vi "MainKinetics Calibration.vi"() -> ()   [LabVIEW 2017]
uses:
  <vilib>/Utility/miscctls.llb/LVRowAndColumnTypeDef.ctl
  <vilib>/Utility/sysdir.llb/System Directory Type.ctl
  <vilib>/Utility/config.llb/Read Key (String).vi
  <vilib>/Utility/config.llb/Write Key (String).vi
  <vilib>/Utility/cursorutil.llb/Set Cursor (Icon Pict).vi
  PCAN_Driver/ControlCAN.lvlib
  <vilib>/Utility/config.llb/NI_LVConfig.lvlib
panel:
  out "AO[0] 2":sgl
  out "AO[0] 1":sgl
  out "RO[1]":string
  out "AO[1]":string
  out "CC":dbl
  out "AO[0]":sgl
  out "SN From File":string
  out "ProductRev":string
  out "UUT In":u16(ring)=4 items=["BLDC  60A  P/N: 1"=1, "BLDC  30A  P/N: 2"=2, "Warrior 60A P/N: 3"=3, "Condenser Merkava P/N: 4"=4, "Condenser India P/N: 4"=5]
  out "G.Stop":bool
  out "STDBY":bool
  out "CurrentSens":bool
  out "CurrentOut":dbl
  out "Current":string
  out "VISA Current":refnum<visa-resource-name>
  out "Offset":dbl
  out "Analogtest":bool=TRUE
  out "TestinExecution":string
  out "FullSpeed2 Current":dbl
  out "FullSpeed1 Current":dbl
  out "User":string
  out "ParamVersion":string
  out "DSP Board S/N":string
  out "POWER Board S/N":string caption="DRIVER Board S/N"
  in  "EventTimeout":i32=100
  out "SpeedLimit":dbl[](array[numeric])
  out "TestArray":string[](array[string])
  out "Motor Speed RPM Serial":dbl
  out "DAQmx Device Name":tag
  out "PN":string
  out "FileName":string
  out "VenableSpeed":u16
  out "TesterVersion":string
  out "ClosePanel":bool=TRUE
  out "UUT SN Report":string
  out "Automation":bool
  out "Test Failed":bool
  out "VisualInspectionResult":bool
  out "MotorTempResult":bool
  out "VenableDirectionResult":bool
  out "VenableResult":bool
  out "ComTestResult":bool=TRUE
  out "UUT SoftwareVer":string
  out "Next SN":i32
  in  "SetSN":bool
  out "Current SN":i32
  out "FullSpeed2 Speed":dbl
  out "FullSpeed2 Current":dbl
  out "FullSpeed1 Current":dbl
  out "FullSpeed1 Speed":dbl
  out "UUT":u8
  out "CAN Status":bool
  out "Array":u64[][](array[numeric]) format="%016x"
  out "Motor Phase Current RMS":dbl
  out "Ambient Temperature":dbl
  out "Speed error":bool
  out "Commutation err":bool
  out "Under voltage/Over voltage":bool
  out "Derated drive temp":bool
  out "Motor Over temperature":bool
  out "Motor Sensor temp Fauilre":bool
  out "Drive Over temperature":bool
  out "Drive Sensor temp Failure":bool
  out "Ambient Over temp":bool
  out "Ambient Sensor temp":bool
  out "DC Voltage":dbl
  out "DC Current":dbl
  out "Power transistor Heat sink Temp.":dbl
  out "Motor Stator Temp.":dbl
  out "Motor Speed RPM":dbl
  out "ECS State":u16
  out "UUT":string="EBAY"
  in  "Logger Path":path
  in  "Report":bool
  in  "Start":bool
  in  "ATR":string[][](table)=[["Test Communication", "-", "-", "-", "-", ""], ["Set S/N", "-", "-", "-", "-", ""], ["Set Board Number", "-", "-", "-", "-", ""], [" ", "", "", "", "", ""], ["Test Communication", "-", "-", "-", "-", ""], ["Get S/N", "-", "-", "-", "", ""], ["Get Board Number", "-", "-", "-", "", ""], ["Get FW", "-", "-", "-", "", ""], ["Enable Motor", "", "", "", "", ""], ["Small position command", "", "", "", "", ""], ["Measure delta", "", "", "", "", ""], ["Velocity command", "", "", "", "", ""]]
  in  "Settings":bool
  in  "Refresh Button":bool
  out "Serial Status":bool
  in  "VISA Kinetics":refnum<visa-resource-name>="COM6"
  in  "Serial Com":bool
  in  "Help Button":bool
  out "Pannel User Message":string
  in  "Stop Button":bool
  # "Kinetics"
  # "REDLER TECHNOLOGIES LTD"
  # "ver 1.2p"
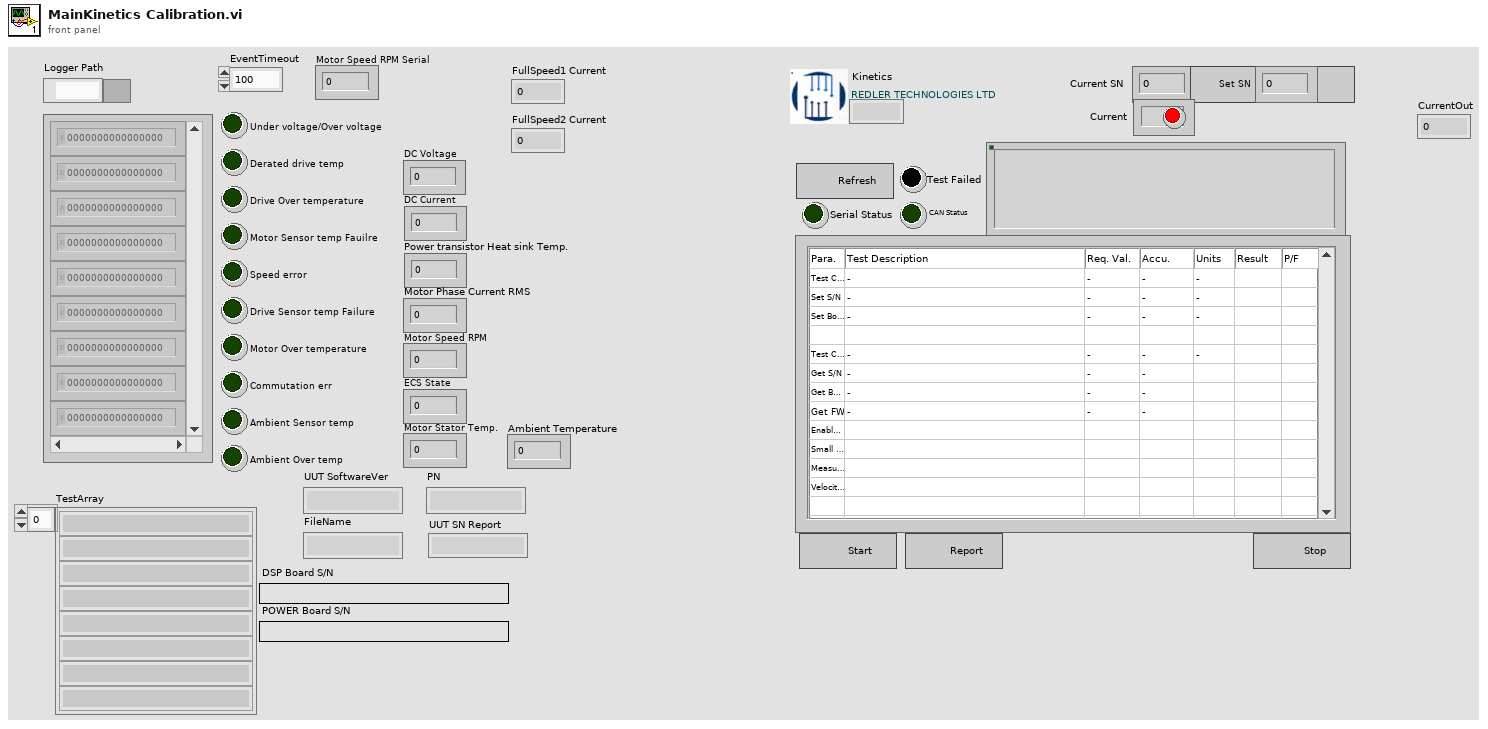
[diagram p1: front panel]
types:
  T1 = enum8{"Enabled", "Disabled", "Disabled and Grayed Out"}
  T2 = cluster{"VISA":refnum<visa-resource-name>, "TestArray":string[]}
  T3 = cluster{"ID":u32, "MSGTYPE":u8, "LEN":u8, "aDATA":u8[]}[]
  T4 = enum16{"Erase ATR Table", "Stop", "MainProgram", "Initialize"}
  T5 = typedef "NI_LVConfig.lvlib/Config Data RefNum.ctl" = refnum<k1>
  T6 = enum16{"Init", "0 ohm", "6 ohm", "13.2 ohm", "15 ohm", "25.9 ohm", "33 ohm", "Down", "Up", "Venable", "Firmware", "PowerSuply"}
  T7 = enum16{"Wait", "Exit", "VC=0", "ReadVC", "VC=1000"}
  T8 = enum16{"Stop", "Result", "FullSpeed2", "MD[1]=1", "FullSpeed1", "MD[1]=0"}
  T9 = enum16{"K15", "K16", "K17", "Venable", "Firmeware", "Fan", "Power", "120C", "110C", "100C", "90C", "80C", "70C", "60C", "50C", "40C", "30C", "25C", "20C", "10C", "0C"}
  T10 = enum8{"Term1", "Term2", "Current", "Fan", "TempCPU"}
  T11 = enum16{"Exit", "AI0/3", "AO0", "Wait", "Read", "Init"}
  T12 = enum16{"Exit", "Wait", "ReadCurrent", "ReadTemp", "Init"}
  T13 = enum16{"Init", "0 ohm", "6 ohm", "13.2 ohm", "15 ohm", "25.9 ohm", "33 ohm", "Down", "Up", "Venable", "Firmware", "PowerSuply"}[]
  T14 = typedef "LVRowAndColumnTypeDef.ctl" = cluster{"Row":i32, "Column":i32}
  T15 = enum32{"Invalid", "Standard", "Closed", "Hidden", "Minimized", "Maximized"}
  T16 = cluster{"ID":u32, "MSGTYPE":u8, "LEN":u8, "aDATA":u8[]}
  T17 = enum16{"open", "replace", "create", "open or create", "replace or create", "replace or create with confirmation"}
  T18 = typedef "ControlCAN.lvlib/DevType.ctl" = u32
  T19 = typedef "ControlCAN.lvlib/CAN Channel.ctl" = u32
  T20 = typedef "ControlCAN.lvlib/VCI_INIT_CONFIG.ctl" = cluster{"AccCode":u32, "AccMask":u32, "InitFlag":T21, "Fliter":T22, "Timing0":u8, "Timing1":u8, "Mode":T23}
  T21 = typedef "ControlCAN.lvlib/InitFlag.ctl" = u32
  T22 = typedef "ControlCAN.lvlib/Fliter.ctl" = u8
  T23 = typedef "ControlCAN.lvlib/Mode.ctl" = u8
  T24 = cluster{"DevType":T18, "DevIndex":u32, "CanIndex":T19, "VCI_INIT_CONFIG":T20}
  T25 = typedef "ControlCAN.lvlib/VCI_CAN_OBJ.ctl" = cluster{"ID":u32, "TimeStamp":u32, "TimeFlag":u8, "SendType":u8, "RemoteFlag":u8, "ExternFlag":u8, "DataLen":u8, "Data":u8[], "Reserved":u8[]}
  T26 = cluster{"Type":enum16{"接收", "发送"}, "Channel":T19, "Time":timestamp, "VCI_CAN_OBJ":T25}[]
  T27 = cluster{"Type":enum16{"接收", "发送"}, "Channel":T19, "Time":timestamp, "VCI_CAN_OBJ":T25}
  T28 = typedef "LVPoint32TypeDef.ctl" = cluster{"Horizontal":i32, "Vertical":i32}
  T29 = typedef "System Directory Type.ctl" = i32
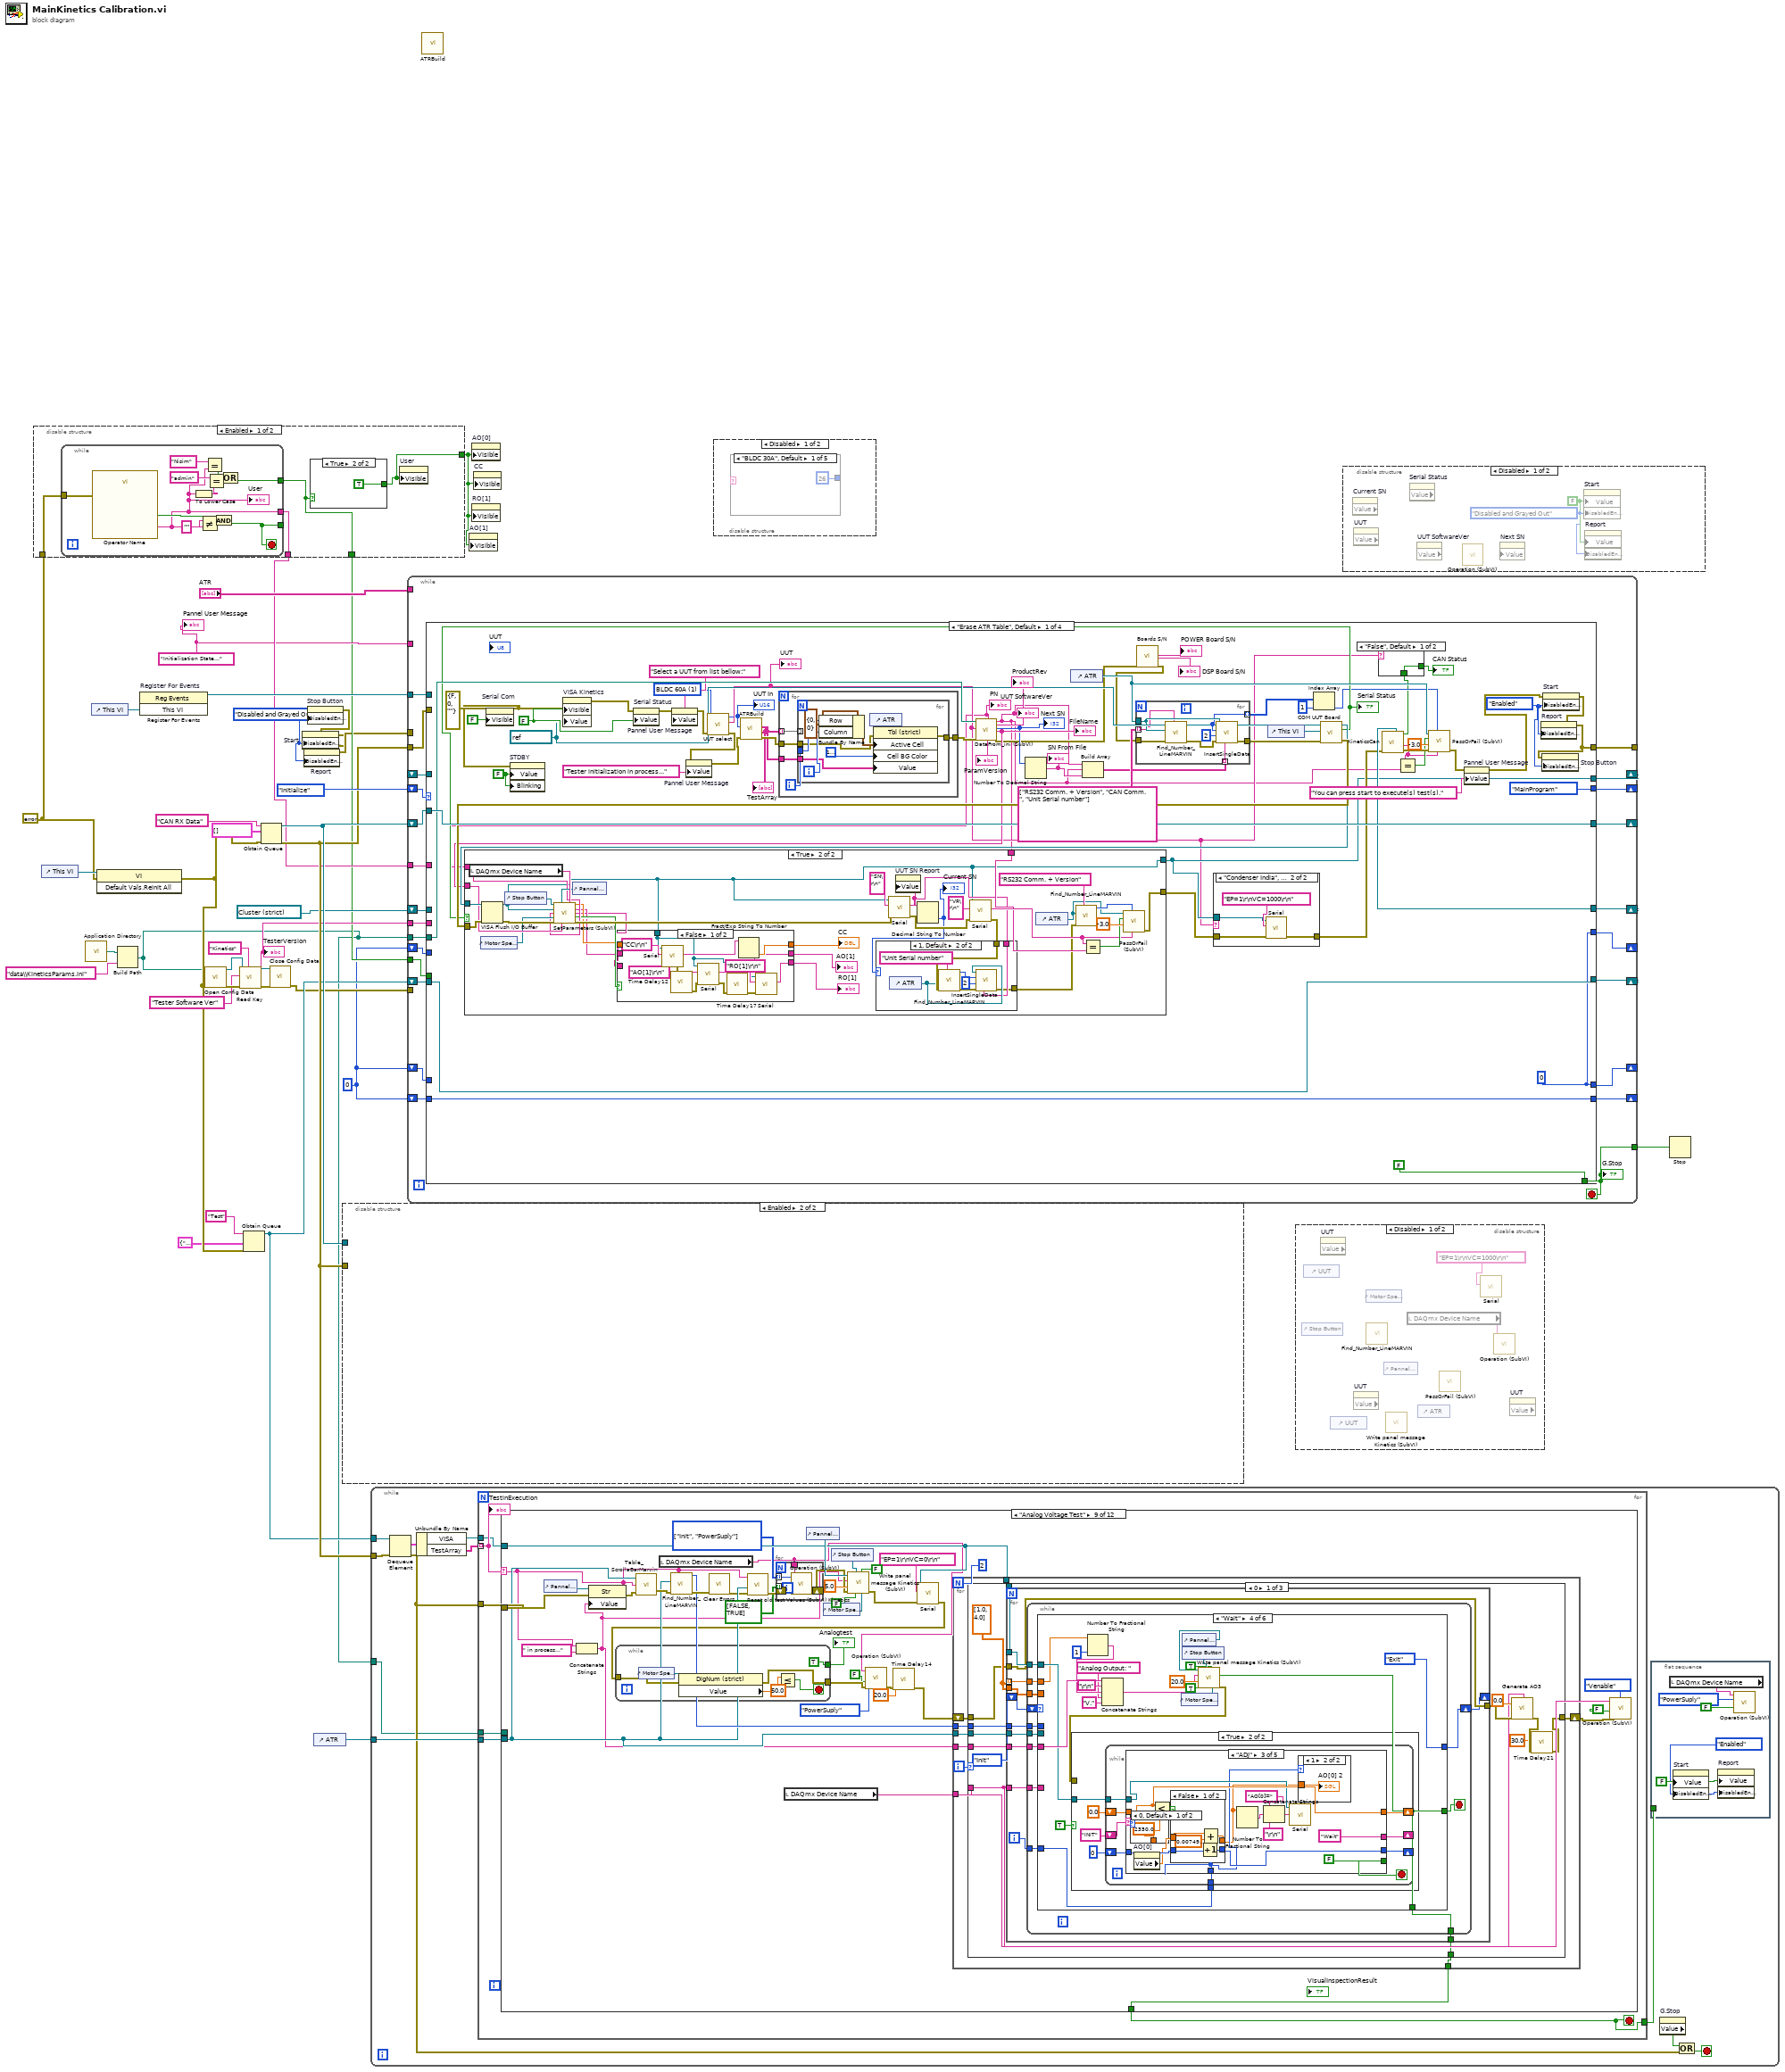
[diagram p0: block diagram]
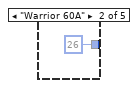
[diagram p2: hidden frame]
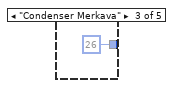
[diagram p3: hidden frame]
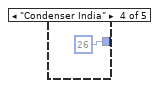
[diagram p4: hidden frame]
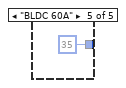
[diagram p5: hidden frame]
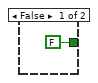
[diagram p7: hidden frame]
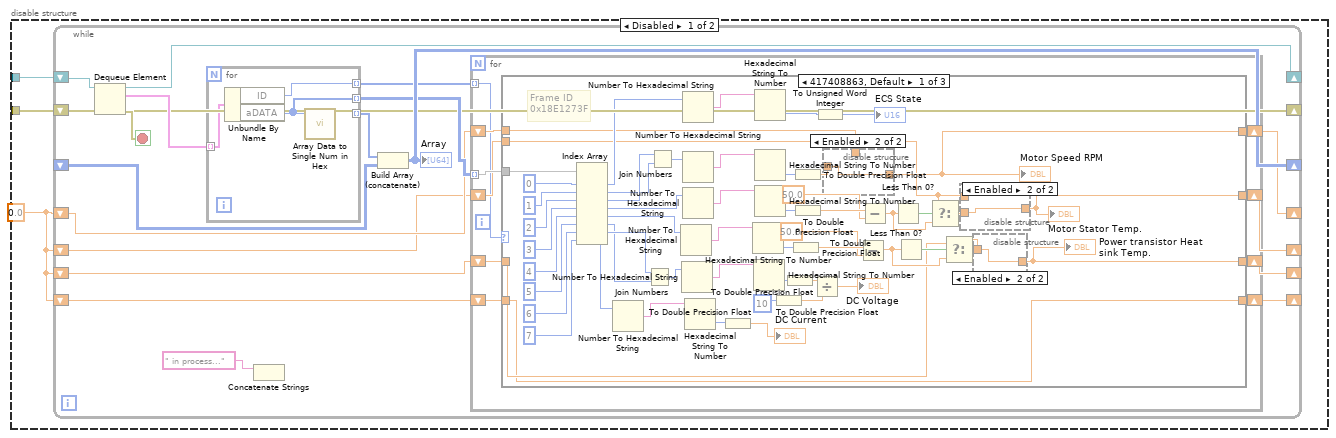
[diagram p9: hidden frame]
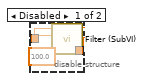
[diagram p10: hidden frame]
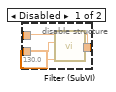
[diagram p11: hidden frame]
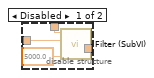
[diagram p12: hidden frame]
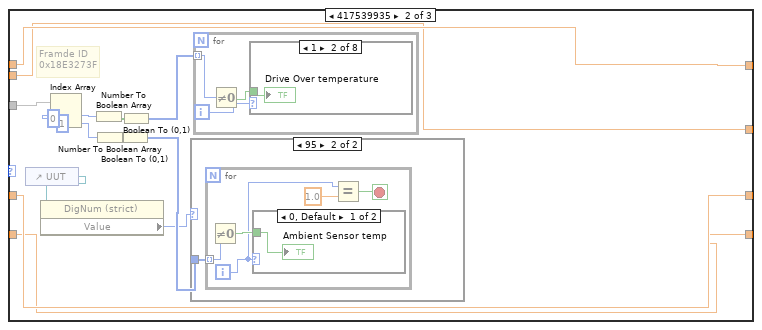
[diagram p13: hidden frame]
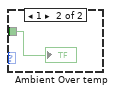
[diagram p15: hidden frame]
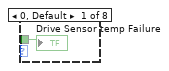
[diagram p16: hidden frame]
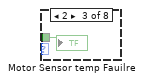
[diagram p17: hidden frame]
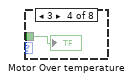
[diagram p18: hidden frame]
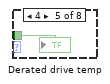
[diagram p19: hidden frame]
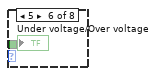
[diagram p20: hidden frame]
diagram:
  w2 = T1."Disabled and Grayed Out" ("Disabled")
  w23 = "Initialization State..."
  w9 = 0
  w12 = errorcluster {"status"=FALSE, "code"=0, "source"=""} ("error in (no error)")
  n1 = disable-structure shown="Enabled" {
    disable-tunnel: [w41 _] -> w24
    disable-tunnel: w12 -> [w40 _]
    disable-tunnel: [w39 _] -> w10
    disable-tunnel: [w38 _] -> w1
    frame Enabled {
      n2 = while {
        tunnel: [w52] -> _
        tunnel: [w45] -> w41
        tunnel: [w50] -> w39
        tunnel: w40 -> [w47]
        stop <- w52 stop-if-true
        n3 = call "Operator Name"("error in (no error)"=w47) -> ("Operator Name"=w45:string, "OK"=w53:bool)  [unwired: 16 in, 1 out]
        "User" <- w45
        n4 = To Lower Case(string=w45) -> (all lower case string=w44:string)
        n5 = Not Equal?(x=w45, y="") -> (x != y?=w54:bool)
        n6 = Equal?(x="Nisim", y=w45) -> (x = y?=w48:bool)
        n7 = Equal?(x="admin", y=w44) -> (x = y?=w51:bool)
        n8 = And(x=w53, y=w54) -> (x .and. y?=w52:bool)
        n9 = Or(x=w48, y=w51) -> (x .or. y?=w50:bool)
      }
      n10 = case shown="True" w39 {
        tunnel: [FALSE TRUE] -> w38
        frame False {
        }
        frame True {
        }
      }
      n11 = property on="User" class="Str"("Visible"=w38) -> ()  [unwired: 2 in, 2 out]
    }
    frame Disabled {
    }
  }
  n12 = control-ref of="This VI"() -> (w13:refnum<vi>)
  n13 = call <vilib>:"Application Directory.vi"() -> ("Application Directory"=w28:path)
  n14 = control-ref of="This VI"() -> (w26:refnum<vi>)
  n15 = invoke class="VI" method="Default Vals.Reinit All"(reference=w13, error in=w12) -> (error out=w11:errorcluster)  [unwired: 1 in, 2 out]
  n16 = Build Path(base path=w28, name or relative path="data\\KineticsParams.ini") -> (appended path=w6:path)
  n17 = register-events "Register For Events"(w26) -> (reference out=w25:refnum<event-registration>)  [unwired: 2 in, 1 out]
  n18 = call <vilib>:"Open Config Data.vi"("error in (no error)"=w11, "configuration file path"=w6) -> ("error out"=w21:errorcluster, "refnum"=w20:T5)  [unwired: 1 in, 7 out]
  n19 = call-poly <vilib>:"Read Key.vi"("section"="Kinetics", "error in (no error)"=w21, "key"="Tester Software Ver", "refnum"=w20) -> ("error out"=w18:errorcluster, "value"=w14:string, "refnum out"=w17:T5)  [unwired: 2 in, 3 out]
  "TesterVersion" <- w14
  n20 = Obtain Queue(name (unnamed)="Test", element data type=T2 {"VISA"="COM1", "TestArray"=[]}, error in (no error)=w11) -> (queue out=w31:refnum<queue>)  [unwired: 2 in, 2 out]
  n21 = Obtain Queue(name (unnamed)="CAN RX Data", element data type=T3 [], error in (no error)=w11) -> (queue out=w34:refnum<queue>, error out=w32:errorcluster)  [unwired: 2 in, 1 out]
  n22 = call <vilib>:"Close Config Data.vi"("error in (no error)"=w18, "refnum"=w17) -> ("error out"=w16:errorcluster)  [unwired: 8 in, 1 out]
  n23 = property on="Stop Button" class="Bool (strict)"("DisabledEnum"=w2) -> (error out=w3:errorcluster)  [unwired: 2 in, 1 out]
  n24 = property on="Start" class="Bool (strict)"(error in=w3, "DisabledEnum"=w2) -> (error out=w4:errorcluster)  [unwired: 1 in, 1 out]
  n25 = property on="Report" class="Bool (strict)"(error in=w4, "DisabledEnum"=w2) -> (error out=w5:errorcluster)  [unwired: 1 in, 1 out]
  n26 = control-ref of="ATR"() -> (w22:refnum<vi>)
  n27 = disable-structure shown="Enabled" {
    disable-tunnel: w34 -> [w58 _]
    disable-tunnel: w32 -> [w57 _]
    frame Disabled {
      w56 = 0.0
      n28 = while {
        shift-right: [w75] -> _
        shift-left: w58 -> [w77]
        shift-right: [w73] -> _
        shift-left: _ -> [w74]
        shift-right: [w69] -> _
        shift-left: w57 -> [w69]
        shift-right: [w67] -> _
        shift-left: w56 -> [w68]
        shift-right: [w66] -> _
        shift-left: w56 -> [w65]
        shift-right: [w64] -> _
        shift-left: w56 -> [w63]
        shift-right: [w62] -> _
        shift-left: w56 -> [w61]
        stop <- w76 stop-if-true
        n29 = Dequeue Element(queue=w77, error in (no error)=w69) -> (queue out=w75:refnum<queue>, element=w70:T3, error out=w76:errorcluster)  [unwired: 1 in, 1 out]
        n30 = for {
          tunnel: [w223] -> w72 mode=indexing
          tunnel: w70 -> [w222] mode=indexing
          tunnel: [w221] -> w71 mode=indexing
          tunnel: [w220] -> w60 mode=indexing
          n31 = Unbundle By Name(w222) -> ("ID"=w220:u32, "aDATA"=w221:u8[])
          n32 = call "Array Data to Single Num in Hex.vi"("aDATA"=w221) -> ("Numeric"=w223:u64)  [unwired: 10 in]
        }
        n33 = Concatenate Strings(" in process..." ("Strin")) -> ()  [unwired: 1 in, 1 out]
        n34 = Build Array (concatenate)(w72, w74) -> (w73:u64[][])
        "Array" <- w73
        n35 = for {
          tunnel: w71 -> [w87] mode=indexing
          shift-right: [w85] -> w67
          shift-left: w68 -> [w86]
          shift-right: [w84] -> w66
          shift-left: w65 -> [w83]
          shift-right: [w82] -> w64
          shift-left: w63 -> [w81]
          shift-right: [w80] -> w62
          shift-left: w61 -> [w79]
          tunnel: w60 -> [w78] mode=indexing
          n36 = case shown="417408863, Default" w78 {
            tunnel: w87 -> [w124 w172 w210]
            tunnel: w86 -> [w98 w161 w199]
            tunnel: [w97 w161 w199] -> w85
            tunnel: [w94 w160 w198] -> w84
            tunnel: w83 -> [w93 w160 w198]
            tunnel: [w90 w159 w197] -> w82
            tunnel: w81 -> [w89 w159 w197]
            tunnel: [w88 w158 w193] -> w80
            tunnel: w79 -> [w88 w158 w192]
            frame 417408863, Default {
              # "Frame ID\n0x18E1273F"
              n37 = Index Array(array=w124, index #1=0 ("index"), index #2=1 ("index"), index #3=2 ("index"), index #4=3 ("index"), index #5=4 ("index"), index #6=5 ("index"), index #7=6 ("index"), index #8=7 ("index")) -> (element #1=w108:u8, element #2=w110:u8, element #3=w111:u8, element #4=w115:u8, element #5=w118:u8, element #6=w122:u8, element #7=w123:u8, element #8=w121:u8)
              n38 = Number To Hexadecimal String(2:w121) -> (0:w135:string)  [unwired: 1 in]
              n39 = Join Numbers(hi=w123, lo=w122) -> ((hi.lo)=w142:u16)
              n40 = Join Numbers(hi=w111, lo=w110) -> ((hi.lo)=w112:u16)
              n41 = Number To Hexadecimal String(2:w118) -> (0:w119:string)  [unwired: 1 in]
              n42 = Number To Hexadecimal String(2:w142) -> (0:w141:string)  [unwired: 1 in]
              n43 = Number To Hexadecimal String(2:w108) -> (0:w109:string)  [unwired: 1 in]
              n44 = Number To Hexadecimal String(2:w112) -> (0:w113:string)  [unwired: 1 in]
              n45 = Number To Hexadecimal String(2:w115) -> (0:w116:string)  [unwired: 1 in]
              n46 = Hexadecimal String To Number(string=w135) -> (number=w134:u32)  [unwired: 2 in, 1 out]
              n47 = To Double Precision Float(number=w134) -> (double precision float=→"DC Current":dbl)
              n48 = Hexadecimal String To Number(string=w119) -> (number=w120:u32)  [unwired: 2 in, 1 out]
              n49 = Hexadecimal String To Number(string=w141) -> (number=w140:u32)  [unwired: 2 in, 1 out]
              n50 = Hexadecimal String To Number(string=w109) -> (number=w106:u32)  [unwired: 2 in, 1 out]
              n51 = Hexadecimal String To Number(string=w113) -> (number=w114:u32)  [unwired: 2 in, 1 out]
              n52 = Hexadecimal String To Number(string=w116) -> (number=w117:u32)  [unwired: 2 in, 1 out]
              n53 = To Double Precision Float(number=u32 10 ("y")) -> (double precision float=w138:dbl)
              n54 = To Double Precision Float(number=w140) -> (double precision float=w137:dbl)
              n55 = To Double Precision Float(number=w120) -> (double precision float=w103:dbl)
              n56 = To Double Precision Float(number=w114) -> (double precision float=w99:dbl)
              n57 = To Double Precision Float(number=w117) -> (double precision float=w105:dbl)
              n58 = Divide(x=w137, y=w138) -> (x/y=→"DC Voltage":dbl)
              n59 = To Unsigned Word Integer(number=w106) -> (unsigned 16bit integer=→"ECS State":u16)
              n60 = disable-structure shown="Enabled" {
                disable-tunnel: w99 -> [w156 w157]
                disable-tunnel: w98 -> [w155 _]
                disable-tunnel: [w153 w157] -> w97
                frame Disabled {
                  n61 = call "Filter (SubVI).vi"("Delta"=5000.0, "NewVal"=w156, "OldVal"=w155) -> ("Val"=w153:dbl)  [unwired: 8 in]
                }
                frame Enabled {
                }
              }
              "Motor Speed RPM" <- w97
              n62 = Subtract(x=w103, y=50.0 ("x")) -> (x-y=w92:dbl)
              n63 = Subtract(x=w105, y=50.0 ("x")) -> (x-y=w95:dbl)
              n64 = Less Than 0?(x=w95) -> (x < 0?=w101:bool)
              n65 = Less Than 0?(x=w92) -> (x < 0?=w100:bool)
              n66 = Select(t=w93, s=w101, f=w95) -> (s? t:f=w96:dbl)
              n67 = Select(t=w89, s=w100, f=w92) -> (s? t:f=w91:dbl)
              n68 = disable-structure shown="Enabled" {
                disable-tunnel: w96 -> [w151 w152]
                disable-tunnel: [w150 w152] -> w94
                disable-tunnel: w93 -> [w149 _]
                frame Disabled {
                  n69 = call "Filter (SubVI).vi"("Delta"=130.0, "NewVal"=w151, "OldVal"=w149) -> ("Val"=w150:dbl)  [unwired: 8 in]
                }
                frame Enabled {
                }
              }
              "Motor Stator Temp." <- w94
              n70 = disable-structure shown="Enabled" {
                disable-tunnel: w91 -> [w146 w147]
                disable-tunnel: [w144 w147] -> w90
                disable-tunnel: w89 -> [w143 _]
                frame Disabled {
                  n71 = call "Filter (SubVI).vi"("Delta"=100.0, "NewVal"=w146, "OldVal"=w143) -> ("Val"=w144:dbl)  [unwired: 8 in]
                }
                frame Enabled {
                }
              }
              "Power transistor Heat sink Temp." <- w90
            }
            frame 417539935 {
              # "Framde ID\n0x18E3273F"
              n72 = control-ref of="UUT"() -> (w162:refnum<vi>)
              n73 = property on="Property Node" class="DigNum (strict)"(reference=w162) -> ("Value"=w163:u8)  [unwired: 1 in, 2 out]
              n74 = Index Array(array=w172, index #1=0 ("index"), index #2=1 ("index")) -> (element #1=w170:u8, element #2=w165:u8)
              n75 = Number To Boolean Array(number=w170) -> (Boolean array=w169:bool[])
              n76 = Number To Boolean Array(number=w165) -> (Boolean array=w167:bool[])
              n77 = Boolean To (0,1)(Boolean=w167) -> (0, 1=w164:i16[])
              n78 = Boolean To (0,1)(Boolean=w169) -> (0, 1=w168:i16[])
              n79 = case shown="95" w163 {
                tunnel: w164 -> [_ w173]
                frame 0, Default {
                }
                frame 95 {
                  n80 = for {
                    tunnel: w173 -> [w178] mode=indexing
                    i -> [w174]
                    stop <- w176 stop-if-true
                    n81 = Not Equal To 0?(x=w178) -> (x != 0?=w177:bool)
                    n82 = case shown="0, Default" w174 {
                      tunnel: w177 -> [w179 w180]
                      frame 0, Default {
                        "Ambient Sensor temp" <- w179
                      }
                      frame 1 {
                        "Ambient Over temp" <- w180
                      }
                    }
                    n83 = Equal?(x=w174, y=1.0) -> (x = y?=w176:bool)
                  }
                }
              }
              n84 = for {
                tunnel: w168 -> [w182] mode=indexing
                i -> [w183]
                n85 = Not Equal To 0?(x=w182) -> (x != 0?=w181:bool)
                n86 = case shown="1" w183 {
                  tunnel: w181 -> [w184 w185 w186 w187 w188 w189 w190 w191]
                  frame 0, Default {
                    "Drive Sensor temp Failure" <- w184
                  }
                  frame 1 {
                    "Drive Over temperature" <- w185
                  }
                  frame 2 {
                    "Motor Sensor temp Fauilre" <- w186
                  }
                  frame 3 {
                    "Motor Over temperature" <- w187
                  }
                  frame 4 {
                    "Derated drive temp" <- w188
                  }
                  frame 5 {
                    "Under voltage/Over voltage" <- w189
                  }
                  frame 6 {
                    "Commutation err" <- w190
                  }
                  frame 7 {
                    "Speed error" <- w191
                  }
                }
              }
            }
            frame 417474399 {
              # "Frame ID\n0x18E2273F"
              n87 = Index Array(array=w210, index #1=0 ("index"), index #2=1 ("index")) -> (element #1=w207:u8, element #2=w204:u8)
              n88 = disable-structure shown="Enabled" {
                disable-tunnel: [w218 w219] -> w208
                disable-tunnel: w207 -> [w217 w219]
                frame Disabled {
                  n89 = Number To Hexadecimal String(2:w217) -> (0:w216:string)  [unwired: 1 in]
                  n90 = Hexadecimal String To Number(string=w216) -> (number=w218:u32)  [unwired: 2 in, 1 out]
                }
                frame Enabled {
                }
              }
              n91 = Number To Hexadecimal String(2:w204) -> (0:w202:string)  [unwired: 1 in]
              n92 = Hexadecimal String To Number(string=w202) -> (number=w203:u32)  [unwired: 2 in, 1 out]
              n93 = To Double Precision Float(number=w203) -> (double precision float=w201:dbl)
              n94 = To Double Precision Float(number=w208) -> (double precision float=→"Motor Phase Current RMS":dbl)
              n95 = Subtract(x=w201, y=50.0) -> (x-y=w195:dbl)
              n96 = Less Than 0?(x=w195) -> (x < 0?=w196:bool)
              n97 = Select(t=w192, s=w196, f=w195) -> (s? t:f=w194:dbl)
              n98 = disable-structure shown="Disabled" {
                disable-tunnel: w194 -> [w214 w215]
                disable-tunnel: [w212 w215] -> w193
                disable-tunnel: w192 -> [w211 _]
                frame Disabled {
                  n99 = call "Filter (SubVI).vi"("Delta"=65.0, "NewVal"=w214, "OldVal"=w211) -> ("Val"=w212:dbl)  [unwired: 8 in]
                }
                frame Enabled {
                }
              }
              "Ambient Temperature" <- w193
            }
          }
        }
      }
    }
    frame Enabled {
    }
  }
  n100 = while {
    tunnel: w22 -> [w234]
    tunnel: w32 -> [w232]
    tunnel: w31 -> [w233]
    tunnel: w6 -> [w224]
    stop <- w226 stop-if-true
    n101 = Dequeue Element(queue=w233, error in (no error)=w232) -> (element=w231:T2, error out=w229:errorcluster)  [unwired: 1 in, 2 out]
    n102 = Unbundle By Name(w231) -> ("VISA"=w230:refnum<visa-resource-name>, "TestArray"=w227:string[])
    n103 = for {
      tunnel: w227 -> [w244] mode=indexing
      tunnel: w230 -> [w243]
      tunnel: w234 -> [w242]
      tunnel: w229 -> [w245]
      tunnel: [w241] -> w228
      tunnel: w224 -> [w240]
      stop <- w241 stop-if-true
      n104 = case shown="\"Analog Voltage Test\"" w244 {
        selector: w244 -> [_ w263 w693 w1167 w1306 w1453 w1538 w1622 w1710 w2205 w2346 _]
        tunnel: w242 -> [_ w256 _ _ w1300 w1447 w1532 w1616 w1711 w2213 w2345 w2421]
        tunnel: w245 -> [_ w266 _ _ w1313 w1452 w1537 w1621 w1712 w2220 w2333 w2425]
        tunnel: w243 -> [_ w259 w692 w1166 w1303 w1441 w1529 w1607 w1693 w2206 w2331 _]
        tunnel: [TRUE ("Stopped") w251 w691 w1156 w1296 w1436 w1522 w1609 w1705 w2204 FALSE ("Stopped") _] -> w241
        tunnel: w240 -> [_ _ _ _ _ _ _ _ _ _ w2332 _]
        frame "", Default {
        }
        frame "Comm. & Motor Test" {
          n105 = control-ref of="Pannel User Message"() -> (w267:refnum<vi>)
          n106 = Concatenate Strings(w263, " in process..." ("string")) -> (w258:string)
          n107 = property class="Str"(reference=w267, error in=w266, "Value"=w258) -> (error out=w265:errorcluster)  [unwired: 1 out]
          n108 = call "Table_ScrollaBarMarvin.vi"("error in"=w265, "Line to focus"=w263, "reference in"=w256) -> ("error out"=w262:errorcluster)  [unwired: 2 out]
          n109 = call "Find_Number_LineMARVIN.vi"("Test Paragraph"=w263, "error in"=w262, "TableIn"=w256) -> ("error out"=w268:errorcluster, "Line number"=w247:i32)  [unwired: 2 in, 2 out]
          n110 = property on="UUT" class="Str"() -> ("Value"=w255:string)  [unwired: 2 in, 2 out]
          n111 = Concatenate Strings("- Set the FIREWERE switch to OFF position." ("Screen Line"), "- Set the VENABLE switch to ON position." ("Screen Line")) -> (w252:string)
          n112 = call <vilib>:"Clear Errors.vi"("error in (no error)"=w268) -> ("error out"=w261:errorcluster)  [unwired: 5 in, 1 out]
          n113 = Add(x=3, y=w247) -> (x+y=w257:i32)
          n114 = call "Reset old test Values (SubVI) Kinetics.vi"("error in"=w261, "Atr in"=w256, "Test Paragraph"=w263) -> ("error out"=w250:errorcluster)  [unwired: 6 in, 2 out]
          n115 = case shown="\"Condenser India\", \"Condenser Merkava\"" w255 {
            tunnel: w252 -> [_ w690]
            tunnel: w250 -> [w688 w689]
            tunnel: [w688 w689] -> w249
            frame "False", Default {
            }
            frame "Condenser India", "Condenser Merkava" {
              n116 = One Button Dialog(message=w690) -> ()  [unwired: 1 in, 1 out]
            }
          }
          n117 = for {
            N: 2 -> [_]
            tunnel: w259 -> [w276]
            tunnel: w258 -> [w275]
            tunnel: w257 -> [w274]
            tunnel: w256 -> [w273]
            tunnel: [w272] -> w251
            tunnel: w249 -> [w271]
            tunnel: w247 -> [w269]
            i -> [w270]
            n118 = case shown="0, Default" w270 {
              tunnel: w276 -> [w292 w391]
              tunnel: w275 -> [w291 w390]
              tunnel: w274 -> [w290 _]
              tunnel: w273 -> [w284 w388]
              tunnel: [w289 w392] -> w272
              tunnel: w271 -> [w280 _]
              tunnel: w269 -> [w286 _]
              frame 0, Default {
                n119 = Increment(x=w286) -> (x+1=w279:i32)
                n120 = property on="Serial Status" class="Bool (strict)"() -> ("Value"=w288:bool)  [unwired: 2 in, 2 out]
                n121 = property on="UUT SoftwareVer" class="Str"() -> ("Value"=w277:string)  [unwired: 2 in, 2 out]
                n122 = call "PassOrFail (SubVI).vi"("String Res"=w277, "index (row)"=w279, "error in (no error)"=w280, "Data in"=-3.0, "Pass?Fail"=w288, "Table in"=w284) -> ("error out"=w282:errorcluster)  [unwired: 5 in]
                n123 = Increment(x=w279) -> (x+1=w278:i32)
                n124 = property on="CAN Status" class="Bool (strict)"() -> ("Value"=w283:bool)  [unwired: 2 in, 2 out]
                n125 = call "PassOrFail (SubVI).vi"("String Res"=w277, "index (row)"=w278, "error in (no error)"=w282, "Data in"=-3.0, "Pass?Fail"=w283, "Table in"=w284) -> ("error out"=w281:errorcluster)  [unwired: 5 in]
                n126 = disable-structure shown="Disabled" {
                  disable-tunnel: w292 -> [w300 _]
                  disable-tunnel: w291 -> [w299 _]
                  disable-tunnel: w290 -> [w297 _]
                  disable-tunnel: [w295 _] -> w289
                  disable-tunnel: w284 -> [w294 _]
                  disable-tunnel: w281 -> [w293 _]
                  frame Disabled {
                    n127 = while {
                      shift-right: [w311] -> _
                      shift-left: T7."VC=1000" -> [w314]
                      tunnel: w293 -> [w313]
                      tunnel: w300 -> [w312]
                      tunnel: w299 -> [w310]
                      shift-right: [w307] -> w296
                      shift-left: bool[] [FALSE, FALSE] -> [w308]
                      tunnel: w297 -> [w306]
                      tunnel: w294 -> [w305]
                      tunnel: [w303] -> w295
                      i -> [w309]
                      stop <- w304 stop-if-true
                      n128 = case shown="\"Exit\", Default" w314 {
                        tunnel: w313 -> [_ w337 _ w368 _]
                        tunnel: w312 -> [w317 w335 w344 w372 _]
                        tunnel: [T7."Exit" T7."Wait" w341 T7."Wait" T7."ReadVC"] -> w311
                        tunnel: w310 -> [_ _ _ _ w380]
                        tunnel: [TRUE FALSE FALSE FALSE FALSE] -> w304
                        tunnel: w309 -> [_ _ w342 _ w375]
                        tunnel: w308 -> [w316 w332 w340 w370 w377]
                        tunnel: [w316 w332 w339 w370 w377] -> w307
                        tunnel: w306 -> [w325 _ _ _ _]
                        tunnel: w305 -> [w327 _ _ _ _]
                        tunnel: [_ _ _ _ w374] -> w303
                        frame "Exit", Default {
                          n129 = And Array Elements(Boolean array=w316) -> (logical AND=w320:bool)
                          n130 = local read "DAQmx Device Name"() -> (w324:tag)
                          n131 = Select(t="OK", s=w320, f="Failed") -> (s? t:f=w326:string)
                          n132 = call "PassOrFail (SubVI).vi"("String Res"=w326, "index (row)"=w325, "Data in"=-3.0, "Pass?Fail"=w320, "Table in"=w327) -> ("error out"=w315:errorcluster)  [unwired: 6 in]
                          n133 = call "Serial.vi"("error in (no error)"=w315, "write buffer"="EP=1\r\nVC=0\r\n", "VISA resource name"=w317) -> ("error out"=w318:errorcluster)  [unwired: 7 in, 1 out]
                          n134 = call "Operation (SubVI).vi"("error in (no error)"=w318, "On/Off"=FALSE, "Operation"=T6."Venable", "DAQmx Device Name"=w324) -> ()  [unwired: 7 in, 1 out]
                        }
                        frame "VC=0" {
                          n135 = call "Serial.vi"("error in (no error)"=w337, "write buffer"="EP=1\r\nVC=0\r\n", "VISA resource name"=w335) -> ()  [unwired: 7 in, 2 out]
                        }
                        frame "ReadVC" {
                          n136 = call "Serial.vi"("write buffer"="VC\r\n", "VISA resource name"=w344) -> ("read buffer"=w343:string)  [unwired: 8 in, 1 out]
                          n137 = case shown="5, Default" w342 {
                            tunnel: w343 -> [w353 w359]
                            tunnel: [T7."VC=0" T7."Exit"] -> w341
                            tunnel: w340 -> [w348 w358]
                            tunnel: [w346 w355] -> w339
                            frame 2 {
                              n138 = Decimal String To Number(string=w353) -> (number=w352:i32)  [unwired: 2 in, 1 out]
                              n139 = In Range and Coerce(upper limit=11000, x=w352, lower limit=10500) -> (In Range?=w347:bool)  [unwired: 1 out]
                              n140 = Replace Array Subset(array=w348, new element=w347, index=0) -> (w346:bool[])
                            }
                            frame 5, Default {
                              n141 = Decimal String To Number(string=w359) -> (number=w362:i32)  [unwired: 2 in, 1 out]
                              n142 = In Range and Coerce(upper limit=100, x=w362, lower limit=0) -> (In Range?=w356:bool)  [unwired: 1 out]
                              n143 = Replace Array Subset(array=w358, new element=w356, index=1) -> (w355:bool[])
                            }
                          }
                        }
                        frame "VC=1000" {
                          n144 = local read "DAQmx Device Name"() -> (w369:tag)
                          n145 = call "Operation (SubVI).vi"("error in (no error)"=w368, "On/Off"=TRUE, "Operation"=T6."Venable", "DAQmx Device Name"=w369) -> ("error out"=w367:errorcluster)  [unwired: 7 in]
                          n146 = call "Serial.vi"("error in (no error)"=w367, "write buffer"="EP=1\r\nVC=10800\r\n", "VISA resource name"=w372) -> ()  [unwired: 7 in, 2 out]
                        }
                        frame "Wait" {
                          n147 = case shown="4" w375 {
                            tunnel: [59.0 ("Time to wait") 59.0 ("Time to wait")] -> w381
                            frame 4 {
                            }
                            frame 1, Default {
                            }
                          }
                          n148 = control-ref of="Motor Speed RPM Serial"() -> (w385:refnum<vi>)
                          n149 = control-ref of="Pannel User Message"() -> (w384:refnum<vi>)
                          n150 = control-ref of="Stop Button"() -> (w379:refnum<vi>)
                          n151 = call "Write panel message Kinetics (SubVI).vi"(4:"rpm"=w385, 5:"rpm"=TRUE ("rpm"), "PrintTime"=TRUE, "Stop"=w379, "Time to wait"=w381, "Strin"=w380, "String in"=w384) -> ("Stopped"=w374:bool)  [unwired: 2 in, 2 out]
                        }
                      }
                    }
                    n152 = And Array Elements(Boolean array=w296) -> (logical AND=→"ComTestResult":bool)
                  }
                  frame Enabled {
                  }
                }
              }
              frame 1 {
                n153 = case shown="True" TRUE {
                  tunnel: [_ w414] -> w392
                  tunnel: w391 -> [w393 w413]
                  tunnel: w390 -> [_ w411]
                  tunnel: w388 -> [w399 _]
                  frame False {
                    n154 = Two Button Dialog(message="Is the motor run in he right direction?", 1:"No" ("F button name (\"Cancel\")"), 2:"Yes" ("T button name (\"OK\")")) -> (T button?=w395:bool)
                    n155 = call "Find_Number_LineMARVIN.vi"("Test Paragraph"="Motor Direction", "TableIn"=w399) -> ("Line number"=w410:i32)  [unwired: 3 in, 3 out]
                    n156 = Select(t="OK", s=w395, f="Failed") -> (s? t:f=w409:string)
                    n157 = call "PassOrFail (SubVI).vi"("String Res"=w409, "index (row)"=w410, "Data in"=-3.0, "Pass?Fail"=w395, "Table in"=w399) -> ("error out"=w407:errorcluster)  [unwired: 6 in]
                    n158 = call "Serial.vi"("error in (no error)"=w407, "write buffer"="EP=1\r\nVC=0\r\n", "VISA resource name"=w393) -> ("error out"=w408:errorcluster)  [unwired: 7 in, 1 out]
                    n159 = local read "DAQmx Device Name"() -> (w394:tag)
                    n160 = call "Operation (SubVI).vi"("error in (no error)"=w408, "On/Off"=FALSE, "Operation"=T6."Venable", "DAQmx Device Name"=w394) -> ()  [unwired: 7 in, 1 out]
                  }
                  frame True {
                    n161 = property on="UUT" class="Str"() -> ("Value"=w416:string)  [unwired: 2 in, 2 out]
                    n162 = case shown="\"BLDC 60A\"" w416 {
                      tunnel: [26 26 26 26 40] -> w417
                      tunnel: [_ _ _ _ 56] -> w418
                      tunnel: [_ _ _ _ "10800"] -> w412
                      frame "BLDC 30A", Default {
                      }
                      frame "Warrior 60A" {
                      }
                      frame "Condenser Merkava" {
                      }
                      frame "Condenser India" {
                      }
                      frame "BLDC 60A" {
                      }
                    }
                    n163 = local read "DAQmx Device Name"() -> (w422:tag)
                    n164 = control-ref of="Stop Button"() -> (w419:refnum<vi>)
                    n165 = control-ref of="ATR"() -> (w423:refnum<vi>)
                    n166 = control-ref of="Pannel User Message"() -> (w420:refnum<vi>)
                    n167 = control-ref of="Motor Speed RPM Serial"() -> (w421:refnum<vi>)
                    n168 = while {
                      shift-right: [w436] -> _
                      shift-left: T8."MD[1]=0" -> [w437]
                      tunnel: w419 -> [w435]
                      tunnel: w420 -> [w434]
                      tunnel: w421 -> [w433]
                      tunnel: w422 -> [w432]
                      tunnel: w417 -> [w431]
                      tunnel: w418 -> [w430]
                      tunnel: w423 -> [w429]
                      tunnel: [w424] -> w414
                      tunnel: w413 -> [w427]
                      tunnel: w412 -> [w426]
                      tunnel: w411 -> [w425]
                      stop <- w428 stop-if-true
                      n169 = case shown="\"FullSpeed2\"" w437 {
                        tunnel: [T8."Stop" T8."Stop" w495 w566 w606 w680] -> w436
                        tunnel: [TRUE w457 FALSE FALSE FALSE FALSE] -> w428
                        tunnel: w435 -> [_ w447 w480 w546 w592 w657]
                        tunnel: w434 -> [_ w446 w481 w547 w593 w658]
                        tunnel: w433 -> [_ w445 w482 w541 w595 w652]
                        tunnel: w432 -> [_ w449 w485 w533 _ w644]
                        tunnel: w431 -> [_ _ _ _ w594 _]
                        tunnel: w430 -> [_ _ w479 _ _ _]
                        tunnel: w429 -> [_ w458 _ _ _ _]
                        tunnel: w427 -> [w438 w452 w475 w528 w590 w649]
                        tunnel: w426 -> [_ _ w474 _ w587 _]
                        tunnel: w425 -> [_ _ w472 w538 w585 w648]
                        tunnel: [_ w442 w471 w529 w584 w639] -> w424
                        frame "Stop", Default {
                          n170 = call "Serial.vi"("write buffer"="EP=1\r\nVC=0\r\nMD[1]=1\r\n", "VISA resource name"=w438) -> ()  [unwired: 8 in, 2 out]
                        }
                        frame "Result" {
                          n171 = property on="FullSpeed2 Current" class="DigNum (strict)"() -> ("Value"=w463:dbl)  [unwired: 2 in, 2 out]
                          n172 = property on="FullSpeed1 Current" class="DigNum (strict)"() -> ("Value"=w462:dbl)  [unwired: 2 in, 2 out]
                          n173 = Subtract(x=w463, y=w462) -> (x-y=w470:dbl)
                          n174 = call "Find_Number_LineMARVIN.vi"("Test Paragraph"="Motor Direction", "TableIn"=w458) -> ("Line number"=w467:i32)  [unwired: 3 in, 3 out]
                          n175 = Absolute Value(x=w470) -> (abs(x)=w465:dbl)
                          n176 = Greater Or Equal?(x=w465, y=7.0) -> (x >= y?=w443:bool)
                          n177 = Not(x=w443) -> (.not. x?=w442:bool)
                          n178 = Select(t="OK", s=w443, f="Failed") -> (s? t:f=w459:string)
                          n179 = call "PassOrFail (SubVI).vi"("String Res"=w459, "index (row)"=w467, "Data in"=-3.0, "Pass?Fail"=w443, "Table in"=w458) -> ("error out"=w451:errorcluster)  [unwired: 6 in]
                          n180 = call "Serial.vi"("error in (no error)"=w451, "write buffer"="EP=1\r\nVC=0\r\n", "VISA resource name"=w452) -> ("error out"=w456:errorcluster)  [unwired: 7 in, 1 out]
                          n181 = call "Operation (SubVI).vi"("error in (no error)"=w456, "On/Off"=FALSE, "Operation"=T6."Venable", "DAQmx Device Name"=w449) -> ("error out"=w448:errorcluster)  [unwired: 7 in]
                          n182 = Not(x=TRUE) -> (.not. x?=w457:bool)
                          n183 = call "Wait Motor 0 RPM (SubVI).vi"("Strin"="Please wait untill RPM = 0.", "error in (no error)"=w448, "Motor Speed RPM Serial"=w445, "Pannel User Message"=w446, "Stop"=w447) -> ()  [unwired: 6 in, 1 out]
                        }
                        frame "FullSpeed2" {
                          n184 = Search and Replace String(input string="EP=1\r\nVC=0\r\n" ("write buffer"), search string="0", replace string=w474) -> (result string=w478:string)  [unwired: 5 in, 3 out]
                          n185 = call "Serial.vi"("write buffer"=w478, "VISA resource name"=w475) -> ("error out"=w473:errorcluster)  [unwired: 8 in, 1 out]
                          n186 = Concatenate Strings(w472, "\nFull speed operation " ("string")) -> (w489:string)
                          n187 = call "Write panel message Kinetics (SubVI).vi"(4:"rpm"=w482, 5:"rpm"=TRUE ("rpm"), "PrintTime"=TRUE, "Stop"=w480, "error in (no error)"=w473, "Time to wait"=45.0, "Strin"=w489, "String in"=w481) -> ("error out"=w492:errorcluster, "Stopped"=w484:bool)  [unwired: 1 in, 1 out]
                          n188 = flat-sequence {
                            tunnel: w492 -> [w499]
                            tunnel: [w499] -> w491
                            tunnel: [w498] -> w490
                            frame #0 {
                              n189 = call <vilib>:"High Resolution Relative Seconds.vi"() -> ("relative seconds"=w498:dbl)
                            }
                          }
                          n190 = while {
                            tunnel: w491 -> [_]
                            tunnel: [w522] -> _
                            tunnel: w479 -> [w526]
                            tunnel: w490 -> [w524]
                            tunnel: w489 -> [w520]
                            tunnel: w482 -> [w513]
                            tunnel: w485 -> [_]
                            tunnel: w484 -> [w517]
                            tunnel: [w508] -> w483
                            tunnel: w481 -> [w516]
                            tunnel: w480 -> [w515]
                            tunnel: [w511] -> w471
                            stop <- w527 stop-if-true
                            n191 = call <vilib>:"High Resolution Relative Seconds.vi"() -> ("relative seconds"=w525:dbl)
                            n192 = local read "CurrentOut"() -> (w510:dbl)
                            n193 = property class="DigNum (strict)"(reference=w513) -> ("Value"=w502:dbl)  [unwired: 1 in, 2 out]
                            n194 = Subtract(x=w525, y=w524) -> (x-y=w506:dbl)
                            n195 = Greater Or Equal?(x=w506, y=60.0) -> (x >= y?=w507:bool)
                            n196 = To Double Precision Float(number=w510) -> (double precision float=w509:dbl)
                            "FullSpeed2 Current" <- w509
                            n197 = Greater Or Equal?(x=w509, y=w526) -> (x >= y?=w514:bool)
                            n198 = Greater Or Equal?(x=w506, y=15.0) -> (x >= y?=w504:bool)
                            n199 = In Range and Coerce(upper limit=11000.0, x=w502, lower limit=10600.0 ("y")) -> (In Range?=w500:bool)  [unwired: 1 out]
                            n200 = And(x=w514, y=w500) -> (x .and. y?=w512:bool)
                            n201 = call "Write panel message Kinetics (SubVI).vi"(4:"rpm"=w513, 5:"rpm"=TRUE ("rpm"), "PrintTime"=FALSE, "Stop"=w515, "Time to wait"=0.2, "Strin"=w520, "String in"=w516) -> ("error out"=w522:errorcluster, "Stopped"=w511:bool)  [unwired: 2 in, 1 out]
                            n202 = Compound Arithmetic op=OR(w504, w511, w507) -> (w508:bool)
                            n203 = Compound Arithmetic op=OR(w504, w511, w517, w507, w512) -> (w527:bool)
                          }
                          n204 = Select(t=T8."Stop", s=w483, f=T8."Result") -> (s? t:f=w495:T8)
                        }
                        frame "MD[1]=1" {
                          n205 = call "Operation (SubVI).vi"("On/Off"=FALSE, "Operation"=T6."Venable", "DAQmx Device Name"=w533) -> ("error out"=w556:errorcluster)  [unwired: 8 in]
                          n206 = Concatenate Strings(w538, "\nSet Parameters MD[1]=1" ("Strin")) -> (w548:string)
                          n207 = disable-structure shown="Enabled" {
                            disable-tunnel: w556 -> [w573 w579]
                            disable-tunnel: [w572 w579] -> w555
                            disable-tunnel: w548 -> [w571 w578]
                            disable-tunnel: w547 -> [w570 w582]
                            disable-tunnel: w546 -> [w569 w581]
                            disable-tunnel: w541 -> [w568 w580]
                            disable-tunnel: [w567 w577] -> w530
                            frame Disabled {
                              n208 = call "Write panel message Kinetics (SubVI).vi"(4:"rpm"=w568, 5:"rpm"=FALSE ("rpm"), "PrintTime"=FALSE, "Stop"=w569, "error in (no error)"=w573, "Time to wait"=30.0, "Strin"=w571, "String in"=w570) -> ("error out"=w572:errorcluster, "Stopped"=w567:bool)  [unwired: 1 in, 1 out]
                            }
                            frame Enabled {
                              n209 = call "Wait Motor 0 RPM (SubVI).vi"("Strin"=w578, "error in (no error)"=w579, "Motor Speed RPM Serial"=w580, "Pannel User Message"=w582, "Stop"=w581) -> ("Stopped"=w577:bool)  [unwired: 6 in]
                            }
                          }
                          n210 = call "Serial.vi"("error in (no error)"=w555, "write buffer"="EP=1\r\nVC=0\r\nMD[1]=1\r\n", "VISA resource name"=w528) -> ("error out"=w552:errorcluster)  [unwired: 7 in, 1 out]
                          n211 = call "Operation (SubVI).vi"("error in (no error)"=w552, "On/Off"=FALSE, "Operation"=T6."PowerSuply", "DAQmx Device Name"=w533) -> ("error out"=w551:errorcluster)  [unwired: 7 in]
                          n212 = call "Write panel message Kinetics (SubVI).vi"(4:"rpm"=w541, 5:"rpm"=FALSE ("rpm"), "PrintTime"=TRUE, "Stop"=w546, "error in (no error)"=w551, "Time to wait"=25.0, "Strin"=w548, "String in"=w547) -> ("error out"=w534:errorcluster, "Stopped"=w531:bool)  [unwired: 1 in, 1 out]
                          n213 = call "Operation (SubVI).vi"("error in (no error)"=w534, "On/Off"=TRUE, "Operation"=T6."PowerSuply", "DAQmx Device Name"=w533) -> ("error out"=w535:errorcluster)  [unwired: 7 in]
                          n214 = call "Operation (SubVI).vi"("error in (no error)"=w535, "On/Off"=TRUE, "Operation"=T6."Venable", "DAQmx Device Name"=w533) -> ("error out"=w543:errorcluster)  [unwired: 7 in]
                          n215 = call "Write panel message Kinetics (SubVI).vi"(4:"rpm"=w541, 5:"rpm"=FALSE ("rpm"), "PrintTime"=TRUE, "Stop"=w546, "error in (no error)"=w543, "Time to wait"=3.0, "Strin"=w548, "String in"=w547) -> ("Stopped"=w532:bool)  [unwired: 1 in, 2 out]
                          n216 = Compound Arithmetic op=OR(w532, w531, w530) -> (w529:bool)
                          n217 = Compound Arithmetic op=OR(w532, w531, w530) -> (w540:bool)
                          n218 = Select(t=T8."Stop", s=w540, f=T8."FullSpeed2") -> (s? t:f=w566:T8)
                        }
                        frame "FullSpeed1" {
                          n219 = Search and Replace String(input string="EP=1\r\nVC=0\r\n" ("write buffer"), search string="0", replace string=w587) -> (result string=w586:string)  [unwired: 5 in, 3 out]
                          n220 = call "Serial.vi"("write buffer"=w586, "VISA resource name"=w590) -> ("error out"=w591:errorcluster)  [unwired: 8 in, 1 out]
                          n221 = Concatenate Strings(w585, "\nFull speed operation " ("string")) -> (w600:string)
                          n222 = call "Write panel message Kinetics (SubVI).vi"(4:"rpm"=w595, 5:"rpm"=TRUE ("rpm"), "PrintTime"=TRUE, "Stop"=w592, "error in (no error)"=w591, "Time to wait"=45.0, "Strin"=w600, "String in"=w593) -> ("error out"=w603:errorcluster, "Stopped"=w596:bool)  [unwired: 1 in, 1 out]
                          n223 = flat-sequence {
                            tunnel: w603 -> [w610]
                            tunnel: [w610] -> w602
                            tunnel: [w609] -> w601
                            frame #0 {
                              n224 = call <vilib>:"High Resolution Relative Seconds.vi"() -> ("relative seconds"=w609:dbl)
                            }
                          }
                          n225 = while {
                            tunnel: w602 -> [_]
                            tunnel: [w633] -> _
                            tunnel: w594 -> [w637]
                            tunnel: w601 -> [w635]
                            tunnel: w600 -> [w631]
                            tunnel: w595 -> [w622]
                            tunnel: w596 -> [w627]
                            tunnel: [w619] -> w583
                            tunnel: w593 -> [w626]
                            tunnel: w592 -> [w625]
                            tunnel: [w621] -> w584
                            stop <- w638 stop-if-true
                            n226 = call <vilib>:"High Resolution Relative Seconds.vi"() -> ("relative seconds"=w636:dbl)
                            n227 = local read "CurrentOut"() -> (w620:dbl)
                            n228 = property class="DigNum (strict)"(reference=w622) -> ("Value"=w612:dbl)  [unwired: 1 in, 2 out]
                            n229 = Subtract(x=w636, y=w635) -> (x-y=w617:dbl)
                            n230 = Greater Or Equal?(x=w617, y=60.0) -> (x >= y?=w618:bool)
                            n231 = To Double Precision Float(number=w620) -> (double precision float=→"FullSpeed1 Current":dbl)
                            n232 = Greater Or Equal?(x=w620, y=w637) -> (x >= y?=w624:bool)
                            n233 = Greater Or Equal?(x=w617, y=15.0) -> (x >= y?=w615:bool)
                            n234 = In Range and Coerce(upper limit=11000.0, x=w612, lower limit=10600.0 ("y")) -> (In Range?=w611:bool)  [unwired: 1 out]
                            n235 = And(x=w611, y=w624) -> (x .and. y?=w623:bool)
                            n236 = call "Write panel message Kinetics (SubVI).vi"(4:"rpm"=w622, 5:"rpm"=TRUE ("rpm"), "PrintTime"=FALSE, "Stop"=w625, "Time to wait"=0.2, "Strin"=w631, "String in"=w626) -> ("error out"=w633:errorcluster, "Stopped"=w621:bool)  [unwired: 2 in, 1 out]
                            n237 = Compound Arithmetic op=OR(w615, w621, w618) -> (w619:bool)
                            n238 = Compound Arithmetic op=OR(w615, w621, w627, w618, w623) -> (w638:bool)
                          }
                          n239 = Select(t=T8."Stop", s=w583, f=T8."MD[1]=1") -> (s? t:f=w606:T8)
                        }
                        frame "MD[1]=0" {
                          n240 = call "Operation (SubVI).vi"("On/Off"=FALSE, "Operation"=T6."Venable", "DAQmx Device Name"=w644) -> ("error out"=w667:errorcluster)  [unwired: 8 in]
                          n241 = Concatenate Strings(w648, "\nSet Parameters MD[1]=0" ("Strin")) -> (w659:string)
                          n242 = call "Write panel message Kinetics (SubVI).vi"(4:"rpm"=w652, 5:"rpm"=FALSE ("rpm"), "PrintTime"=FALSE, "Stop"=w657, "error in (no error)"=w667, "Time to wait"=0.2, "Strin"=w659, "String in"=w658) -> ("error out"=w666:errorcluster, "Stopped"=w640:bool)  [unwired: 1 in, 1 out]
                          n243 = call "Serial.vi"("error in (no error)"=w666, "write buffer"="EP=1\r\nVC=0\r\nMD[1]=0\r\n", "VISA resource name"=w649) -> ("error out"=w663:errorcluster)  [unwired: 7 in, 1 out]
                          n244 = call "Operation (SubVI).vi"("error in (no error)"=w663, "On/Off"=FALSE, "Operation"=T6."PowerSuply", "DAQmx Device Name"=w644) -> ("error out"=w662:errorcluster)  [unwired: 7 in]
                          n245 = call "Write panel message Kinetics (SubVI).vi"(4:"rpm"=w652, 5:"rpm"=FALSE ("rpm"), "PrintTime"=TRUE, "Stop"=w657, "error in (no error)"=w662, "Time to wait"=25.0, "Strin"=w659, "String in"=w658) -> ("error out"=w647:errorcluster, "Stopped"=w641:bool)  [unwired: 1 in, 1 out]
                          n246 = call "Operation (SubVI).vi"("error in (no error)"=w647, "On/Off"=TRUE, "Operation"=T6."PowerSuply", "DAQmx Device Name"=w644) -> ("error out"=w646:errorcluster)  [unwired: 7 in]
                          n247 = call "Operation (SubVI).vi"("error in (no error)"=w646, "On/Off"=TRUE, "Operation"=T6."Venable", "DAQmx Device Name"=w644) -> ("error out"=w654:errorcluster)  [unwired: 7 in]
                          n248 = call "Write panel message Kinetics (SubVI).vi"(4:"rpm"=w652, 5:"rpm"=FALSE ("rpm"), "PrintTime"=TRUE, "Stop"=w657, "error in (no error)"=w654, "Time to wait"=3.0, "Strin"=w659, "String in"=w658) -> ("Stopped"=w642:bool)  [unwired: 1 in, 2 out]
                          n249 = Compound Arithmetic op=OR(w642, w641, w640) -> (w639:bool)
                          n250 = Compound Arithmetic op=OR(w642, w641, w640) -> (w651:bool)
                          n251 = Select(t=T8."Stop", s=w651, f=T8."FullSpeed1") -> (s? t:f=w680:T8)
                        }
                      }
                    }
                  }
                }
              }
            }
          }
        }
        frame "Venable Test" {
          n252 = control-ref of="Stop Button"() -> (w697:refnum<vi>)
          n253 = control-ref of="ATR"() -> (w698:refnum<vi>)
          n254 = control-ref of="Pannel User Message"() -> (w699:refnum<vi>)
          n255 = control-ref of="Motor Speed RPM Serial"() -> (w700:refnum<vi>)
          n256 = control-ref of="UUT"() -> (w701:refnum<vi>)
          n257 = Concatenate Strings(w693, " in process..." ("Strin")) -> (w694:string)
          n258 = while {
            shift-right: [w708] -> _
            shift-left: enum16{"Stop", "Direction", "Venable", "Start"}."Start" -> [w713]
            tunnel: w697 -> [w712]
            tunnel: w698 -> [w711]
            tunnel: w699 -> [w710]
            tunnel: w700 -> [w709]
            tunnel: w701 -> [w706]
            tunnel: w694 -> [w707]
            tunnel: w693 -> [w705]
            tunnel: w692 -> [w704]
            tunnel: [w702] -> w691
            stop <- w703 stop-if-true
            n259 = case shown="\"Start\"" w713 {
              tunnel: w712 -> [_ w743 w992 w1041]
              tunnel: w711 -> [_ w739 w990 w1034]
              tunnel: w710 -> [_ w742 w993 w1047]
              tunnel: w709 -> [_ w741 w994 _]
              tunnel: w706 -> [w714 w735 w995 _]
              tunnel: [w716 FALSE FALSE FALSE] -> w703
              tunnel: [w715 w738 w991 w1045] -> w708
              tunnel: w707 -> [_ w740 w989 w1040]
              tunnel: w705 -> [_ _ _ w1033]
              tunnel: w704 -> [_ _ _ w1036]
              tunnel: [_ _ _ w1028] -> w702
              frame "Stop", Default {
                n260 = disable-structure shown="Enabled" {
                  disable-tunnel: [w719 TRUE] -> w716
                  disable-tunnel: [w718 enum16{"Stop", "Direction", "Venable", "Start"}."Stop"] -> w715
                  disable-tunnel: w714 -> [w717 _]
                  frame Disabled {
                    n261 = flat-sequence {
                      tunnel: w717 -> [_]
                      tunnel: [TRUE] -> w719
                      tunnel: [enum16{"Stop", "Direction", "Venable", "Start"}."Stop"] -> w718
                      frame #0 {
                        (unwired) u16 0 ("Motor Speed RPM")
                        (unwired) TRUE ("Remote")
                        n262 = property on="VISA Kinetics" class="VISAName"() -> (error out=w723:errorcluster, "Value"=w724:refnum<visa-resource-name>)  [unwired: 2 in, 1 out]
                        n263 = call "Serial.vi"("error in (no error)"=w723, "Clear Log"=FALSE, "write buffer"="EP=1\r\nMD[1]=1\r\n", "VISA resource name"=w724) -> ("error out"=w720:errorcluster)  [unwired: 6 in, 1 out]
                        n264 = call "CANSendMessage.vi"("error in (no error)"=w720) -> ("error out"=w729:errorcluster)  [unwired: 10 in]
                        n265 = call "TesterOption (SubVI).vi"("2 Options"=FALSE, "error in (no error)"=w729, "On/Off"=FALSE, "Tester Option"=T9."Venable") -> ("error out"=w725:errorcluster)  [unwired: 6 in, 1 out]
                        n266 = call "Time Delay9"("error in (no error)"=w725) -> ()  [unwired: 10 in, 1 out]
                      }
                      frame #1 {
                      }
                    }
                  }
                  frame Enabled {
                  }
                }
              }
              frame "Direction" {
                n267 = property on="UUT" class="DigNum (strict)"() -> ("Value"=w734:u8)  [unwired: 2 in, 2 out]
                n268 = while {
                  shift-right: [w754] -> w737
                  shift-left: T8."MD[1]=0" -> [w755]
                  tunnel: w735 -> [w752]
                  tunnel: w743 -> [w751]
                  tunnel: w742 -> [w750]
                  tunnel: w741 -> [w749]
                  tunnel: w740 -> [w748]
                  tunnel: w739 -> [w747]
                  tunnel: w734 -> [w746]
                  stop <- w753 stop-if-true
                  n269 = case shown="\"FullSpeed2\"" w755 {
                    tunnel: [T8."Stop" w779 w816 w886 w914 w984] -> w754
                    tunnel: [TRUE FALSE FALSE FALSE FALSE FALSE] -> w753
                    tunnel: w752 -> [_ _ _ _ _ _]
                    tunnel: w751 -> [_ w766 w793 w856 w894 w952]
                    tunnel: w750 -> [_ _ w792 w865 w893 w962]
                    tunnel: w749 -> [_ _ w809 w854 w908 w958]
                    tunnel: w748 -> [_ _ w804 w873 w906 w970]
                    tunnel: w747 -> [_ w770 _ _ _ _]
                    tunnel: w746 -> [_ w758 w790 _ w888 _]
                    frame "Stop", Default {
                    }
                    frame "Result" {
                      n270 = property on="FullSpeed1 Current" class="DigNum (strict)"() -> ("Value"=w774:dbl)  [unwired: 2 in, 2 out]
                      n271 = property on="FullSpeed2 Current" class="DigNum (strict)"() -> ("Value"=w775:dbl)  [unwired: 2 in, 2 out]
                      n272 = property on="FullSpeed2 Speed" class="DigNum (strict)"() -> ("Value"=w777:dbl)  [unwired: 2 in, 2 out]
                      n273 = property on="FullSpeed1 Speed" class="DigNum (strict)"() -> ("Value"=w776:dbl)  [unwired: 2 in, 2 out]
                      n274 = Subtract(x=w775, y=w774) -> (x-y=w773:dbl)
                      n275 = Absolute Value(x=w773) -> (abs(x)=w762:dbl)
                      n276 = Greater Or Equal?(x=w762, y=u32 5) -> (x >= y?=w768:bool)
                      n277 = Equal?(x=w758, y=u8 95) -> (x = y?=w760:bool)
                      n278 = case shown="True" w760 {
                        tunnel: w777 -> [_ w788]
                        tunnel: w776 -> [_ w787]
                        tunnel: [TRUE w784] -> w769
                        frame False {
                        }
                        frame True {
                          n279 = Subtract(x=w788, y=w787) -> (x-y=w789:dbl)
                          n280 = Absolute Value(x=w789) -> (abs(x)=w786:dbl)
                          n281 = Greater Or Equal?(x=w786, y=500.0) -> (x >= y?=w784:bool)
                        }
                      }
                      n282 = call "Find_Number_LineMARVIN.vi"("Test Paragraph"="Motor Rotation Direction", "TableIn"=w770) -> ("Line number"=w767:i32)  [unwired: 3 in, 3 out]
                      n283 = And(x=w769, y=w768) -> (x .and. y?=w759:bool)
                      "VenableDirectionResult" <- w759
                      n284 = call "PassOrFail (SubVI).vi"("String Res"="", "index (row)"=w767, "Data in"=-3.0, "Pass?Fail"=w759, "Table in"=w770) -> ("error out"=w765:errorcluster)  [unwired: 6 in]
                      n285 = property class="Bool (strict)"(reference=w766, error in=w765) -> ("Value"=w782:bool)  [unwired: 2 out]
                      n286 = Select(t=T8."Stop", s=w782, f=T8."Stop") -> (s? t:f=w779:T8)
                    }
                    frame "FullSpeed2" {
                      (unwired) TRUE ("Remote")
                      n287 = Concatenate Strings(w804, "\nFull speed operation " ("string")) -> (w791:string)
                      n288 = call "CANSendMessage.vi"() -> ("error out"=w811:errorcluster)  [unwired: 11 in]
                      n289 = call "Write panel message Kinetics (SubVI).vi"(4:"rpm"=w809, 5:"rpm"=TRUE ("rpm"), "PrintTime"=FALSE, "Stop"=w793, "error in (no error)"=w811, "Time to wait"=0.2, "Strin"=w791, "String in"=w792) -> ("error out"=w796:errorcluster)  [unwired: 1 in, 2 out]
                      n290 = Equal?(x=w790, y=u8 95) -> (x = y?=w799:bool)
                      n291 = Select(t=u16 15100, s=w799, f=u16 12100 ("y")) -> ()  [unwired: 1 out]
                      n292 = flat-sequence {
                        tunnel: w796 -> [w821]
                        tunnel: [w821] -> w795
                        tunnel: [w820] -> w794
                        frame #0 {
                          n293 = call <vilib>:"High Resolution Relative Seconds.vi"() -> ("relative seconds"=w820:dbl)
                        }
                      }
                      n294 = Select(t=14500.0, s=w799, f=11500.0) -> (s? t:f=w798:dbl)
                      n295 = Select(t=47.0, s=w799, f=24.0) -> (s? t:f=w797:dbl)
                      n296 = while {
                        tunnel: w809 -> [w823]
                        tunnel: w795 -> [w847]
                        tunnel: [w830] -> w806
                        tunnel: w798 -> [w843]
                        tunnel: w797 -> [w842]
                        tunnel: w794 -> [w838]
                        tunnel: w793 -> [w828]
                        tunnel: w792 -> [w829]
                        tunnel: w791 -> [w826]
                        stop <- w840 stop-if-true
                        n297 = call <vilib>:"High Resolution Relative Seconds.vi"() -> ("relative seconds"=w839:dbl)
                        n298 = Subtract(x=w839, y=w838) -> (x-y=w837:dbl)
                        n299 = property class="DigNum (strict)"(reference=w823, error in=w847) -> ("Value"=w844:dbl)  [unwired: 2 out]
                        "FullSpeed2 Speed" <- w844
                        n300 = Greater Or Equal?(x=w837, y=120.0) -> (x >= y?=w835:bool)
                        n301 = Greater Or Equal?(x=w844, y=w843) -> (x >= y?=w834:bool)
                        n302 = property class="Bool (strict)"(reference=w828) -> ("Value"=w833:bool)  [unwired: 1 in, 2 out]
                        n303 = call "GetADCTester (SubVI).vi"("GetADCTester"=T10."Current", "TimeToGet"=5) -> ("error out"=w845:errorcluster, "ADCValOutput Single"=w841:dbl)  [unwired: 7 in, 1 out]
                        "FullSpeed2 Current" <- w841
                        n304 = Greater Or Equal?(x=w841, y=w842) -> (x >= y?=w831:bool)
                        n305 = And(x=w834, y=w831) -> (x .and. y?=w832:bool)
                        n306 = Compound Arithmetic op=OR(w833, w835, w832) -> (w840:bool)
                        n307 = call "Write panel message Kinetics (SubVI).vi"(4:"rpm"=w823, 5:"rpm"=TRUE ("rpm"), "PrintTime"=FALSE, "Stop"=w828, "error in (no error)"=w845, "Time to wait"=0.2, "Strin"=w826, "String in"=w829) -> ("error out"=w830:errorcluster)  [unwired: 1 in, 2 out]
                      }
                      n308 = property class="Bool (strict)"(reference=w793, error in=w806) -> ("Value"=w819:bool)  [unwired: 2 out]
                      n309 = Select(t=T8."Stop", s=w819, f=T8."Result") -> (s? t:f=w816:T8)
                    }
                    frame "MD[1]=1" {
                      (unwired) TRUE ("Remote")
                      (unwired) u16 0 ("Motor Speed RPM")
                      n310 = Concatenate Strings(w873, "\nSet Parameters MD[1]=1" ("Strin")) -> (w864:string)
                      n311 = call "TesterOption (SubVI).vi"("2 Options"=FALSE, "On/Off"=FALSE, "Tester Option"=T9."Venable") -> ("error out"=w878:errorcluster, "VISA Refnum out"=w869:refnum<visa-resource-name>)  [unwired: 7 in]
                      n312 = call "CANSendMessage.vi"("error in (no error)"=w878) -> ("error out"=w880:errorcluster)  [unwired: 10 in]
                      n313 = call "Write panel message Kinetics (SubVI).vi"(4:"rpm"=w854, 5:"rpm"=FALSE ("rpm"), "PrintTime"=TRUE, "Stop"=w856, "error in (no error)"=w880, "Time to wait"=20.0, "Strin"=w864, "String in"=w865) -> ("error out"=w853:errorcluster)  [unwired: 1 in, 2 out]
                      n314 = property on="VISA Kinetics" class="VISAName"(error in=w853) -> (error out=w879:errorcluster, "Value"=w882:refnum<visa-resource-name>)  [unwired: 1 in, 1 out]
                      n315 = call "Serial.vi"("error in (no error)"=w879, "Clear Log"=FALSE, "write buffer"="EP=1\r\nMD[1]=1\r\n", "VISA resource name"=w882) -> ("error out"=w868:errorcluster)  [unwired: 6 in, 1 out]
                      n316 = call "TesterOption (SubVI).vi"("2 Options"=FALSE, "error in (no error)"=w868, "On/Off"=FALSE, "Tester Option"=T9."Power", "VISA Refnum in"=w869) -> ("error out"=w866:errorcluster, "VISA Refnum out"=w857:refnum<visa-resource-name>)  [unwired: 5 in]
                      n317 = call "Write panel message Kinetics (SubVI).vi"(4:"rpm"=w854, 5:"rpm"=FALSE ("rpm"), "PrintTime"=TRUE, "Stop"=w856, "error in (no error)"=w866, "Time to wait"=25.0, "Strin"=w864, "String in"=w865) -> ("error out"=w858:errorcluster)  [unwired: 1 in, 2 out]
                      n318 = call "TesterOption (SubVI).vi"("2 Options"=FALSE, "error in (no error)"=w858, "On/Off"=TRUE, "Tester Option"=T9."Venable", "VISA Refnum in"=w857) -> ("error out"=w855:errorcluster)  [unwired: 5 in, 1 out]
                      n319 = call "Time Delay8"("error in (no error)"=w855) -> ("error out"=w851:errorcluster)  [unwired: 10 in]
                      n320 = property class="Bool (strict)"(reference=w856, error in=w851) -> ("Value"=w887:bool)  [unwired: 2 out]
                      n321 = Select(t=T8."Stop", s=w887, f=T8."FullSpeed2") -> (s? t:f=w886:T8)
                    }
                    frame "FullSpeed1" {
                      (unwired) TRUE ("Remote")
                      n322 = call "CANSendMessage.vi"() -> ("error out"=w909:errorcluster)  [unwired: 11 in]
                      n323 = Concatenate Strings(w906, "\nFull speed operation " ("string")) -> (w892:string)
                      n324 = call "Write panel message Kinetics (SubVI).vi"(4:"rpm"=w908, 5:"rpm"=TRUE ("rpm"), "PrintTime"=FALSE, "Stop"=w894, "error in (no error)"=w909, "Time to wait"=0.2, "Strin"=w892, "String in"=w893) -> ("error out"=w897:errorcluster)  [unwired: 1 in, 2 out]
                      n325 = Equal?(x=w888, y=u8 95) -> (x = y?=w904:bool)
                      n326 = flat-sequence {
                        tunnel: w897 -> [w919]
                        tunnel: [w919] -> w896
                        tunnel: [w918] -> w895
                        frame #0 {
                          n327 = call <vilib>:"High Resolution Relative Seconds.vi"() -> ("relative seconds"=w918:dbl)
                        }
                      }
                      n328 = Select(t=u16 15100, s=w904, f=u16 12100 ("y")) -> ()  [unwired: 1 out]
                      n329 = Select(t=13700.0, s=w904, f=11500.0) -> (s? t:f=w899:dbl)
                      n330 = Select(t=56.0, s=w904, f=33.0) -> (s? t:f=w898:dbl)
                      n331 = while {
                        tunnel: w908 -> [w921]
                        tunnel: w896 -> [w945]
                        tunnel: [w928] -> w907
                        tunnel: w899 -> [w940]
                        tunnel: w898 -> [w937]
                        tunnel: w895 -> [w935]
                        tunnel: w894 -> [w926]
                        tunnel: w893 -> [w927]
                        tunnel: w892 -> [w924]
                        stop <- w942 stop-if-true
                        n332 = property class="DigNum (strict)"(reference=w921, error in=w945) -> ("Value"=w941:dbl)  [unwired: 2 out]
                        "FullSpeed1 Speed" <- w941
                        n333 = call <vilib>:"High Resolution Relative Seconds.vi"() -> ("relative seconds"=w936:dbl)
                        n334 = Subtract(x=w936, y=w935) -> (x-y=w934:dbl)
                        n335 = Greater Or Equal?(x=w934, y=120.0) -> (x >= y?=w932:bool)
                        n336 = Greater Or Equal?(x=w941, y=w940) -> (x >= y?=w939:bool)
                        n337 = call "GetADCTester (SubVI).vi"("GetADCTester"=T10."Current", "TimeToGet"=5) -> ("error out"=w943:errorcluster, "ADCValOutput Single"=w938:dbl)  [unwired: 7 in, 1 out]
                        "FullSpeed1 Current" <- w938
                        n338 = Greater Or Equal?(x=w938, y=w937) -> (x >= y?=w929:bool)
                        n339 = And(x=w929, y=w939) -> (x .and. y?=w930:bool)
                        n340 = property class="Bool (strict)"(reference=w926) -> ("Value"=w931:bool)  [unwired: 1 in, 2 out]
                        n341 = call "Write panel message Kinetics (SubVI).vi"(4:"rpm"=w921, 5:"rpm"=TRUE ("rpm"), "PrintTime"=FALSE, "Stop"=w926, "error in (no error)"=w943, "Time to wait"=0.2, "Strin"=w924, "String in"=w927) -> ("error out"=w928:errorcluster)  [unwired: 1 in, 2 out]
                        n342 = Compound Arithmetic op=OR(w931, w930, w932) -> (w942:bool)
                      }
                      n343 = property class="Bool (strict)"(reference=w894, error in=w907) -> ("Value"=w917:bool)  [unwired: 2 out]
                      n344 = Select(t=T8."Stop", s=w917, f=T8."MD[1]=1") -> (s? t:f=w914:T8)
                    }
                    frame "MD[1]=0" {
                      (unwired) TRUE ("Remote")
                      (unwired) u16 0 ("Motor Speed RPM")
                      n345 = Concatenate Strings(w970, "\nSet Parameters MD[1]=0" ("Strin")) -> (w961:string)
                      n346 = call "TesterOption (SubVI).vi"("2 Options"=FALSE, "On/Off"=FALSE, "Tester Option"=T9."Venable") -> ("error out"=w976:errorcluster, "VISA Refnum out"=w966:refnum<visa-resource-name>)  [unwired: 7 in]
                      n347 = call "CANSendMessage.vi"("error in (no error)"=w976) -> ("error out"=w978:errorcluster)  [unwired: 10 in]
                      n348 = call "Write panel message Kinetics (SubVI).vi"(4:"rpm"=w958, 5:"rpm"=FALSE ("rpm"), "PrintTime"=FALSE, "Stop"=w952, "error in (no error)"=w978, "Time to wait"=0.2, "Strin"=w961, "String in"=w962) -> ("error out"=w973:errorcluster)  [unwired: 1 in, 2 out]
                      n349 = property on="VISA Kinetics" class="VISAName"(error in=w973) -> (error out=w977:errorcluster, "Value"=w980:refnum<visa-resource-name>)  [unwired: 1 in, 1 out]
                      n350 = call "Serial.vi"("error in (no error)"=w977, "Clear Log"=FALSE, "write buffer"="EP=1\r\nMD[1]=0\r\n", "VISA resource name"=w980) -> ("error out"=w965:errorcluster)  [unwired: 6 in, 1 out]
                      n351 = call "TesterOption (SubVI).vi"("2 Options"=FALSE, "error in (no error)"=w965, "On/Off"=FALSE, "Tester Option"=T9."Power", "VISA Refnum in"=w966) -> ("error out"=w963:errorcluster, "VISA Refnum out"=w953:refnum<visa-resource-name>)  [unwired: 5 in]
                      n352 = call "Write panel message Kinetics (SubVI).vi"(4:"rpm"=w958, 5:"rpm"=FALSE ("rpm"), "PrintTime"=TRUE, "Stop"=w952, "error in (no error)"=w963, "Time to wait"=25.0, "Strin"=w961, "String in"=w962) -> ("error out"=w954:errorcluster)  [unwired: 1 in, 2 out]
                      n353 = call "TesterOption (SubVI).vi"("2 Options"=FALSE, "error in (no error)"=w954, "On/Off"=TRUE, "Tester Option"=T9."Venable", "VISA Refnum in"=w953) -> ("error out"=w951:errorcluster)  [unwired: 5 in, 1 out]
                      n354 = call "Time Delay4"("error in (no error)"=w951) -> ("error out"=w947:errorcluster)  [unwired: 10 in]
                      n355 = property class="Bool (strict)"(reference=w952, error in=w947) -> ("Value"=w985:bool)  [unwired: 2 out]
                      n356 = Select(t=T8."Stop", s=w985, f=T8."FullSpeed1") -> (s? t:f=w984:T8)
                    }
                  }
                }
                n357 = flat-sequence {
                  tunnel: [enum16{"Stop", "Direction", "Venable", "Start"}."Stop"] -> w738
                  tunnel: w737 -> [_]
                  frame #0 {
                  }
                }
              }
              frame "Venable" {
                n358 = call "Find_Number_LineMARVIN.vi"("Test Paragraph"="Enable Test", "TableIn"=w990) -> ("Line number"=w996:i32)  [unwired: 3 in, 3 out]
                n359 = Increment(x=w996) -> (x+1=w986:i32)
                n360 = for {
                  tunnel: u16[] [5000, 0, 5000] -> [w1021] mode=indexing
                  tunnel: bool[] [TRUE, FALSE, TRUE] -> [w1019] mode=indexing
                  tunnel: w986 -> [w1022]
                  tunnel: w995 -> [_]
                  tunnel: w994 -> [w1012]
                  tunnel: w993 -> [w1015]
                  tunnel: w992 -> [w1014]
                  tunnel: w990 -> [w1008]
                  tunnel: w989 -> [w1006]
                  tunnel: [w1005] -> w988 mode=indexing
                  i -> [w1023]
                  (unwired) u16 5000 ("Motor Speed RPM")
                  (unwired) TRUE ("Remote")
                  w1024 = 200.0 ("y")
                  n361 = call "CANSendMessage.vi"() -> ("error out"=w1018:errorcluster)  [unwired: 11 in]
                  n362 = Add(x=w1022, y=w1023) -> (x+y=w1009:i32)
                  n363 = call "TesterOption (SubVI).vi"("2 Options"=FALSE, "error in (no error)"=w1018, "On/Off"=w1019, "Tester Option"=T9."Venable") -> ("error out"=w1017:errorcluster)  [unwired: 6 in, 1 out]
                  n364 = call "Write panel message Kinetics (SubVI).vi"(4:"rpm"=w1012, 5:"rpm"=TRUE ("rpm"), "PrintTime"=TRUE, "Stop"=w1014, "error in (no error)"=w1017, "Time to wait"=15.0, "Strin"=w1006, "String in"=w1015) -> ("error out"=w1016:errorcluster)  [unwired: 1 in, 2 out]
                  n365 = property class="DigNum (strict)"(reference=w1012, error in=w1016) -> ("Value"=w1007:dbl)  [unwired: 2 out]
                  n366 = Add(x=w1021, y=w1024) -> (x+y=w1026:dbl)
                  n367 = Subtract(x=w1021, y=w1024) -> (x-y=w1025:dbl)
                  n368 = In Range and Coerce(upper limit=w1026, x=w1007, lower limit=w1025) -> (In Range?=w1005:bool)  [unwired: 1 out]
                  n369 = call "PassOrFail (SubVI).vi"("index (row)"=w1009, "Data in"=w1007, "Pass?Fail"=w1005, "Table in"=w1008) -> ()  [unwired: 7 in, 1 out]
                }
                n370 = property class="Bool (strict)"(reference=w992) -> ("Value"=w1003:bool)  [unwired: 1 in, 2 out]
                n371 = And Array Elements(Boolean array=w988) -> (logical AND=→"VenableResult":bool)
                n372 = Select(t=enum16{"Stop", "Direction", "Venable", "Start"}."Stop", s=w1003, f=enum16{"Stop", "Direction", "Venable", "Start"}."Direction") -> (s? t:f=w991:enum16{"Stop", "Direction", "Venable", "Start"})
              }
              frame "Start" {
                n373 = property class="Str"(reference=w1047, "Value"=w1040) -> (error out=w1044:errorcluster)  [unwired: 1 in, 1 out]
                n374 = call "Find_Number_LineMARVIN.vi"("Test Paragraph"=w1033, "error in"=w1044, "TableIn"=w1034) -> ("error out"=w1035:errorcluster, "Line number"=w1032:i32)  [unwired: 2 in, 2 out]
                n375 = control-ref of="Motor Speed RPM Serial"() -> (w1027:refnum<vi>)
                n376 = call "Table_ScrollaBarMarvin.vi"("error in"=w1035, "Line to focus"=w1033, "reference in"=w1034) -> ("error out"=w1048:errorcluster)  [unwired: 2 out]
                n377 = call "Reset old test Values (SubVI) Kinetics.vi"("error in"=w1048, "Atr in"=w1034, "Test Paragraph"=w1033) -> ("error out"=w1029:errorcluster)  [unwired: 6 in, 2 out]
                n378 = Increment(x=w1032) -> (x+1=w1031:i32)
                n379 = while {
                  shift-right: [w1061] -> _
                  shift-left: T7."VC=1000" -> [w1064]
                  tunnel: w1029 -> [w1063]
                  tunnel: w1036 -> [w1062]
                  tunnel: w1033 -> [w1060]
                  shift-right: [w1057] -> w1039
                  shift-left: bool[] [FALSE, FALSE] -> [w1058]
                  tunnel: w1031 -> [w1056]
                  tunnel: w1034 -> [w1055]
                  shift-right: [w1053] -> _
                  shift-left: dbl[] [0.0, 0.0] -> [w1054]
                  tunnel: [w1051] -> w1028
                  tunnel: w1027 -> [w1050]
                  i -> [w1059]
                  stop <- w1052 stop-if-true
                  n380 = case shown="\"Wait\"" w1064 {
                    tunnel: w1063 -> [_ w1082 _ w1128 _]
                    tunnel: w1062 -> [_ w1081 w1097 w1132 _]
                    tunnel: [T7."Exit" T7."Wait" w1094 T7."Wait" T7."ReadVC"] -> w1061
                    tunnel: w1060 -> [_ _ _ _ w1139]
                    tunnel: [TRUE FALSE FALSE FALSE w1135] -> w1052
                    tunnel: w1059 -> [_ _ w1095 _ _]
                    tunnel: w1058 -> [w1066 w1079 w1093 w1130 w1137]
                    tunnel: [w1066 w1079 w1092 w1130 w1137] -> w1057
                    tunnel: w1056 -> [w1067 _ _ _ _]
                    tunnel: w1055 -> [w1068 _ _ _ _]
                    tunnel: w1054 -> [w1065 w1077 w1090 w1123 w1136]
                    tunnel: [w1065 w1077 w1089 w1123 w1136] -> w1053
                    tunnel: [_ _ _ _ w1135] -> w1051
                    tunnel: w1050 -> [_ _ _ _ w1134]
                    frame "Exit", Default {
                      n381 = for {
                        tunnel: w1068 -> [w1076]
                        tunnel: w1067 -> [w1075]
                        tunnel: w1066 -> [w1074] mode=indexing
                        tunnel: w1065 -> [w1071] mode=indexing
                        i -> [w1072]
                        n382 = Add(x=w1072, y=w1075) -> (x+y=w1073:i32)
                        n383 = call "PassOrFail (SubVI).vi"("index (row)"=w1073, "Data in"=w1071, "Pass?Fail"=w1074, "Table in"=w1076) -> ()  [unwired: 7 in, 1 out]
                      }
                    }
                    frame "VC=0" {
                      n384 = disable-structure shown="Enabled" {
                        disable-tunnel: w1082 -> [w1085 _]
                        disable-tunnel: w1081 -> [w1083 _]
                        frame Disabled {
                          n385 = call "Serial.vi"("error in (no error)"=w1085, "write buffer"="EP=1\r\nVC=0\r\n", "VISA resource name"=w1083) -> ()  [unwired: 7 in, 2 out]
                        }
                        frame Enabled {
                          n386 = local read "DAQmx Device Name"() -> (w1088:tag)
                          n387 = call "Operation (SubVI).vi"("On/Off"=FALSE, "Operation"=T6."Venable", "DAQmx Device Name"=w1088) -> ()  [unwired: 8 in, 1 out]
                        }
                      }
                    }
                    frame "ReadVC" {
                      n388 = call "Serial.vi"("write buffer"="VC\r\n", "VISA resource name"=w1097) -> ("read buffer"=w1096:string)  [unwired: 8 in, 1 out]
                      n389 = case shown="2" w1095 {
                        tunnel: w1096 -> [w1109 w1119]
                        tunnel: [T7."VC=0" T7."Exit"] -> w1094
                        tunnel: w1093 -> [w1105 w1118]
                        tunnel: [w1103 w1115] -> w1092
                        tunnel: w1090 -> [w1102 w1114]
                        tunnel: [w1099 w1111] -> w1089
                        frame 2 {
                          n390 = Decimal String To Number(string=w1109) -> (number=w1100:i32)  [unwired: 2 in, 1 out]
                          n391 = In Range and Coerce(upper limit=1100, x=w1100, lower limit=900) -> (In Range?=w1104:bool)  [unwired: 1 out]
                          n392 = Replace Array Subset(array=w1102, new element=w1100, index=0) -> (w1099:dbl[])
                          n393 = Replace Array Subset(array=w1105, new element=w1104, index=0) -> (w1103:bool[])
                        }
                        frame 5, Default {
                          n394 = Decimal String To Number(string=w1119) -> (number=w1112:i32)  [unwired: 2 in, 1 out]
                          n395 = In Range and Coerce(upper limit=100, x=w1112, lower limit=0) -> (In Range?=w1116:bool)  [unwired: 1 out]
                          n396 = Replace Array Subset(array=w1114, new element=w1112, index=1) -> (w1111:dbl[])
                          n397 = Replace Array Subset(array=w1118, new element=w1116, index=1) -> (w1115:bool[])
                        }
                      }
                    }
                    frame "VC=1000" {
                      n398 = local read "DAQmx Device Name"() -> (w1129:tag)
                      n399 = call "Operation (SubVI).vi"("error in (no error)"=w1128, "On/Off"=TRUE, "Operation"=T6."Venable", "DAQmx Device Name"=w1129) -> ("error out"=w1127:errorcluster)  [unwired: 7 in]
                      n400 = call "Serial.vi"("error in (no error)"=w1127, "write buffer"="EP=1\r\nVC=1000\r\n", "VISA resource name"=w1132) -> ()  [unwired: 7 in, 2 out]
                    }
                    frame "Wait" {
                      n401 = while {
                        tunnel: w1139 -> [w1151]
                        tunnel: [w1149] -> w1135
                        tunnel: w1134 -> [w1148]
                        i -> [w1142]
                        stop <- w1143 stop-if-true
                        n402 = property class="DigNum (strict)"(reference=w1148) -> ("Value"=w1145:dbl)  [unwired: 1 in, 2 out]
                        n403 = Equal?(x=3, y=w1142) -> (x = y?=w1140:bool)
                        n404 = control-ref of="Pannel User Message"() -> (w1155:refnum<vi>)
                        n405 = control-ref of="Stop Button"() -> (w1150:refnum<vi>)
                        n406 = call "Write panel message Kinetics (SubVI).vi"(4:"rpm"=w1148, 5:"rpm"=TRUE ("rpm"), "PrintTime"=TRUE, "Stop"=w1150, "Time to wait"=20.0, "Strin"=w1151, "String in"=w1155) -> ("Stopped"=w1149:bool)  [unwired: 2 in, 2 out]
                        n407 = In Range and Coerce(upper limit=1100.0, x=w1145, lower limit=900.0) -> (In Range?=w1144:bool)  [unwired: 1 out]
                        n408 = Or(x=w1140, y=w1144) -> (x .or. y?=w1143:bool)
                      }
                    }
                  }
                }
                n409 = And Array Elements(Boolean array=w1039) -> ()  [unwired: 1 out]
                n410 = property class="Bool (strict)"(reference=w1041) -> ("Value"=w1049:bool)  [unwired: 1 in, 2 out]
                n411 = Select(t=enum16{"Stop", "Direction", "Venable", "Start"}."Stop", s=w1049, f=enum16{"Stop", "Direction", "Venable", "Start"}."Stop") -> (s? t:f=w1045:enum16{"Stop", "Direction", "Venable", "Start"})
              }
            }
          }
        }
        frame "Motor Thermistor Test" {
          n412 = Concatenate Strings(w1167, " in process..." ("Strin")) -> (w1168:string)
          n413 = control-ref of="ATR"() -> (w1170:refnum<vi>)
          n414 = control-ref of="Pannel User Message"() -> (w1171:refnum<vi>)
          n415 = property class="Str"(reference=w1171, "Value"=w1168) -> (error out=w1164:errorcluster)  [unwired: 1 in, 1 out]
          n416 = call "Find_Number_LineMARVIN.vi"("Test Paragraph"=w1167, "error in"=w1164, "TableIn"=w1170) -> ("error out"=w1161:errorcluster, "Line number"=w1160:i32)  [unwired: 2 in, 2 out]
          n417 = call "Table_ScrollaBarMarvin.vi"("error in"=w1161, "Line to focus"=w1167, "reference in"=w1170) -> ("error out"=w1165:errorcluster)  [unwired: 2 out]
          n418 = call "Reset old test Values (SubVI) Kinetics.vi"("error in"=w1165, "Atr in"=w1170, "Test Paragraph"=w1167) -> ("error out"=w1157:errorcluster)  [unwired: 6 in, 2 out]
          n419 = Increment(x=w1160) -> (x+1=w1159:i32)
          n420 = while {
            shift-right: [w1182] -> _
            shift-left: T7."VC=1000" -> [w1185]
            tunnel: w1157 -> [w1184]
            tunnel: w1166 -> [w1183]
            tunnel: w1167 -> [w1181]
            shift-right: [w1177] -> _
            shift-left: bool[] [FALSE, FALSE] -> [w1178]
            tunnel: w1159 -> [w1176]
            tunnel: w1170 -> [w1175]
            shift-right: [w1173] -> _
            shift-left: dbl[] [0.0, 0.0] -> [w1174]
            tunnel: [w1172] -> w1156
            i -> [w1179]
            stop <- w1180 stop-if-true
            n421 = case shown="\"Wait\"" w1185 {
              tunnel: w1184 -> [_ w1209 _ w1266 _]
              tunnel: w1183 -> [w1186 w1208 w1225 w1270 _]
              tunnel: [T7."Exit" T7."Wait" w1222 T7."Wait" T7."ReadVC"] -> w1182
              tunnel: w1181 -> [_ _ _ _ w1277]
              tunnel: [TRUE FALSE FALSE FALSE w1272] -> w1180
              tunnel: w1179 -> [_ w1203 w1223 _ _]
              tunnel: w1178 -> [w1192 w1206 w1221 w1268 w1274]
              tunnel: [w1192 w1206 w1220 w1268 w1274] -> w1177
              tunnel: w1176 -> [w1193 _ _ _ _]
              tunnel: w1175 -> [w1194 _ _ _ _]
              tunnel: w1174 -> [w1191 w1204 w1218 w1261 w1273]
              tunnel: [w1191 w1204 w1217 w1261 w1273] -> w1173
              tunnel: [_ _ _ _ w1272] -> w1172
              frame "Exit", Default {
                n422 = for {
                  tunnel: w1194 -> [w1202]
                  tunnel: w1193 -> [w1201]
                  tunnel: w1192 -> [w1200] mode=indexing
                  tunnel: w1191 -> [w1197] mode=indexing
                  i -> [w1198]
                  n423 = Add(x=w1198, y=w1201) -> (x+y=w1199:i32)
                  n424 = call "PassOrFail (SubVI).vi"("index (row)"=w1199, "Data in"=w1197, "Pass?Fail"=w1200, "Table in"=w1202) -> ()  [unwired: 7 in, 1 out]
                }
                n425 = local read "DAQmx Device Name"() -> (w1190:tag)
                n426 = call "Serial.vi"("write buffer"="EP=1\r\nVC=0\r\n", "VISA resource name"=w1186) -> ()  [unwired: 8 in, 2 out]
                n427 = call "Operation (SubVI).vi"("On/Off"=FALSE, "Operation"=T6."Venable", "DAQmx Device Name"=w1190) -> ()  [unwired: 8 in, 1 out]
              }
              frame "VC=0" {
                n428 = disable-structure shown="Enabled" {
                  disable-tunnel: w1209 -> [w1212 _]
                  disable-tunnel: w1208 -> [w1210 _]
                  disable-tunnel: w1203 -> [_ w1213]
                  frame Disabled {
                    n429 = call "Serial.vi"("error in (no error)"=w1212, "write buffer"="EP=1\r\nVC=0\r\n", "VISA resource name"=w1210) -> ()  [unwired: 7 in, 2 out]
                  }
                  frame Enabled {
                    n430 = case shown="6, Default" w1213 {
                      tunnel: ["Connect wires of the thermistor" ("message") "Disconnect wires of the thermistor" ("message")] -> w1214
                      frame 6, Default {
                      }
                      frame 3 {
                      }
                    }
                    n431 = One Button Dialog(message=w1214) -> ()  [unwired: 1 in, 1 out]
                  }
                }
              }
              frame "ReadVC" {
                n432 = call "Serial.vi"("write buffer"="VC\r\n", "VISA resource name"=w1225) -> ("read buffer"=w1224:string)  [unwired: 8 in, 1 out]
                n433 = case shown="2" w1223 {
                  tunnel: w1224 -> [w1236 w1245 w1257]
                  tunnel: [w1230 T7."VC=0" T7."Exit"] -> w1222
                  tunnel: w1221 -> [w1227 w1244 w1256]
                  tunnel: [w1227 w1241 w1253] -> w1220
                  tunnel: w1218 -> [w1228 w1240 w1252]
                  tunnel: [w1228 w1237 w1249] -> w1217
                  frame 2 {
                    n434 = Decimal String To Number(string=w1236) -> (number=w1233:i32)  [unwired: 2 in, 1 out]
                    n435 = In Range and Coerce(upper limit=1100, x=w1233, lower limit=900) -> (In Range?=w1232:bool)  [unwired: 1 out]
                    n436 = Select(t=T7."VC=0", s=w1232, f=T7."Exit") -> (s? t:f=w1230:T7)
                  }
                  frame 5, Default {
                    n437 = Decimal String To Number(string=w1245) -> (number=w1238:i32)  [unwired: 2 in, 1 out]
                    n438 = In Range and Coerce(upper limit=100, x=w1238, lower limit=0) -> (In Range?=w1242:bool)  [unwired: 1 out]
                    n439 = Replace Array Subset(array=w1240, new element=w1238, index=0) -> (w1237:dbl[])
                    n440 = Replace Array Subset(array=w1244, new element=w1242, index=0) -> (w1241:bool[])
                  }
                  frame 8 {
                    n441 = Decimal String To Number(string=w1257) -> (number=w1250:i32)  [unwired: 2 in, 1 out]
                    n442 = In Range and Coerce(upper limit=1100, x=w1250, lower limit=900) -> (In Range?=w1254:bool)  [unwired: 1 out]
                    n443 = Replace Array Subset(array=w1252, new element=w1250, index=1) -> (w1249:dbl[])
                    n444 = Replace Array Subset(array=w1256, new element=w1254, index=1) -> (w1253:bool[])
                  }
                }
              }
              frame "VC=1000" {
                n445 = local read "DAQmx Device Name"() -> (w1267:tag)
                n446 = call "Operation (SubVI).vi"("error in (no error)"=w1266, "On/Off"=TRUE, "Operation"=T6."Venable", "DAQmx Device Name"=w1267) -> ("error out"=w1265:errorcluster)  [unwired: 7 in]
                n447 = call "Serial.vi"("error in (no error)"=w1265, "write buffer"="EP=1\r\nVC=1000\r\n", "VISA resource name"=w1270) -> ()  [unwired: 7 in, 2 out]
              }
              frame "Wait" {
                n448 = control-ref of="Motor Speed RPM Serial"() -> (w1282:refnum<vi>)
                n449 = control-ref of="Pannel User Message"() -> (w1281:refnum<vi>)
                n450 = control-ref of="Stop Button"() -> (w1276:refnum<vi>)
                n451 = call "Write panel message Kinetics (SubVI).vi"(4:"rpm"=w1282, 5:"rpm"=TRUE ("rpm"), "PrintTime"=TRUE, "Stop"=w1276, "Time to wait"=20.0, "Strin"=w1277, "String in"=w1281) -> ("Stopped"=w1272:bool)  [unwired: 2 in, 2 out]
              }
            }
          }
        }
        frame "Up/Down Blower Test" {
          n452 = control-ref of="Pannel User Message"() -> (w1314:refnum<vi>)
          n453 = Concatenate Strings(w1306, " in process..." ("Strin")) -> (w1285:string)
          n454 = property class="Str"(reference=w1314, error in=w1313, "Value"=w1285) -> (error out=w1312:errorcluster)  [unwired: 1 out]
          n455 = call "Table_ScrollaBarMarvin.vi"("error in"=w1312, "Line to focus"=w1306, "reference in"=w1300) -> ()  [unwired: 3 out]
          n456 = call "Reset old test Values (SubVI) Kinetics.vi"("Atr in"=w1300, "Test Paragraph"=w1306) -> ("error out"=w1307:errorcluster)  [unwired: 7 in, 2 out]
          n457 = call "Find_Number_LineMARVIN.vi"("Test Paragraph"=w1306, "error in"=w1307, "TableIn"=w1300) -> ("error out"=w1292:errorcluster, "Line number"=w1305:i32)  [unwired: 2 in, 2 out]
          n458 = control-ref of="Motor Speed RPM Serial"() -> (w1286:refnum<vi>)
          n459 = local read "DAQmx Device Name"() -> (w1293:tag)
          n460 = call "Operation (SubVI).vi"("error in (no error)"=w1292, "On/Off"=TRUE, "Operation"=T6."PowerSuply", "DAQmx Device Name"=w1293) -> ("error out"=w1284:errorcluster)  [unwired: 7 in]
          n461 = control-ref of="Pannel User Message"() -> (w1287:refnum<vi>)
          n462 = control-ref of="Stop Button"() -> (w1291:refnum<vi>)
          n463 = call "Write panel message Kinetics (SubVI).vi"(4:"rpm"=w1286, 5:"rpm"=FALSE ("rpm"), "PrintTime"=FALSE, "Stop"=w1291, "error in (no error)"=w1284, "Time to wait"=3.0, "Strin"=w1285, "String in"=w1287) -> ("error out"=w1283:errorcluster)  [unwired: 1 in, 2 out]
          n464 = Increment(x=w1305) -> (x+1=w1299:i32)
          n465 = call "Serial.vi"("error in (no error)"=w1283, "write buffer"="VM[1]\r\n", "VISA resource name"=w1303) -> ("error out"=w1302:errorcluster, "read buffer"=w1297:string)  [unwired: 7 in]
          n466 = call "InsertSingleData.vi"("String In"=w1297, "error in (no error)"=w1302, "Col"=2, "Row"=w1299, "Table in"=w1300) -> ("error out"=w1301:errorcluster)  [unwired: 6 in]
          n467 = while {
            shift-right: [w1326] -> _
            shift-left: T7."VC=1000" -> [w1329]
            tunnel: w1301 -> [w1328]
            tunnel: w1303 -> [w1327]
            tunnel: w1285 -> [w1325]
            shift-right: [w1322] -> _
            shift-left: bool[] [FALSE, FALSE] -> [w1323]
            tunnel: w1299 -> [w1321]
            tunnel: w1300 -> [w1320]
            shift-right: [w1318] -> _
            shift-left: dbl[] [0.0, 0.0] -> [w1319]
            tunnel: w1297 -> [w1317]
            tunnel: [w1315] -> w1296
            i -> [w1324]
            stop <- w1316 stop-if-true
            n468 = case shown="\"Wait\"" w1329 {
              tunnel: w1328 -> [_ w1350 _ w1410 _]
              tunnel: w1327 -> [_ w1349 w1366 w1413 _]
              tunnel: [T7."Exit" T7."Wait" w1363 T7."Wait" T7."ReadVC"] -> w1326
              tunnel: w1325 -> [_ _ _ _ w1420]
              tunnel: [TRUE FALSE FALSE FALSE w1415] -> w1316
              tunnel: w1324 -> [_ _ w1364 _ _]
              tunnel: w1323 -> [w1334 w1347 w1362 w1411 w1417]
              tunnel: [w1334 w1347 w1361 w1411 w1417] -> w1322
              tunnel: w1321 -> [w1335 _ _ _ _]
              tunnel: w1320 -> [w1336 _ _ _ _]
              tunnel: w1319 -> [w1333 w1345 w1359 w1405 w1416]
              tunnel: [w1333 w1345 w1358 w1405 w1416] -> w1318
              tunnel: w1317 -> [_ _ w1357 _ _]
              tunnel: [_ _ _ _ w1415] -> w1315
              frame "Exit", Default {
                n469 = for {
                  tunnel: w1336 -> [w1344]
                  tunnel: w1335 -> [w1343]
                  tunnel: w1334 -> [w1342] mode=indexing
                  tunnel: w1333 -> [w1339] mode=indexing
                  i -> [w1340]
                  n470 = Add(x=w1340, y=w1343) -> (x+y=w1341:i32)
                  n471 = call "PassOrFail (SubVI).vi"("index (row)"=w1341, "Data in"=w1339, "Pass?Fail"=w1342, "Table in"=w1344) -> ()  [unwired: 7 in, 1 out]
                }
                n472 = local read "DAQmx Device Name"() -> (w1332:tag)
                n473 = call "Operation (SubVI).vi"("On/Off"=FALSE, "Operation"=T6."Venable", "DAQmx Device Name"=w1332) -> ()  [unwired: 8 in, 1 out]
              }
              frame "VC=0" {
                n474 = disable-structure shown="Enabled" {
                  disable-tunnel: w1350 -> [w1353 _]
                  disable-tunnel: w1349 -> [w1351 _]
                  frame Disabled {
                    n475 = call "Serial.vi"("error in (no error)"=w1353, "write buffer"="EP=1\r\nVC=0\r\n", "VISA resource name"=w1351) -> ()  [unwired: 7 in, 2 out]
                  }
                  frame Enabled {
                    n476 = local read "DAQmx Device Name"() -> (w1356:tag)
                    n477 = call "Operation (SubVI).vi"("On/Off"=TRUE, "Operation"=T6."Down", "DAQmx Device Name"=w1356) -> ()  [unwired: 8 in, 1 out]
                  }
                }
              }
              frame "ReadVC" {
                n478 = call "Serial.vi"("write buffer"="VC\r\n", "VISA resource name"=w1366) -> ("read buffer"=w1365:string)  [unwired: 8 in, 1 out]
                n479 = case shown="5, Default" w1364 {
                  tunnel: w1365 -> [w1384 w1397]
                  tunnel: [T7."VC=0" T7."Exit"] -> w1363
                  tunnel: w1362 -> [w1382 w1396]
                  tunnel: [w1380 w1393] -> w1361
                  tunnel: w1359 -> [w1379 w1392]
                  tunnel: [w1377 w1389] -> w1358
                  tunnel: w1357 -> [w1371 _]
                  frame 2 {
                    w1372 = 100
                    n480 = Decimal String To Number(string=w1384) -> (number=w1373:i32)  [unwired: 2 in, 1 out]
                    n481 = Decimal String To Number(string=w1371) -> (number=w1368:i32)  [unwired: 2 in, 1 out]
                    n482 = Add(x=w1368, y=w1372) -> (x+y=w1370:i32)
                    n483 = Subtract(x=w1368, y=w1372) -> (x-y=w1369:i32)
                    n484 = In Range and Coerce(upper limit=w1370, x=w1373, lower limit=w1369) -> (In Range?=w1381:bool)  [unwired: 1 out]
                    n485 = Replace Array Subset(array=w1379, new element=w1373, index=0) -> (w1377:dbl[])
                    n486 = Replace Array Subset(array=w1382, new element=w1381, index=0) -> (w1380:bool[])
                    n487 = local read "DAQmx Device Name"() -> (w1376:tag)
                    n488 = call "Operation (SubVI).vi"("On/Off"=FALSE, "Operation"=T6."Up", "DAQmx Device Name"=w1376) -> ()  [unwired: 8 in, 1 out]
                  }
                  frame 5, Default {
                    n489 = Decimal String To Number(string=w1397) -> (number=w1390:i32)  [unwired: 2 in, 1 out]
                    n490 = In Range and Coerce(upper limit=100, x=w1390, lower limit=0) -> (In Range?=w1394:bool)  [unwired: 1 out]
                    n491 = Replace Array Subset(array=w1392, new element=w1390, index=1) -> (w1389:dbl[])
                    n492 = Replace Array Subset(array=w1396, new element=w1394, index=1) -> (w1393:bool[])
                    n493 = local read "DAQmx Device Name"() -> (w1388:tag)
                    n494 = call "Operation (SubVI).vi"("On/Off"=FALSE, "Operation"=T6."Down", "DAQmx Device Name"=w1388) -> ()  [unwired: 8 in, 1 out]
                  }
                }
              }
              frame "VC=1000" {
                n495 = local read "DAQmx Device Name"() -> (w1404:tag)
                n496 = call "Operation (SubVI).vi"("error in (no error)"=w1410, "On/Off"=TRUE, "Operation"=T6."Venable", "DAQmx Device Name"=w1404) -> ("error out"=w1409:errorcluster)  [unwired: 7 in]
                n497 = call "Serial.vi"("error in (no error)"=w1409, "write buffer"="EP=1\r\nVC=0\r\n", "VISA resource name"=w1413) -> ("error out"=w1401:errorcluster)  [unwired: 7 in, 1 out]
                n498 = call "Operation (SubVI).vi"("error in (no error)"=w1401, "On/Off"=TRUE, "Operation"=T6."Up", "DAQmx Device Name"=w1404) -> ()  [unwired: 7 in, 1 out]
              }
              frame "Wait" {
                n499 = control-ref of="Motor Speed RPM Serial"() -> (w1425:refnum<vi>)
                n500 = control-ref of="Pannel User Message"() -> (w1424:refnum<vi>)
                n501 = control-ref of="Stop Button"() -> (w1419:refnum<vi>)
                n502 = call "Write panel message Kinetics (SubVI).vi"(4:"rpm"=w1425, 5:"rpm"=TRUE ("rpm"), "PrintTime"=TRUE, "Stop"=w1419, "Time to wait"=30.0, "Strin"=w1420, "String in"=w1424) -> ("Stopped"=w1415:bool)  [unwired: 2 in, 2 out]
              }
            }
          }
        }
        frame "Resistance Merkava 4 Test" {
          w1434 = T13 [enum."0 ohm", enum."6 ohm", enum."15 ohm"] items=["Init", "0 ohm", "6 ohm", "13.2 ohm", "15 ohm", "25.9 ohm", "33 ohm", "Down", "Up", "Venable", "Firmware", "PowerSuply"]
          w1438 = T13 [enum."6 ohm", enum."15 ohm", enum."15 ohm"] items=["Init", "0 ohm", "6 ohm", "13.2 ohm", "15 ohm", "25.9 ohm", "33 ohm", "Down", "Up", "Venable", "Firmware", "PowerSuply"]
          w1443 = T13 [enum."PowerSuply", enum."Down"] items=["Init", "0 ohm", "6 ohm", "13.2 ohm", "15 ohm", "25.9 ohm", "33 ohm", "Down", "Up", "Venable", "Firmware", "PowerSuply"]
          w1444 = T13 [enum."PowerSuply", enum."Venable", enum."Down", enum."0 ohm", enum."PowerSuply"] items=["Init", "0 ohm", "6 ohm", "13.2 ohm", "15 ohm", "25.9 ohm", "33 ohm", "Down", "Up", "Venable", "Firmware", "PowerSuply"]
          w1451 = T13 [enum."0 ohm", enum."6 ohm", enum."15 ohm"] items=["Init", "0 ohm", "6 ohm", "13.2 ohm", "15 ohm", "25.9 ohm", "33 ohm", "Down", "Up", "Venable", "Firmware", "PowerSuply"]
          # "1.65"
          n503 = control-ref of="Pannel User Message"() -> (w1457:refnum<vi>)
          n504 = Concatenate Strings(w1453, " in process..." ("Strin")) -> (w1445:string)
          n505 = property class="Str"(reference=w1457, error in=w1452, "Value"=w1445) -> (error out=w1456:errorcluster)  [unwired: 1 out]
          n506 = call "Table_ScrollaBarMarvin.vi"("error in"=w1456, "Line to focus"=w1453, "reference in"=w1447) -> ()  [unwired: 3 out]
          n507 = call "Reset old test Values (SubVI) Kinetics.vi"("Atr in"=w1447, "Test Paragraph"=w1453) -> ("error out"=w1455:errorcluster)  [unwired: 7 in, 2 out]
          n508 = call "Find_Number_LineMARVIN.vi"("Test Paragraph"=w1453, "error in"=w1455, "TableIn"=w1447) -> ("error out"=w1428:errorcluster, "Line number"=w1449:i32)  [unwired: 2 in, 2 out]
          n509 = disable-structure shown="Enabled" {
            disable-tunnel: [w1460 "CF[0]=4.5"] -> w1430
            disable-tunnel: w1428 -> [w1459 w1462]
            disable-tunnel: [w1458 w1462] -> w1427
            frame Disabled {
              n510 = call "Cable Length Param.vi"("error constant"=w1459) -> ("error out"=w1458:errorcluster, "Cable Length Param"=w1460:string)  [unwired: 9 in]
            }
            frame Enabled {
            }
          }
          n511 = for {
            tunnel: w1444 -> [w1473] mode=indexing
            tunnel: [w1471] -> w1446
            tunnel: w1427 -> [w1472]
            tunnel: [w1468] -> w1426
            tunnel: bool[] [FALSE, TRUE, TRUE, TRUE, TRUE] -> [w1470] mode=indexing
            tunnel: dbl[] [5.0, 0.2, 0.2, 0.2, 3.0] -> [w1467] mode=indexing
            n512 = local read "DAQmx Device Name"() -> (w1471:tag)
            n513 = call "Operation (SubVI).vi"("error in (no error)"=w1472, "On/Off"=w1470, "Operation"=w1473, "DAQmx Device Name"=w1471) -> ("error out"=w1469:errorcluster)  [unwired: 7 in]
            n514 = call "Time Delay6"("error in (no error)"=w1469, "Delay Time (s)"=w1467) -> ("error out"=w1468:errorcluster)  [unwired: 9 in]
          }
          n515 = Concatenate Strings("EP=1\r\n" ("write buffer"), w1430, "\r\n" ("string")) -> (w1429:string)
          n516 = call "Serial.vi"("error in (no error)"=w1426, "write buffer"=w1429, "VISA resource name"=w1441) -> ("error out"=w1442:errorcluster)  [unwired: 7 in, 1 out]
          n517 = Increment(x=w1449) -> (x+1=w1448:i32)
          n518 = for {
            tunnel: w1451 -> [w1480] mode=indexing
            tunnel: i32[] [6850, 8300, 9200] -> [w1496] mode=indexing
            tunnel: w1448 -> [w1491]
            tunnel: w1447 -> [w1486]
            tunnel: w1442 -> [w1485]
            tunnel: w1446 -> [w1484]
            tunnel: w1445 -> [w1483]
            tunnel: bool[] [TRUE, TRUE, TRUE] -> [w1482] mode=indexing
            tunnel: w1438 -> [w1477] mode=indexing
            tunnel: [w1481] -> w1436
            tunnel: bool[] [TRUE, FALSE] -> [w1479]
            tunnel: w1434 -> [w1476] mode=indexing
            tunnel: [w1475] -> w1433
            i -> [w1492]
            stop <- w1481 stop-if-true
            w1495 = 100 ("x")
            n519 = Add(x=w1491, y=w1492) -> (x+y=w1490:i32)
            n520 = call "Operation (SubVI).vi"("error in (no error)"=w1485, "On/Off"=w1482, "Operation"=w1480, "DAQmx Device Name"=w1484) -> ("error out"=w1498:errorcluster)  [unwired: 7 in]
            n521 = control-ref of="Motor Speed RPM Serial"() -> (w1499:refnum<vi>)
            n522 = control-ref of="Pannel User Message"() -> (w1501:refnum<vi>)
            n523 = control-ref of="Stop Button"() -> (w1504:refnum<vi>)
            n524 = call "Write panel message Kinetics (SubVI).vi"(4:"rpm"=w1499, 5:"rpm"=TRUE ("rpm"), "PrintTime"=TRUE, "Stop"=w1504, "error in (no error)"=w1498, "Time to wait"=30.0, "Strin"=w1483, "String in"=w1501) -> ("error out"=w1497:errorcluster, "Stopped"=w1481:bool)  [unwired: 1 in, 1 out]
            n525 = property on="Motor Speed RPM Serial" class="DigNum (strict)"(error in=w1497) -> (error out=w1489:errorcluster, "Value"=w1488:dbl)  [unwired: 1 in, 1 out]
            n526 = Subtract(x=w1496, y=w1495) -> (x-y=w1493:i32)
            n527 = Add(x=w1495, y=w1496) -> (x+y=w1494:i32)
            n528 = In Range and Coerce(upper limit=w1494, x=w1488, lower limit=w1493) -> (In Range?=w1487:bool)  [unwired: 1 out]
            n529 = call "PassOrFail (SubVI).vi"("index (row)"=w1490, "error in (no error)"=w1489, "Data in"=w1488, "Pass?Fail"=w1487, "Table in"=w1486) -> ("error out"=w1474:errorcluster)  [unwired: 6 in]
            n530 = Build Array(w1477, w1476) -> (w1478:T13)
            n531 = for {
              tunnel: w1484 -> [w1510]
              tunnel: w1479 -> [w1509] mode=indexing
              tunnel: w1478 -> [w1508] mode=indexing
              tunnel: [w1506] -> w1475
              tunnel: w1474 -> [w1505]
              n532 = call "Operation (SubVI).vi"("error in (no error)"=w1505, "On/Off"=w1509, "Operation"=w1508, "DAQmx Device Name"=w1510) -> ("error out"=w1507:errorcluster)  [unwired: 7 in]
              n533 = call "Time Delay5"("error in (no error)"=w1507) -> ("error out"=w1506:errorcluster)  [unwired: 10 in]
            }
          }
          n534 = for {
            tunnel: w1433 -> [w1464]
            tunnel: w1443 -> [w1463] mode=indexing
            n535 = local read "DAQmx Device Name"() -> (w1465:tag)
            n536 = call "Operation (SubVI).vi"("error in (no error)"=w1464, "On/Off"=FALSE, "Operation"=w1463, "DAQmx Device Name"=w1465) -> ()  [unwired: 7 in, 1 out]
          }
        }
        frame "Resistance Merkava 3 Test" {
          w1520 = T13 [enum."0 ohm", enum."13.2 ohm", enum."33 ohm"] items=["Init", "0 ohm", "6 ohm", "13.2 ohm", "15 ohm", "25.9 ohm", "33 ohm", "Down", "Up", "Venable", "Firmware", "PowerSuply"]
          w1524 = T13 [enum."13.2 ohm", enum."33 ohm", enum."33 ohm"] items=["Init", "0 ohm", "6 ohm", "13.2 ohm", "15 ohm", "25.9 ohm", "33 ohm", "Down", "Up", "Venable", "Firmware", "PowerSuply"]
          w1527 = T13 [enum."PowerSuply", enum."Venable", enum."Up", enum."0 ohm", enum."PowerSuply"] items=["Init", "0 ohm", "6 ohm", "13.2 ohm", "15 ohm", "25.9 ohm", "33 ohm", "Down", "Up", "Venable", "Firmware", "PowerSuply"]
          (unwired) "EP=1\r\nCF[0]=4.5\r\n" ("write buffer")
          w1530 = T13 [enum."PowerSuply", enum."Up"] items=["Init", "0 ohm", "6 ohm", "13.2 ohm", "15 ohm", "25.9 ohm", "33 ohm", "Down", "Up", "Venable", "Firmware", "PowerSuply"]
          w1536 = T13 [enum."0 ohm", enum."13.2 ohm", enum."33 ohm"] items=["Init", "0 ohm", "6 ohm", "13.2 ohm", "15 ohm", "25.9 ohm", "33 ohm", "Down", "Up", "Venable", "Firmware", "PowerSuply"]
          # "6.5"
          n537 = control-ref of="Pannel User Message"() -> (w1542:refnum<vi>)
          n538 = Concatenate Strings(w1538, " in process..." ("Strin")) -> (w1511:string)
          n539 = property class="Str"(reference=w1542, error in=w1537, "Value"=w1511) -> (error out=w1541:errorcluster)  [unwired: 1 out]
          n540 = call "Table_ScrollaBarMarvin.vi"("error in"=w1541, "Line to focus"=w1538, "reference in"=w1532) -> ()  [unwired: 3 out]
          n541 = call "Reset old test Values (SubVI) Kinetics.vi"("Atr in"=w1532, "Test Paragraph"=w1538) -> ("error out"=w1540:errorcluster)  [unwired: 7 in, 2 out]
          n542 = call "Find_Number_LineMARVIN.vi"("Test Paragraph"=w1538, "error in"=w1540, "TableIn"=w1532) -> ("error out"=w1513:errorcluster, "Line number"=w1534:i32)  [unwired: 2 in, 2 out]
          n543 = disable-structure shown="Enabled" {
            disable-tunnel: [w1545 "CF[0]=4.5"] -> w1517
            disable-tunnel: w1513 -> [w1544 w1547]
            disable-tunnel: [w1543 w1547] -> w1512
            frame Disabled {
              n544 = call "Cable Length Param.vi"("error constant"=w1544) -> ("error out"=w1543:errorcluster, "Cable Length Param"=w1545:string)  [unwired: 9 in]
            }
            frame Enabled {
            }
          }
          n545 = for {
            tunnel: [w1557] -> w1531
            tunnel: w1512 -> [w1558]
            tunnel: [w1553] -> w1514
            tunnel: w1527 -> [w1556] mode=indexing
            tunnel: bool[] [FALSE, TRUE, TRUE, TRUE, TRUE] -> [w1555] mode=indexing
            tunnel: dbl[] [10.0, 0.2, 0.2, 0.2, 3.0] -> [w1552] mode=indexing
            n546 = local read "DAQmx Device Name"() -> (w1557:tag)
            n547 = call "Operation (SubVI).vi"("error in (no error)"=w1558, "On/Off"=w1555, "Operation"=w1556, "DAQmx Device Name"=w1557) -> ("error out"=w1554:errorcluster)  [unwired: 7 in]
            n548 = call "Time Delay7"("error in (no error)"=w1554, "Delay Time (s)"=w1552) -> ("error out"=w1553:errorcluster)  [unwired: 9 in]
          }
          n549 = Concatenate Strings("EP=1\r\n" ("write buffer"), w1517, "\r\n" ("string")) -> (w1515:string)
          n550 = Increment(x=w1534) -> (x+1=w1533:i32)
          n551 = call "Serial.vi"("error in (no error)"=w1514, "write buffer"=w1515, "VISA resource name"=w1529) -> ("error out"=w1528:errorcluster)  [unwired: 7 in, 1 out]
          n552 = for {
            tunnel: w1536 -> [w1570] mode=indexing
            tunnel: i32[] [6850, 9000, 9980] -> [w1581] mode=indexing
            tunnel: w1533 -> [w1576]
            tunnel: w1532 -> [w1571]
            tunnel: w1528 -> [w1569]
            tunnel: w1531 -> [w1568]
            tunnel: w1511 -> [w1567]
            tunnel: bool[] [TRUE, TRUE, TRUE] -> [w1566] mode=indexing
            tunnel: w1524 -> [w1563] mode=indexing
            tunnel: [w1565] -> w1522
            tunnel: bool[] [TRUE, FALSE] -> [w1564]
            tunnel: w1520 -> [w1562] mode=indexing
            tunnel: [w1560] -> w1519
            i -> [w1577]
            stop <- w1565 stop-if-true
            w1580 = 100 ("x")
            n553 = Add(x=w1576, y=w1577) -> (x+y=w1575:i32)
            n554 = call "Operation (SubVI).vi"("error in (no error)"=w1569, "On/Off"=w1566, "Operation"=w1570, "DAQmx Device Name"=w1568) -> ("error out"=w1583:errorcluster)  [unwired: 7 in]
            n555 = control-ref of="Motor Speed RPM Serial"() -> (w1584:refnum<vi>)
            n556 = control-ref of="Pannel User Message"() -> (w1586:refnum<vi>)
            n557 = control-ref of="Stop Button"() -> (w1589:refnum<vi>)
            n558 = call "Write panel message Kinetics (SubVI).vi"(4:"rpm"=w1584, 5:"rpm"=TRUE ("rpm"), "PrintTime"=TRUE, "Stop"=w1589, "error in (no error)"=w1583, "Time to wait"=30.0, "Strin"=w1567, "String in"=w1586) -> ("error out"=w1582:errorcluster, "Stopped"=w1565:bool)  [unwired: 1 in, 1 out]
            n559 = property on="Motor Speed RPM Serial" class="DigNum (strict)"(error in=w1582) -> (error out=w1574:errorcluster, "Value"=w1573:dbl)  [unwired: 1 in, 1 out]
            n560 = Subtract(x=w1581, y=w1580) -> (x-y=w1578:i32)
            n561 = Add(x=w1580, y=w1581) -> (x+y=w1579:i32)
            n562 = In Range and Coerce(upper limit=w1579, x=w1573, lower limit=w1578) -> (In Range?=w1572:bool)  [unwired: 1 out]
            n563 = Build Array(w1563, w1562) -> (w1561:T13)
            n564 = call "PassOrFail (SubVI).vi"("index (row)"=w1575, "error in (no error)"=w1574, "Data in"=w1573, "Pass?Fail"=w1572, "Table in"=w1571) -> ("error out"=w1559:errorcluster)  [unwired: 6 in]
            n565 = for {
              tunnel: w1568 -> [w1595]
              tunnel: w1564 -> [w1594] mode=indexing
              tunnel: w1561 -> [w1593] mode=indexing
              tunnel: [w1591] -> w1560
              tunnel: w1559 -> [w1590]
              n566 = call "Operation (SubVI).vi"("error in (no error)"=w1590, "On/Off"=w1594, "Operation"=w1593, "DAQmx Device Name"=w1595) -> ("error out"=w1592:errorcluster)  [unwired: 7 in]
              n567 = call "Time Delay2"("error in (no error)"=w1592) -> ("error out"=w1591:errorcluster)  [unwired: 10 in]
            }
          }
          n568 = for {
            tunnel: w1519 -> [w1549]
            tunnel: w1530 -> [w1548] mode=indexing
            n569 = local read "DAQmx Device Name"() -> (w1550:tag)
            n570 = call "Operation (SubVI).vi"("error in (no error)"=w1549, "On/Off"=FALSE, "Operation"=w1548, "DAQmx Device Name"=w1550) -> ()  [unwired: 7 in, 1 out]
          }
        }
        frame "Resistance Namer Test" {
          w1604 = T13 [enum."13.2 ohm", enum."25.9 ohm", enum."33 ohm"] items=["Init", "0 ohm", "6 ohm", "13.2 ohm", "15 ohm", "25.9 ohm", "33 ohm", "Down", "Up", "Venable", "Firmware", "PowerSuply"]
          w1605 = T13 [enum."25.9 ohm", enum."33 ohm", enum."33 ohm"] items=["Init", "0 ohm", "6 ohm", "13.2 ohm", "15 ohm", "25.9 ohm", "33 ohm", "Down", "Up", "Venable", "Firmware", "PowerSuply"]
          w1611 = T13 [enum."Init", enum."PowerSuply", enum."Venable", enum."Down", enum."Up", enum."13.2 ohm", enum."PowerSuply", enum."Down", enum."Up"] items=["Init", "0 ohm", "6 ohm", "13.2 ohm", "15 ohm", "25.9 ohm", "33 ohm", "Down", "Up", "Venable", "Firmware", "PowerSuply"]
          (unwired) "EP=1\r\nCF[0]=4.5\r\n" ("write buffer")
          w1614 = T13 [enum."Init", enum."Down", enum."Up"] items=["Init", "0 ohm", "6 ohm", "13.2 ohm", "15 ohm", "25.9 ohm", "33 ohm", "Down", "Up", "Venable", "Firmware", "PowerSuply"]
          w1620 = T13 [enum."13.2 ohm", enum."25.9 ohm", enum."33 ohm"] items=["Init", "0 ohm", "6 ohm", "13.2 ohm", "15 ohm", "25.9 ohm", "33 ohm", "Down", "Up", "Venable", "Firmware", "PowerSuply"]
          n571 = control-ref of="Pannel User Message"() -> (w1626:refnum<vi>)
          n572 = Concatenate Strings(w1622, " in process..." ("Strin")) -> (w1615:string)
          n573 = property class="Str"(reference=w1626, error in=w1621, "Value"=w1615) -> (error out=w1625:errorcluster)  [unwired: 1 out]
          n574 = call "Table_ScrollaBarMarvin.vi"("error in"=w1625, "Line to focus"=w1622, "reference in"=w1616) -> ()  [unwired: 3 out]
          n575 = call "Reset old test Values (SubVI) Kinetics.vi"("Atr in"=w1616, "Test Paragraph"=w1622) -> ("error out"=w1624:errorcluster)  [unwired: 7 in, 2 out]
          n576 = call "Find_Number_LineMARVIN.vi"("Test Paragraph"=w1622, "error in"=w1624, "TableIn"=w1616) -> ("error out"=w1597:errorcluster, "Line number"=w1618:i32)  [unwired: 2 in, 2 out]
          n577 = disable-structure shown="Enabled" {
            disable-tunnel: [w1629 "CF[0]=4.5"] -> w1602
            disable-tunnel: w1597 -> [w1628 w1631]
            disable-tunnel: [w1627 w1631] -> w1596
            frame Disabled {
              n578 = call "Cable Length Param.vi"("error constant"=w1628) -> ("error out"=w1627:errorcluster, "Cable Length Param"=w1629:string)  [unwired: 9 in]
            }
            frame Enabled {
            }
          }
          n579 = for {
            tunnel: [w1641] -> w1608
            tunnel: w1596 -> [w1642]
            tunnel: [w1638] -> w1598
            tunnel: w1611 -> [w1640] mode=indexing
            tunnel: dbl[] [1.0, 10.0, 0.2, 0.2, 0.2, 0.2, 5.0, 0.2, 0.2] -> [w1637] mode=indexing
            tunnel: bool[] [FALSE, FALSE, TRUE, TRUE, TRUE, TRUE, TRUE, TRUE, TRUE] -> [w1636] mode=indexing
            n580 = local read "DAQmx Device Name"() -> (w1641:tag)
            n581 = call "Operation (SubVI).vi"("error in (no error)"=w1642, "On/Off"=w1636, "Operation"=w1640, "DAQmx Device Name"=w1641) -> ("error out"=w1639:errorcluster)  [unwired: 7 in]
            n582 = call "Time Delay10"("error in (no error)"=w1639, "Delay Time (s)"=w1637) -> ("error out"=w1638:errorcluster)  [unwired: 9 in]
          }
          n583 = Concatenate Strings("EP=1\r\n" ("write buffer"), w1602, "\r\n" ("string")) -> (w1599:string)
          n584 = call "Serial.vi"("error in (no error)"=w1598, "write buffer"=w1599, "VISA resource name"=w1607) -> ("error out"=w1613:errorcluster)  [unwired: 7 in, 1 out]
          n585 = Increment(x=w1618) -> (x+1=w1617:i32)
          n586 = for {
            tunnel: w1620 -> [w1649] mode=indexing
            tunnel: i32[] [8350, 8900, 9450] -> [w1664] mode=indexing
            tunnel: w1617 -> [w1659]
            tunnel: w1616 -> [w1654]
            tunnel: w1613 -> [w1653]
            tunnel: w1608 -> [w1652]
            tunnel: w1615 -> [w1651]
            tunnel: [w1650] -> w1609
            tunnel: bool[] [TRUE, FALSE] -> [w1648]
            tunnel: w1605 -> [w1647] mode=indexing
            tunnel: w1604 -> [w1646] mode=indexing
            tunnel: [w1644] -> w1603
            i -> [w1660]
            stop <- w1650 stop-if-true
            w1663 = 100 ("x")
            n587 = Add(x=w1659, y=w1660) -> (x+y=w1658:i32)
            n588 = call "Operation (SubVI).vi"("error in (no error)"=w1653, "On/Off"=TRUE, "Operation"=w1649, "DAQmx Device Name"=w1652) -> ("error out"=w1666:errorcluster)  [unwired: 7 in]
            n589 = control-ref of="Motor Speed RPM Serial"() -> (w1667:refnum<vi>)
            n590 = control-ref of="Pannel User Message"() -> (w1669:refnum<vi>)
            n591 = control-ref of="Stop Button"() -> (w1672:refnum<vi>)
            n592 = call "Write panel message Kinetics (SubVI).vi"(4:"rpm"=w1667, 5:"rpm"=TRUE ("rpm"), "PrintTime"=TRUE, "Stop"=w1672, "error in (no error)"=w1666, "Time to wait"=30.0, "Strin"=w1651, "String in"=w1669) -> ("error out"=w1665:errorcluster, "Stopped"=w1650:bool)  [unwired: 1 in, 1 out]
            n593 = property on="Motor Speed RPM Serial" class="DigNum (strict)"(error in=w1665) -> (error out=w1657:errorcluster, "Value"=w1656:dbl)  [unwired: 1 in, 1 out]
            n594 = Subtract(x=w1664, y=w1663) -> (x-y=w1661:i32)
            n595 = Add(x=w1663, y=w1664) -> (x+y=w1662:i32)
            n596 = In Range and Coerce(upper limit=w1662, x=w1656, lower limit=w1661) -> (In Range?=w1655:bool)  [unwired: 1 out]
            n597 = Build Array(w1647, w1646) -> (w1645:T13)
            n598 = call "PassOrFail (SubVI).vi"("index (row)"=w1658, "error in (no error)"=w1657, "Data in"=w1656, "Pass?Fail"=w1655, "Table in"=w1654) -> ("error out"=w1643:errorcluster)  [unwired: 6 in]
            n599 = for {
              tunnel: w1652 -> [w1679]
              tunnel: w1648 -> [w1678] mode=indexing
              tunnel: w1645 -> [w1677] mode=indexing
              tunnel: [w1675] -> w1644
              tunnel: w1643 -> [w1674]
              n600 = call "Operation (SubVI).vi"("error in (no error)"=w1674, "On/Off"=w1678, "Operation"=w1677, "DAQmx Device Name"=w1679) -> ("error out"=w1676:errorcluster)  [unwired: 7 in]
              n601 = call "Time Delay13"("error in (no error)"=w1676) -> ("error out"=w1675:errorcluster)  [unwired: 10 in]
            }
          }
          n602 = for {
            tunnel: w1603 -> [w1633]
            tunnel: w1614 -> [w1632] mode=indexing
            n603 = local read "DAQmx Device Name"() -> (w1634:tag)
            n604 = call "Operation (SubVI).vi"("error in (no error)"=w1633, "On/Off"=FALSE, "Operation"=w1632, "DAQmx Device Name"=w1634) -> ()  [unwired: 7 in, 1 out]
          }
        }
        frame "Analog Voltage Test" {
          w1689 = T13 [enum."Init", enum."PowerSuply"] items=["Init", "0 ohm", "6 ohm", "13.2 ohm", "15 ohm", "25.9 ohm", "33 ohm", "Down", "Up", "Venable", "Firmware", "PowerSuply"]
          n605 = control-ref of="Pannel User Message"() -> (w1716:refnum<vi>)
          n606 = Concatenate Strings(w1710, " in process..." ("string")) -> (w1695:string)
          n607 = property class="Str"(reference=w1716, error in=w1712, "Value"=w1695) -> (error out=w1715:errorcluster)  [unwired: 1 out]
          n608 = call "Table_ScrollaBarMarvin.vi"("error in"=w1715, "Line to focus"=w1710, "reference in"=w1711) -> ("error out"=w1714:errorcluster)  [unwired: 2 out]
          n609 = local read "DAQmx Device Name"() -> (w1687:tag)
          n610 = call "Find_Number_LineMARVIN.vi"("Test Paragraph"=w1710, "error in"=w1714, "TableIn"=w1711) -> ("error out"=w1718:errorcluster, "Line number"=w1717:i32)  [unwired: 2 in, 2 out]
          n611 = call <vilib>:"Clear Errors.vi"("error in (no error)"=w1718) -> ("error out"=w1709:errorcluster)  [unwired: 5 in, 1 out]
          n612 = call "Reset old test Values (SubVI) Kinetics.vi"("error in"=w1709, "Atr in"=w1711, "Test Paragraph"=w1710) -> ("error out"=w1703:errorcluster)  [unwired: 6 in, 2 out]
          n613 = for {
            tunnel: w1687 -> [w2195]
            tunnel: w1689 -> [w2194] mode=indexing
            tunnel: bool[] [FALSE, TRUE] -> [w2193] mode=indexing
            shift-right: [w2192] -> w1700
            shift-left: w1703 -> [w2196]
            n614 = call "Operation (SubVI).vi"("error in (no error)"=w2196, "On/Off"=w2193, "Operation"=w2194, "DAQmx Device Name"=w2195) -> ("error out"=w2192:errorcluster)  [unwired: 7 in]
          }
          n615 = local read "DAQmx Device Name"() -> (w1681:tag)
          n616 = control-ref of="Pannel User Message"() -> (w1702:refnum<vi>)
          n617 = control-ref of="Motor Speed RPM Serial"() -> (w1698:refnum<vi>)
          n618 = control-ref of="Stop Button"() -> (w1696:refnum<vi>)
          n619 = call "Write panel message Kinetics (SubVI).vi"(4:"rpm"=w1698, 5:"rpm"=FALSE ("rpm"), "PrintTime"=FALSE, "Stop"=w1696, "error in (no error)"=w1700, "Time to wait"=5.0, "Strin"=w1695, "String in"=w1702) -> ("error out"=w1694:errorcluster)  [unwired: 1 in, 2 out]
          n620 = call "Serial.vi"("error in (no error)"=w1694, "write buffer"="EP=1\r\nVC=0\r\n", "VISA resource name"=w1693) -> ("error out"=w1691:errorcluster)  [unwired: 7 in, 1 out]
          n621 = while {
            tunnel: [w2199] -> w1688
            tunnel: [TRUE] -> w1692
            tunnel: w1691 -> [w2197]
            stop <- w2201 stop-if-true
            n622 = control-ref of="Motor Speed RPM Serial"() -> (w2203:refnum<vi>)
            n623 = property class="DigNum (strict)"(reference=w2203, error in=w2197) -> (error out=w2199:errorcluster, "Value"=w2202:dbl)  [unwired: 1 out]
            n624 = Less Or Equal?(x=w2202, y=50.0) -> (x <= y?=w2201:bool)
          }
          "Analogtest" <- w1692
          n625 = call "Operation (SubVI).vi"("error in (no error)"=w1688, "On/Off"=FALSE, "Operation"=T6."PowerSuply", "DAQmx Device Name"=w1687) -> ("error out"=w1684:errorcluster)  [unwired: 7 in]
          n626 = call "Time Delay14"("error in (no error)"=w1684, "Delay Time (s)"=20.0) -> ("error out"=w1683:errorcluster)  [unwired: 9 in]
          n627 = for {
            N: 2 -> [_]
            tunnel: w1717 -> [w1727]
            tunnel: w1711 -> [w1726]
            tunnel: [w1725] -> w1705
            tunnel: w1695 -> [w1724]
            tunnel: w1693 -> [w1723]
            tunnel: w1681 -> [w1721]
            shift-right: [w1720] -> w1706
            shift-left: w1683 -> [w1722]
            i -> [w1719]
            n628 = case shown="0" w1719 {
              tunnel: w1727 -> [w1741 w1955 _]
              tunnel: w1726 -> [w1740 w1954 _]
              tunnel: [w1736 w1950 FALSE ("Stopped")] -> w1725
              tunnel: w1724 -> [w1735 w1949 _]
              tunnel: w1723 -> [w1734 w1948 _]
              tunnel: w1722 -> [w1733 w1947 w2191]
              tunnel: w1721 -> [w1732 w1946 _]
              tunnel: [w1730 w1945 w2191] -> w1720
              frame 0 {
                w1739 = dbl[] [1.0, 4.0]
                n629 = for {
                  tunnel: w1739 -> [w1752] mode=indexing
                  tunnel: w1734 -> [w1751]
                  tunnel: w1740 -> [w1750]
                  tunnel: w1733 -> [w1745]
                  tunnel: w1741 -> [w1749]
                  tunnel: w1739 -> [w1748]
                  tunnel: w1735 -> [w1747]
                  tunnel: [w1745] -> w1738
                  shift-right: [w1744] -> _
                  shift-left: T11."Init" -> [w1753]
                  tunnel: [w1743] -> w1736
                  tunnel: w1732 -> [w1742]
                  i -> [w1746]
                  n630 = while {
                    shift-right: [w1759] -> w1744
                    shift-left: w1753 -> [w1765]
                    tunnel: w1752 -> [w1764]
                    tunnel: w1751 -> [w1763]
                    tunnel: w1750 -> [w1762]
                    tunnel: w1749 -> [w1761]
                    tunnel: w1748 -> [w1760]
                    tunnel: w1747 -> [w1758]
                    tunnel: w1746 -> [w1757]
                    tunnel: [w1755] -> w1743
                    tunnel: w1742 -> [w1754]
                    stop <- w1756 stop-if-true
                    n631 = case shown="\"Wait\"" w1765 {
                      tunnel: w1764 -> [_ _ w1781 w1791 _ _]
                      tunnel: w1763 -> [_ _ w1780 w1792 _ w1924]
                      tunnel: w1762 -> [_ _ _ _ _ _]
                      tunnel: w1761 -> [_ w1774 _ _ _ _]
                      tunnel: w1760 -> [_ _ _ _ _ _]
                      tunnel: [T11."AO0" T11."Exit" T11."Wait" T11."Exit" T11."Read" w1926] -> w1759
                      tunnel: [TRUE _ _ w1794 TRUE w1920] -> w1756
                      tunnel: w1758 -> [_ _ _ w1801 _ _]
                      tunnel: w1757 -> [_ w1770 w1778 w1789 _ _]
                      tunnel: [_ _ _ w1794 _ w1920] -> w1755
                      tunnel: w1754 -> [_ w1769 w1782 _ _ w1928]
                      frame "Exit", Default {
                      }
                      frame "AI0/3" {
                        n632 = Increment(x=w1774) -> (x+1=w1773:i32)
                        n633 = property on="Motor Speed RPM Serial" class="DigNum (strict)"() -> ("Value"=w1775:dbl)  [unwired: 2 in, 2 out]
                        n634 = Multiply(x=w1770, y=2) -> (x*y=w1772:i32)
                        n635 = call "Aquire AI"("device name"=w1769) -> ("data"=w1776:dynamicdata)  [unwired: 16 in, 2 out]
                        n636 = Add(x=w1773, y=w1772) -> ()  [unwired: 1 out]
                        n637 = To Double Precision Float(number=w1776) -> (double precision float=w1768:dbl)
                        n638 = Build Array(w1768, w1775) -> ()  [unwired: 1 out]
                      }
                      frame "AO0" {
                        n639 = call "Generate AO2"("data"=w1781, "device name"=w1782) -> ("error out"=w1779:errorcluster)  [unwired: 16 in, 1 out]
                        n640 = case shown="0, Default" w1778 {
                          tunnel: w1780 -> [w1786 _]
                          tunnel: w1779 -> [_ _]
                          frame 0, Default {
                            n641 = call "Serial.vi"("write buffer"="AO[0]\r\n", "VISA resource name"=w1786) -> ("read buffer"=w1787:string)  [unwired: 8 in, 1 out]
                            n642 = Fract/Exp String To Number(string=w1787, default (0 dbl)=sgl 0.0 ("default (0 DBL)")) -> (number=→"AO[0]":sgl)  [unwired: 2 in, 1 out]
                          }
                          frame 1 {
                          }
                        }
                      }
                      frame "Wait" {
                        n643 = Number To Fractional String(number=w1791, precision (6)=i16 1) -> (F-format string=w1796:string)  [unwired: 2 in]
                        n644 = Concatenate Strings(w1801, "\r\n", "Analog Output: ", w1796, "V." ("string")) -> (w1795:string)
                        n645 = control-ref of="Motor Speed RPM Serial"() -> (w1802:refnum<vi>)
                        n646 = control-ref of="Pannel User Message"() -> (w1803:refnum<vi>)
                        n647 = control-ref of="Stop Button"() -> (w1807:refnum<vi>)
                        n648 = call "Write panel message Kinetics (SubVI).vi"(4:"rpm"=w1802, 5:"rpm"=TRUE ("rpm"), "PrintTime"=TRUE, "Stop"=w1807, "Time to wait"=20.0, "Strin"=w1795, "String in"=w1803) -> ("error out"=w1793:errorcluster, "Stopped"=w1794:bool)  [unwired: 2 in, 1 out]
                        n649 = case shown="True" TRUE {
                          tunnel: w1793 -> [_ _]
                          tunnel: w1792 -> [_ w1811]
                          tunnel: w1789 -> [_ w1809]
                          frame False {
                          }
                          frame True {
                            n650 = while {
                              shift-right: [w1820] -> _
                              shift-left: "INIT" ("string") -> [w1822]
                              shift-right: [w1819] -> _
                              shift-left: 0.0 ("upper limit") -> [w1818]
                              tunnel: w1811 -> [w1817]
                              shift-right: [w1815] -> _
                              shift-left: 0 -> [w1816]
                              tunnel: w1809 -> [w1814]
                              stop <- w1821 stop-if-true
                              n651 = case shown="\"ADJ\"" w1822 {
                                selector: w1822 -> [_ _ _ _ w1906]
                                tunnel: [FALSE FALSE FALSE w1891 TRUE] -> w1821
                                tunnel: ["INIT" ("string") w1841 "Wait" ("string") "INIT" ("string") w1906] -> w1820
                                tunnel: [w1826 w1838 w1866 w1888 w1901] -> w1819
                                tunnel: w1818 -> [w1826 _ w1866 _ w1901]
                                tunnel: w1817 -> [_ _ w1865 _ w1903]
                                tunnel: w1816 -> [w1823 w1832 w1864 w1889 w1904]
                                tunnel: [w1823 w1832 w1863 w1889 w1904] -> w1815
                                tunnel: w1814 -> [_ w1828 w1860 _ w1902]
                                frame Default {
                                }
                                frame "INIT" {
                                n652 = control-ref of="Motor Speed RPM Serial"() -> (w1839:refnum<vi>)
                                n653 = control-ref of="Pannel User Message"() -> (w1850:refnum<vi>)
                                n654 = control-ref of="Stop Button"() -> (w1846:refnum<vi>)
                                n655 = call "Write panel message Kinetics (SubVI).vi"(4:"rpm"=w1839, 5:"rpm"=TRUE ("rpm"), "PrintTime"=FALSE, "Stop"=w1846, "Time to wait"=0.2, "Strin"="Adjusting AO[0], Please Wait...", "String in"=w1850) -> ("RPM"=w1838:dbl, "Stopped"=w1844:bool)  [unwired: 2 in, 1 out]
                                n656 = case shown="0, Default" w1828 {
                                tunnel: [2450.0 ("upper limit") 9650.0 ("upper limit")] -> w1837
                                tunnel: [2350.0 ("lower limit") 9550.0 ("lower limit")] -> w1836
                                frame 0, Default {
                                }
                                frame 1 {
                                }
                                }
                                n657 = property on="AO[0]" class="DigNum (strict)"() -> ("Value"=w1827:sgl)  [unwired: 2 in, 2 out]
                                n658 = In Range and Coerce(upper limit=w1837, x=w1838, lower limit=w1836) -> (In Range?=w1829:bool)  [unwired: 1 out]
                                n659 = Equal?(x=w1832, y=5) -> (x = y?=w1833:bool)
                                n660 = Compound Arithmetic op=OR(w1833, w1844, w1829) -> (w1834:bool)
                                n661 = Equal To 0?(x=w1832) -> (x = 0?=w1831:bool)
                                n662 = And(x=w1831, y=w1829) -> (x .and. y?=w1830:bool)
                                n663 = Select(t="Stop" ("string"), s=w1834, f="ADJ" ("string")) -> (s? t:f=w1841:string)
                                n664 = case shown="True" w1830 {
                                tunnel: w1828 -> [_ w1852]
                                tunnel: w1827 -> [_ w1851]
                                frame False {
                                }
                                frame True {
                                n665 = case shown="0, Default" w1852 {
                                tunnel: w1851 -> [w1853 w1854]
                                frame 0, Default {
                                n666 = property on="AO[0] 1" class="DigNum (strict)"("Value"=w1853) -> ()  [unwired: 2 in, 2 out]
                                }
                                frame 1 {
                                n667 = property on="AO[0] 2" class="DigNum (strict)"("Value"=w1854) -> ()  [unwired: 2 in, 2 out]
                                }
                                }
                                }
                                }
                                }
                                frame "ADJ" {
                                n668 = case shown="0, Default" w1860 {
                                tunnel: [2350.0 ("y") 9550.0 ("y")] -> w1871
                                frame 0, Default {
                                }
                                frame 1 {
                                }
                                }
                                n669 = property on="AO[0]" class="DigNum (strict)"() -> ("Value"=w1861:sgl)  [unwired: 2 in, 2 out]
                                n670 = Less?(x=w1866, y=w1871) -> (x < y?=w1870:bool)
                                n671 = case shown="False" w1870 {
                                tunnel: w1861 -> [w1882 w1887]
                                tunnel: [w1881 w1885] -> w1859
                                tunnel: w1864 -> [w1879 w1884]
                                tunnel: [w1878 w1883] -> w1863
                                frame False {
                                n672 = Increment(x=w1879) -> (x+1=w1878:i32)
                                n673 = Add(x=w1882, y=sgl 0.0075) -> (x+y=w1881:sgl)
                                }
                                frame True {
                                n674 = Increment(x=w1884) -> (x+1=w1883:i32)
                                n675 = Subtract(x=w1887, y=sgl 0.0075) -> (x-y=w1885:sgl)
                                }
                                }
                                n676 = Number To Fractional String(number=w1859) -> (F-format string=w1869:string)  [unwired: 3 in]
                                n677 = Concatenate Strings("AO[0]=" ("write buffer"), w1869, "\r\n" ("string")) -> (w1868:string)
                                n678 = call "Serial.vi"("write buffer"=w1868, "VISA resource name"=w1865) -> ()  [unwired: 8 in, 2 out]
                                n679 = case shown="1" w1860 {
                                tunnel: w1859 -> [w1874 w1875]
                                frame 0, Default {
                                "AO[0] 1" <- w1874
                                }
                                frame 1 {
                                "AO[0] 2" <- w1875
                                }
                                }
                                }
                                frame "Wait" {
                                n680 = control-ref of="Motor Speed RPM Serial"() -> (w1898:refnum<vi>)
                                n681 = control-ref of="Pannel User Message"() -> (w1896:refnum<vi>)
                                n682 = control-ref of="Stop Button"() -> (w1897:refnum<vi>)
                                n683 = call "Write panel message Kinetics (SubVI).vi"(4:"rpm"=w1898, 5:"rpm"=TRUE ("rpm"), "PrintTime"=TRUE, "Stop"=w1897, "Time to wait"=20.0, "Strin"="Wait for stabilisation", "String in"=w1896) -> ("RPM"=w1888:dbl, "Stopped"=w1890:bool)  [unwired: 2 in, 1 out]
                                n684 = Or(x=w1890, y=FALSE) -> (x .or. y?=w1891:bool)
                                }
                                frame "Stop" {
                                n685 = case shown="1" w1902 {
                                tunnel: w1903 -> [_ w1916]
                                frame 0, Default {
                                }
                                frame 1 {
                                n686 = property on="AO[0] 2" class="DigNum (strict)"() -> ("Value"=w1908:sgl)  [unwired: 2 in, 2 out]
                                n687 = property on="AO[0] 1" class="DigNum (strict)"() -> ("Value"=w1907:sgl)  [unwired: 2 in, 2 out]
                                n688 = Add(x=w1908, y=w1907) -> (x+y=w1912:sgl)
                                n689 = Divide(x=w1912, y=sgl 2.0) -> (x/y=w1910:sgl)
                                n690 = Number To Fractional String(number=w1910) -> (F-format string=w1909:string)  [unwired: 3 in]
                                n691 = Concatenate Strings("AO[1]=" ("write buffer"), w1909, "\r\n" ("string")) -> (w1915:string)
                                n692 = call "Serial.vi"("write buffer"=w1915, "VISA resource name"=w1916) -> ()  [unwired: 8 in, 2 out]
                                }
                                }
                                }
                              }
                            }
                          }
                        }
                      }
                      frame "Read" {
                        n693 = One Button Dialog(message="No connection.") -> ()  [unwired: 1 in, 1 out]
                      }
                      frame "Init" {
                        w1920 = FALSE ("Analogtest")
                        w1931 = T13 [enum."PowerSuply", enum."Venable"] items=["Init", "0 ohm", "6 ohm", "13.2 ohm", "15 ohm", "25.9 ohm", "33 ohm", "Down", "Up", "Venable", "Firmware", "PowerSuply"]
                        n694 = for {
                          tunnel: w1931 -> [w1938] mode=indexing
                          tunnel: bool[] [TRUE, TRUE] -> [w1937] mode=indexing
                          tunnel: [w1936] -> w1923
                          tunnel: dbl[] [10.0, 2.0] -> [w1934] mode=indexing
                          tunnel: w1928 -> [w1933]
                          n695 = call "Operation (SubVI).vi"("On/Off"=w1937, "Operation"=w1938, "DAQmx Device Name"=w1933) -> ("error out"=w1935:errorcluster)  [unwired: 8 in]
                          n696 = call "Time Delay20"("error in (no error)"=w1935, "Delay Time (s)"=w1934) -> ("error out"=w1936:errorcluster)  [unwired: 9 in]
                        }
                        n697 = for {
                          tunnel: w1924 -> [w1943]
                          tunnel: string[] ["EP=1\r\n", "VC=0\r\n", "CS[0]=0\r\n"] -> [w1942] mode=indexing
                          tunnel: w1923 -> [w1940]
                          tunnel: [w1939] -> w1921
                          n698 = call "Time Delay19"("error in (no error)"=w1940) -> ("error out"=w1941:errorcluster)  [unwired: 10 in]
                          n699 = call "Serial.vi"("error in (no error)"=w1941, "write buffer"=w1942, "VISA resource name"=w1943) -> ("error out"=w1939:errorcluster)  [unwired: 7 in, 1 out]
                        }
                        n700 = Select(t=T11."Read", s=FALSE, f=T11."AO0") -> (s? t:f=w1926:T11)
                        n701 = property on="Analogtest" class="Bool (strict)"(error in=w1921, "Value"=w1920) -> ()  [unwired: 1 in, 2 out]
                      }
                    }
                  }
                }
                n702 = call "Generate AO3"("data"=0.0, "error in"=w1738, "device name"=w1732) -> ("error out"=w1731:errorcluster)  [unwired: 15 in, 1 out]
                n703 = call "Time Delay21"("error in (no error)"=w1731, "Delay Time (s)"=30.0) -> ("error out"=w1730:errorcluster)  [unwired: 9 in]
              }
              frame 1 {
                w1953 = dbl[] [0.0, 1.0, 2.0, 3.0, 4.0, 4.5]
                n704 = for {
                  tunnel: w1953 -> [w1966] mode=indexing
                  tunnel: w1948 -> [w1965]
                  tunnel: w1954 -> [w1964]
                  tunnel: w1947 -> [w1959]
                  tunnel: w1955 -> [w1963]
                  tunnel: w1953 -> [w1962]
                  tunnel: w1949 -> [w1961]
                  tunnel: [w1959] -> w1952
                  shift-right: [w1958] -> _
                  shift-left: T11."Init" -> [w1967]
                  tunnel: [w1957] -> w1950
                  tunnel: w1946 -> [w1956]
                  i -> [w1960]
                  n705 = while {
                    shift-right: [w1973] -> w1958
                    shift-left: w1967 -> [w1979]
                    tunnel: w1966 -> [w1978]
                    tunnel: w1965 -> [w1977]
                    tunnel: w1964 -> [w1976]
                    tunnel: w1963 -> [w1975]
                    tunnel: w1962 -> [w1974]
                    tunnel: w1961 -> [w1972]
                    tunnel: w1960 -> [w1971]
                    tunnel: [w1969] -> w1957
                    tunnel: w1956 -> [w1968]
                    stop <- w1970 stop-if-true
                    n706 = case shown="\"Init\"" w1979 {
                      tunnel: w1978 -> [_ w1984 w2018 w2023 _ _]
                      tunnel: w1977 -> [_ _ _ w2024 _ w2142]
                      tunnel: w1976 -> [_ w1991 _ _ _ w2164]
                      tunnel: w1975 -> [_ w1990 _ _ _ w2163]
                      tunnel: w1974 -> [_ _ _ _ _ w2162]
                      tunnel: [T11."AO0" T11."Exit" T11."Wait" T11."AI0/3" T11."Read" w2146] -> w1973
                      tunnel: [TRUE _ _ w2026 TRUE _] -> w1970
                      tunnel: w1972 -> [_ _ _ w2033 _ _]
                      tunnel: w1971 -> [_ w1985 _ _ _ _]
                      tunnel: [_ _ _ w2026 _ _] -> w1969
                      tunnel: w1968 -> [_ w1983 w2019 _ _ w2149]
                      frame "Exit", Default {
                      }
                      frame "AI0/3" {
                        n707 = Increment(x=w1990) -> (x+1=w1989:i32)
                        n708 = property on="Motor Speed RPM Serial" class="DigNum (strict)"() -> ("Value"=w1993:dbl)  [unwired: 2 in, 2 out]
                        n709 = Multiply(x=w1985, y=2) -> (x*y=w1987:i32)
                        n710 = call "Aquire AI0"("device name"=w1983) -> ("data"=w1994:dynamicdata)  [unwired: 16 in, 2 out]
                        n711 = Add(x=w1989, y=w1987) -> (x+y=w1988:i32)
                        n712 = To Double Precision Float(number=w1994) -> (double precision float=w1982:dbl)
                        n713 = Build Array(w1982, w1993) -> (w1992:dbl[])
                        n714 = for {
                          tunnel: w1992 -> [w1996] mode=indexing
                          tunnel: w1991 -> [w2001]
                          tunnel: w1988 -> [w2003]
                          tunnel: w1985 -> [w1999]
                          tunnel: w1984 -> [w1997]
                          i -> [w2000]
                          n715 = case shown="0, Default" w2000 {
                            tunnel: w1999 -> [_ w2011]
                            tunnel: [w2005 w2014] -> w1998
                            tunnel: w1997 -> [w2007 _]
                            tunnel: w1996 -> [w2004 w2013]
                            frame 0, Default {
                              w2006 = 0.2 ("y")
                              n716 = Add(x=w2006, y=w2007) -> (x+y=w2008:dbl)
                              n717 = Subtract(x=w2007, y=w2006) -> (x-y=w2009:dbl)
                              n718 = In Range and Coerce(upper limit=w2008, x=w2004, lower limit=w2009) -> (In Range?=w2005:bool)  [unwired: 1 out]
                            }
                            frame 1 {
                              w2015 = 200.0 ("y")
                              n719 = property on="SpeedLimit" class="Arr (strict)"() -> ("Value"=w2012:dbl[])  [unwired: 2 in, 2 out]
                              n720 = Index Array(array=w2012, index=w2011) -> (element=w2010:dbl)
                              n721 = Add(x=w2015, y=w2010) -> (x+y=w2016:dbl)
                              n722 = Subtract(x=w2010, y=w2015) -> (x-y=w2017:dbl)
                              n723 = In Range and Coerce(upper limit=w2016, x=w2013, lower limit=w2017) -> (In Range?=w2014:bool)  [unwired: 1 out]
                            }
                          }
                          n724 = Add(x=w2003, y=w2000) -> (x+y=w2002:i32)
                          n725 = call "PassOrFail (SubVI).vi"("index (row)"=w2002, "Data in"=w1996, "Pass?Fail"=w1998, "Table in"=w2001) -> ()  [unwired: 7 in, 1 out]
                        }
                      }
                      frame "AO0" {
                        n726 = call "Generate AO0"("data"=w2018, "device name"=w2019) -> ()  [unwired: 16 in, 2 out]
                      }
                      frame "Wait" {
                        n727 = Equal?(x=w2023, y=4.0) -> ()  [unwired: 1 out]
                        n728 = Number To Fractional String(number=w2023, precision (6)=i16 1) -> (F-format string=w2028:string)  [unwired: 2 in]
                        n729 = Concatenate Strings(w2033, "\r\n", "Analog Output: ", w2028, "V." ("string")) -> (w2027:string)
                        n730 = control-ref of="Motor Speed RPM Serial"() -> (w2034:refnum<vi>)
                        n731 = control-ref of="Pannel User Message"() -> (w2035:refnum<vi>)
                        n732 = control-ref of="Stop Button"() -> (w2039:refnum<vi>)
                        n733 = call "Write panel message Kinetics (SubVI).vi"(4:"rpm"=w2034, 5:"rpm"=TRUE ("rpm"), "PrintTime"=TRUE, "Stop"=w2039, "Time to wait"=20.0, "Strin"=w2027, "String in"=w2035) -> ("error out"=w2025:errorcluster, "Stopped"=w2026:bool)  [unwired: 2 in, 1 out]
                        n734 = case shown="False" FALSE {
                          tunnel: w2025 -> [_ _]
                          tunnel: w2024 -> [_ w2042]
                          frame False {
                          }
                          frame True {
                            n735 = while {
                              shift-right: [w2050] -> _
                              shift-left: "INIT" ("string") -> [w2052]
                              shift-right: [w2049] -> _
                              shift-left: 0.0 ("upper limit") -> [w2048]
                              tunnel: w2042 -> [w2047]
                              shift-right: [w2045] -> _
                              shift-left: 0 -> [w2046]
                              stop <- w2051 stop-if-true
                              n736 = case shown="\"INIT\"" w2052 {
                                selector: w2052 -> [_ _ _ _ w2124]
                                tunnel: [FALSE w2061 FALSE w2103 TRUE] -> w2051
                                tunnel: ["INIT" ("string") w2063 "Wait" ("string") "INIT" ("string") w2124] -> w2050
                                tunnel: [w2056 w2057 w2080 w2100 w2117] -> w2049
                                tunnel: w2048 -> [w2056 _ w2080 _ w2117]
                                tunnel: w2047 -> [_ _ w2079 _ w2115]
                                tunnel: w2046 -> [w2053 w2066 w2078 w2101 w2120]
                                tunnel: [w2053 w2066 w2077 w2101 w2120] -> w2045
                                frame Default {
                                }
                                frame "INIT" {
                                n737 = control-ref of="Motor Speed RPM Serial"() -> (w2058:refnum<vi>)
                                n738 = control-ref of="Pannel User Message"() -> (w2075:refnum<vi>)
                                n739 = control-ref of="Stop Button"() -> (w2071:refnum<vi>)
                                n740 = call "Write panel message Kinetics (SubVI).vi"(4:"rpm"=w2058, 5:"rpm"=TRUE ("rpm"), "PrintTime"=FALSE, "Stop"=w2071, "Time to wait"=0.2, "Strin"="Adjusting AO[0], Please Wait...", "String in"=w2075) -> ("RPM"=w2057:dbl, "Stopped"=w2069:bool)  [unwired: 2 in, 1 out]
                                n741 = In Range and Coerce(upper limit=9650.0, x=w2057, lower limit=9550.0) -> (In Range?=w2059:bool)  [unwired: 1 out]
                                n742 = Equal?(x=w2066, y=3) -> (x = y?=w2060:bool)
                                n743 = Compound Arithmetic op=OR(w2060, w2069, w2059) -> (w2061:bool)
                                n744 = Select(t="Stop" ("string"), s=w2061, f="ADJ" ("string")) -> (s? t:f=w2063:string)
                                }
                                frame "ADJ" {
                                n745 = property on="AO[0]" class="DigNum (strict)"() -> ("Value"=w2085:sgl)  [unwired: 2 in, 2 out]
                                n746 = Less?(x=w2080, y=9550.0) -> (x < y?=w2086:bool)
                                n747 = case shown="True" w2086 {
                                tunnel: w2085 -> [w2094 w2099]
                                tunnel: [w2093 w2097] -> w2081
                                tunnel: w2078 -> [w2091 w2096]
                                tunnel: [w2090 w2095] -> w2077
                                frame False {
                                n748 = Increment(x=w2091) -> (x+1=w2090:i32)
                                n749 = Add(x=w2094, y=sgl 0.01) -> (x+y=w2093:sgl)
                                }
                                frame True {
                                n750 = Increment(x=w2096) -> (x+1=w2095:i32)
                                n751 = Subtract(x=w2099, y=sgl 0.01) -> (x-y=w2097:sgl)
                                }
                                }
                                n752 = Number To Fractional String(number=w2081) -> (F-format string=w2084:string)  [unwired: 3 in]
                                n753 = property on="AO[0]" class="DigNum (strict)"("Value"=w2081) -> ()  [unwired: 2 in, 2 out]
                                n754 = Concatenate Strings("AO[0]=" ("write buffer"), w2084, "\r\n" ("string")) -> (w2083:string)
                                n755 = call "Serial.vi"("write buffer"=w2083, "VISA resource name"=w2079) -> ()  [unwired: 8 in, 2 out]
                                }
                                frame "Wait" {
                                n756 = control-ref of="Motor Speed RPM Serial"() -> (w2110:refnum<vi>)
                                n757 = control-ref of="Pannel User Message"() -> (w2108:refnum<vi>)
                                n758 = control-ref of="Stop Button"() -> (w2109:refnum<vi>)
                                n759 = call "Write panel message Kinetics (SubVI).vi"(4:"rpm"=w2110, 5:"rpm"=TRUE ("rpm"), "PrintTime"=TRUE, "Stop"=w2109, "Time to wait"=7.0, "Strin"="Wait for stabilisation", "String in"=w2108) -> ("RPM"=w2100:dbl, "Stopped"=w2102:bool)  [unwired: 2 in, 1 out]
                                n760 = Or(x=w2102, y=FALSE) -> (x .or. y?=w2103:bool)
                                }
                                frame "Stop" {
                                n761 = property on="AO[0]" class="DigNum (strict)"() -> ("Value"=w2114:sgl)  [unwired: 2 in, 2 out]
                                n762 = In Range and Coerce(upper limit=2450.0, x=w2117, lower limit=2350.0) -> (In Range?=w2116:bool)  [unwired: 1 out]
                                n763 = Equal To 0?(x=w2120) -> (x = 0?=w2119:bool)
                                n764 = Number To Fractional String(number=w2114) -> (F-format string=w2113:string)  [unwired: 3 in]
                                n765 = And(x=w2116, y=w2119) -> (x .and. y?=w2118:bool)
                                n766 = case shown="False" w2118 {
                                tunnel: w2116 -> [w2127 _]
                                tunnel: w2115 -> [w2126 _]
                                tunnel: w2113 -> [w2125 _]
                                frame False {
                                n767 = case shown="True" w2127 {
                                tunnel: w2126 -> [_ w2130]
                                tunnel: w2125 -> [_ w2129]
                                frame False {
                                }
                                frame True {
                                n768 = Concatenate Strings("AO[1]=" ("write buffer"), w2129, "\r\n" ("string")) -> (w2132:string)
                                n769 = call "Serial.vi"("write buffer"=w2132, "VISA resource name"=w2130) -> ()  [unwired: 8 in, 2 out]
                                }
                                }
                                }
                                frame True {
                                }
                                }
                                }
                              }
                            }
                          }
                        }
                      }
                      frame "Read" {
                        n770 = One Button Dialog(message="No connection.") -> ()  [unwired: 1 in, 1 out]
                      }
                      frame "Init" {
                        w2156 = T13 [enum."PowerSuply", enum."Venable"] items=["Init", "0 ohm", "6 ohm", "13.2 ohm", "15 ohm", "25.9 ohm", "33 ohm", "Down", "Up", "Venable", "Firmware", "PowerSuply"]
                        n771 = for {
                          tunnel: w2156 -> [w2171] mode=indexing
                          tunnel: bool[] [TRUE, TRUE] -> [w2170] mode=indexing
                          tunnel: [w2169] -> w2136
                          tunnel: dbl[] [1.0, 1.0] -> [w2167] mode=indexing
                          tunnel: w2149 -> [w2166]
                          n772 = call "Operation (SubVI).vi"("On/Off"=w2170, "Operation"=w2171, "DAQmx Device Name"=w2166) -> ("error out"=w2168:errorcluster)  [unwired: 8 in]
                          n773 = call "Time Delay11"("error in (no error)"=w2168, "Delay Time (s)"=w2167) -> ("error out"=w2169:errorcluster)  [unwired: 9 in]
                        }
                        n774 = call "Aquire AI4"("error in"=w2136, "device name"=w2149) -> ("data"=w2150:dynamicdata, "error out"=w2138:errorcluster)  [unwired: 15 in, 1 out]
                        n775 = call "Serial.vi"("error in (no error)"=w2138, "write buffer"="AG[1]\r\n", "VISA resource name"=w2142) -> ("error out"=w2137:errorcluster, "read buffer"=w2141:string)  [unwired: 7 in]
                        n776 = Fract/Exp String To Number(string=w2141, default (0 dbl)=0.0 ("default (0 DBL)")) -> (number=w2139:dbl)  [unwired: 2 in, 1 out]
                        n777 = Equal To 0?(x=w2139) -> (x = 0?=w2148:bool)
                        n778 = for {
                          tunnel: w2142 -> [w2176]
                          tunnel: [w2172] -> w2158
                          tunnel: string[] ["EP=1\r\n", "VC=0\r\n", "CS[0]=0\r\n", "AG[1]\r\n"] -> [w2175] mode=indexing
                          tunnel: w2137 -> [w2173]
                          n779 = call "Time Delay3"("error in (no error)"=w2173) -> ("error out"=w2174:errorcluster)  [unwired: 10 in]
                          n780 = call "Serial.vi"("error in (no error)"=w2174, "write buffer"=w2175, "VISA resource name"=w2176) -> ("read buffer"=w2172:string)  [unwired: 7 in, 1 out]
                        }
                        n781 = Select(t=T11."Read", s=w2148, f=T11."AO0") -> (s? t:f=w2146:T11)
                        n782 = Fract/Exp String To Number(string=w2158, default (0 dbl)=sgl 0.0 ("default (0 DBL)")) -> (number=w2144:sgl)  [unwired: 2 in, 1 out]
                        n783 = To Double Precision Float(number=w2150) -> (double precision float=→"Offset":dbl)
                        n784 = Add(x=w2163, y=2) -> (x+y=w2161:i32)
                        n785 = for {
                          tunnel: w2164 -> [w2188]
                          tunnel: w2161 -> [w2187]
                          tunnel: w2162 -> [w2183] mode=indexing
                          tunnel: w2144 -> [w2184]
                          tunnel: [w2181] -> w2153
                          tunnel: [w2177] -> w2159 mode=indexing
                          i -> [w2179]
                          n786 = Multiply(x=w2179, y=2) -> (x*y=w2180:i32)
                          n787 = Multiply(x=w2184, y=w2183) -> (x*y=w2177:dbl)
                          n788 = Add(x=w2187, y=w2180) -> (x+y=w2186:i32)
                          n789 = Number To Fractional String(number=w2177, precision (6)=i16 1) -> (F-format string=w2182:string)  [unwired: 2 in]
                          n790 = call "InsertSingleData.vi"("String In"=w2182, "Col"=2, "Row"=w2186, "Table in"=w2188) -> ("error out"=w2181:errorcluster)  [unwired: 7 in]
                        }
                        "SpeedLimit" <- w2159
                        n791 = property on="Analogtest" class="Bool (strict)"(error in=w2153, "Value"=FALSE ("Analogtest")) -> ()  [unwired: 1 in, 2 out]
                      }
                    }
                  }
                }
                n792 = call "Generate AO"("data"=0.0, "error in"=w1952, "device name"=w1946) -> ("error out"=w1945:errorcluster)  [unwired: 15 in, 1 out]
              }
              frame Default {
              }
            }
          }
          n793 = call "Operation (SubVI).vi"("error in (no error)"=w1706, "On/Off"=FALSE, "Operation"=T6."Venable", "DAQmx Device Name"=w1681) -> ()  [unwired: 7 in, 1 out]
        }
        frame "Motor Run Test" {
          n794 = control-ref of="Pannel User Message"() -> (w2223:refnum<vi>)
          n795 = Concatenate Strings(w2205, " in process..." ("Strin")) -> (w2210:string)
          n796 = property class="Str"(reference=w2223, error in=w2220, "Value"=w2210) -> (error out=w2222:errorcluster)  [unwired: 1 out]
          n797 = call "Table_ScrollaBarMarvin.vi"("error in"=w2222, "Line to focus"=w2205, "reference in"=w2213) -> ()  [unwired: 3 out]
          n798 = call "Reset old test Values (SubVI) Kinetics.vi"("Atr in"=w2213, "Test Paragraph"=w2205) -> ("error out"=w2221:errorcluster)  [unwired: 7 in, 2 out]
          n799 = call "Find_Number_LineMARVIN.vi"("Test Paragraph"=w2205, "error in"=w2221, "TableIn"=w2213) -> ("error out"=w2218:errorcluster, "Line number"=w2212:i32)  [unwired: 2 in, 2 out]
          n800 = Increment(x=w2212) -> (x+1=w2211:i32)
          n801 = while {
            tunnel: w2218 -> [w2226]
            tunnel: w2206 -> [w2233]
            shift-right: [w2231] -> _
            shift-left: T12."Init" -> [w2232]
            tunnel: w2213 -> [w2230]
            tunnel: w2211 -> [w2229]
            tunnel: w2210 -> [w2227]
            tunnel: [w2226] -> w2207
            tunnel: [w2224] -> w2204
            i -> [w2228]
            stop <- w2225 stop-if-true
            n802 = case shown="\"ReadCurrent\"" w2232 {
              tunnel: w2226 -> [_ w2239 w2260 w2297 w2306]
              tunnel: w2233 -> [_ _ _ w2298 w2316]
              tunnel: [T12."Exit" T12."ReadTemp" w2257 T12."ReadCurrent" T12."ReadTemp"] -> w2231
              tunnel: w2230 -> [_ _ w2271 w2292 _]
              tunnel: w2229 -> [_ _ w2273 w2294 _]
              tunnel: w2228 -> [_ _ w2274 w2295 _]
              tunnel: w2227 -> [_ w2240 w2259 _ _]
              tunnel: [TRUE ("Stopped") w2237 w2253 _ _] -> w2225
              tunnel: [_ w2237 _ _ _] -> w2224
              frame "Exit", Default {
              }
              frame "Wait" {
                n803 = control-ref of="Motor Speed RPM Serial"() -> (w2245:refnum<vi>)
                n804 = control-ref of="Pannel User Message"() -> (w2244:refnum<vi>)
                n805 = control-ref of="Stop Button"() -> (w2243:refnum<vi>)
                n806 = call "Write panel message Kinetics (SubVI).vi"(4:"rpm"=w2245, 5:"rpm"=TRUE ("rpm"), "PrintTime"=TRUE, "Stop"=w2243, "error in (no error)"=w2239, "Time to wait"=1140.0, "Strin"=w2240, "String in"=w2244) -> ("Stopped"=w2237:bool)  [unwired: 1 in, 2 out]
              }
              frame "ReadCurrent" {
                w2269 = 3.0 ("x")
                n807 = control-ref of="Motor Speed RPM Serial"() -> (w2266:refnum<vi>)
                n808 = control-ref of="Pannel User Message"() -> (w2265:refnum<vi>)
                n809 = control-ref of="Stop Button"() -> (w2264:refnum<vi>)
                n810 = call "Write panel message Kinetics (SubVI).vi"(4:"rpm"=w2266, 5:"rpm"=TRUE ("rpm"), "PrintTime"=TRUE, "Stop"=w2264, "error in (no error)"=w2260, "Time to wait"=59.0, "Strin"=w2259, "String in"=w2265) -> ("error out"=w2256:errorcluster, "Stopped"=w2258:bool)  [unwired: 1 in, 1 out]
                n811 = property on="UUT" class="Str"() -> ("Value"=w2255:string)  [unwired: 2 in, 2 out]
                n812 = case shown="\"True\", Default" w2255 {
                  tunnel: [w2275 w2277] -> w2254
                  tunnel: w2256 -> [_ _]
                  frame "Condenser India", "Condenser Merkava" {
                    n813 = call "Current prob"() -> ("Current"=w2275:dbl)  [unwired: 17 in, 2 out]
                  }
                  frame "True", Default {
                    n814 = local read "CurrentOut"() -> (w2276:dbl)
                    n815 = To Double Precision Float(number=w2276) -> (double precision float=w2277:dbl)
                  }
                }
                n816 = case shown="2, Default" w2274 {
                  tunnel: w2273 -> [w2280 w2283]
                  tunnel: [w2279 w2284] -> w2272
                  tunnel: [T12."Wait" T12."Exit"] -> w2257
                  frame 2, Default {
                    n817 = Increment(x=w2280) -> (x+1=w2279:i32)
                  }
                  frame 5 {
                    n818 = Add(x=w2283, y=3) -> (x+y=w2284:i32)
                  }
                }
                n819 = call "ValFromATR(SubVI).vi"("Row"=w2272, "Table in"=w2271) -> ("Val"=w2270:dbl)  [unwired: 8 in, 1 out]
                n820 = Add(x=w2269, y=w2270) -> (x+y=w2268:dbl)
                n821 = Subtract(x=w2270, y=w2269) -> (x-y=w2267:dbl)
                n822 = local read "DAQmx Device Name"() -> (w2250:tag)
                n823 = In Range and Coerce(upper limit=w2268, x=w2254, lower limit=w2267) -> (In Range?=w2248:bool)  [unwired: 1 out]
                n824 = Not(x=w2248) -> (.not. x?=w2252:bool)
                n825 = Compound Arithmetic op=OR(w2258, w2252) -> (w2253:bool)
                n826 = Not(x=w2248) -> (.not. x?=w2251:bool)
                n827 = call "PassOrFail (SubVI).vi"("index (row)"=w2272, "Data in"=w2254, "Pass?Fail"=w2248, "Table in"=w2271) -> ("error out"=w2246:errorcluster)  [unwired: 7 in]
                n828 = call "Operation (SubVI).vi"("error in (no error)"=w2246, "On/Off"=w2248, "Operation"=T6."PowerSuply", "DAQmx Device Name"=w2250) -> ("error out"=w2247:errorcluster)  [unwired: 7 in]
                n829 = call "Display Message to User7"("error in (no error)"=w2247, "Enable"=w2251) -> ()  [unwired: 8 in, 2 out]
              }
              frame "ReadTemp" {
                w2290 = 15.0 ("x")
                n830 = case shown="4" w2295 {
                  tunnel: w2294 -> [w2300 w2302]
                  tunnel: [w2300 w2303] -> w2293
                  frame 1, Default {
                  }
                  frame 4 {
                    n831 = Add(x=w2302, y=2) -> (x+y=w2303:i32)
                  }
                }
                n832 = call "Serial.vi"("error in (no error)"=w2297, "write buffer"="TA[1]\r\n", "VISA resource name"=w2298) -> ("read buffer"=w2296:string)  [unwired: 7 in, 1 out]
                n833 = call "ValFromATR(SubVI).vi"("Row"=w2293, "Table in"=w2292) -> ("Val"=w2291:dbl)  [unwired: 8 in, 1 out]
                n834 = Fract/Exp String To Number(string=w2296) -> (number=w2286:dbl)  [unwired: 3 in, 1 out]
                n835 = Add(x=w2290, y=w2291) -> (x+y=w2289:dbl)
                n836 = Subtract(x=w2291, y=w2290) -> (x-y=w2288:dbl)
                n837 = In Range and Coerce(upper limit=w2289, x=w2286, lower limit=w2288) -> (In Range?=w2287:bool)  [unwired: 1 out]
                n838 = call "PassOrFail (SubVI).vi"("index (row)"=w2293, "Data in"=w2286, "Pass?Fail"=w2287, "Table in"=w2292) -> ()  [unwired: 7 in, 1 out]
              }
              frame "Init" {
                n839 = local read "DAQmx Device Name"() -> (w2307:tag)
                n840 = call "Operation (SubVI).vi"("error in (no error)"=w2306, "On/Off"=TRUE, "Operation"=T6."PowerSuply", "DAQmx Device Name"=w2307) -> ("error out"=w2305:errorcluster)  [unwired: 7 in]
                n841 = call "Time Delay15"("error in (no error)"=w2305) -> ("error out"=w2304:errorcluster)  [unwired: 10 in]
                n842 = property on="UUT" class="Str"(error in=w2304) -> (error out=w2315:errorcluster, "Value"=w2318:string)  [unwired: 1 in, 1 out]
                n843 = case shown="\"BLDC 60A\"" w2318 {
                  tunnel: ["EP=1\r\nVC=3700\r\n" ("write buffer") "EP=1\r\nVC=9980\r\n" ("write buffer") "EP=1\r\nCL[0]=55\r\nVC=11300\r\n" ("write buffer") "EP=1\r\n" ("write buffer")] -> w2317
                  frame "BLDC 30A", Default {
                  }
                  frame "BLDC 60A" {
                  }
                  frame "Warrior 60A" {
                  }
                  frame "Condenser India", "Condenser Merkava" {
                  }
                }
                n844 = call "Serial.vi"("error in (no error)"=w2315, "write buffer"=w2317, "VISA resource name"=w2316) -> ("error out"=w2310:errorcluster)  [unwired: 7 in, 1 out]
                n845 = local read "DAQmx Device Name"() -> (w2313:tag)
                n846 = call "Operation (SubVI).vi"("error in (no error)"=w2310, "On/Off"=TRUE, "Operation"=T6."Venable", "DAQmx Device Name"=w2313) -> ()  [unwired: 7 in, 1 out]
              }
            }
          }
          n847 = call "Serial.vi"("error in (no error)"=w2207, "write buffer"="EP=1\r\nVC=0\r\n", "VISA resource name"=w2206) -> ("error out"=w2208:errorcluster)  [unwired: 7 in, 1 out]
          n848 = local read "DAQmx Device Name"() -> (w2214:tag)
          n849 = call "Operation (SubVI).vi"("error in (no error)"=w2208, "On/Off"=FALSE, "Operation"=T6."Venable", "DAQmx Device Name"=w2214) -> ()  [unwired: 7 in, 1 out]
        }
        frame "Set Production Parameters" {
          n850 = control-ref of="Pannel User Message"() -> (w2350:refnum<vi>)
          n851 = Concatenate Strings(w2346, " in process..." ("Strin")) -> (w2348:string)
          n852 = property class="Str"(reference=w2350, error in=w2333, "Value"=w2348) -> (error out=w2349:errorcluster)  [unwired: 1 out]
          n853 = call "Table_ScrollaBarMarvin.vi"("error in"=w2349, "Line to focus"=w2346, "reference in"=w2345) -> ("error out"=w2340:errorcluster)  [unwired: 2 out]
          n854 = call "Reset old test Values (SubVI) Kinetics.vi"("error in"=w2340, "Atr in"=w2345, "Test Paragraph"=w2346) -> ("error out"=w2341:errorcluster)  [unwired: 6 in, 2 out]
          n855 = call "Find_Number_LineMARVIN.vi"("Test Paragraph"=w2346, "error in"=w2341, "TableIn"=w2345) -> ("error out"=w2330:errorcluster, "Line number"=w2338:i32)  [unwired: 2 in, 2 out]
          n856 = local read "DAQmx Device Name"() -> (w2336:tag)
          n857 = call "Operation (SubVI).vi"("error in (no error)"=w2330, "On/Off"=TRUE, "Operation"=T6."PowerSuply", "DAQmx Device Name"=w2336) -> ("error out"=w2329:errorcluster)  [unwired: 7 in]
          n858 = call "Time Delay16"("error in (no error)"=w2329) -> ("error out"=w2328:errorcluster)  [unwired: 10 in]
          n859 = property on="Automation" class="Bool (strict)"(error in=w2328) -> (error out=w2326:errorcluster, "Value"=w2323:bool)  [unwired: 1 in, 1 out]
          n860 = case shown="True" w2323 {
            tunnel: w2332 -> [_ w2356]
            tunnel: w2331 -> [_ w2355]
            tunnel: [w2352 w2354] -> w2327
            tunnel: w2326 -> [w2352 _]
            frame False {
            }
            frame True {
              n861 = property on="Current SN" class="DigNum (strict)"() -> (error out=w2362:errorcluster, "Value"=w2369:i32)  [unwired: 2 in, 1 out]
              n862 = Equal To 0?(x=w2369) -> (x = 0?=w2367:bool)
              n863 = Equal?(x=w2369, y=-1) -> (x = y?=w2368:bool)
              n864 = property on="UUT" class="Str"() -> ("Value"=w2361:string)  [unwired: 2 in, 2 out]
              n865 = Or(x=w2368, y=w2367) -> (x .or. y?=w2366:bool)
              n866 = control-ref of="ATR"() -> (w2363:refnum<vi>)
              n867 = case shown="\"BLDC 60A\"" w2361 {
                tunnel: [37 37 12 12 45] -> w2359
                frame "BLDC 30A", Default {
                }
                frame "Warrior 60A" {
                }
                frame "Condenser Merkava" {
                }
                frame "Condenser India" {
                }
                frame "BLDC 60A" {
                }
              }
              n868 = call "PassFailUUT (SubVI).vi"("error in (no error)"=w2362, "Table in"=w2363) -> ("Total Pass"=w2360:i32)  [unwired: 7 in, 2 out]
              n869 = Equal?(x=w2360, y=w2359) -> (x = y?=w2358:bool)
              n870 = property on="CAN Status" class="Bool (strict)"() -> ("Value"=w2364:bool)  [unwired: 2 in, 2 out]
              n871 = property on="Serial Status" class="Bool (strict)"() -> ("Value"=w2365:bool)  [unwired: 2 in, 2 out]
              n872 = And(x=w2365, y=w2364) -> (x .and. y?=w2353:bool)
              n873 = case shown="True" w2353 {
                tunnel: w2356 -> [_ w2382]
                tunnel: w2366 -> [_ w2378]
                tunnel: w2355 -> [_ w2381]
                tunnel: [errorcluster {"status"=FALSE, "code"=0, "source"=""} ("error out") w2380] -> w2354
                tunnel: w2358 -> [_ w2379]
                frame False {
                  n874 = call "Display Message to User4"() -> ()  [unwired: 10 in, 2 out]
                  n875 = property on="SetSN" class="Bool (strict)"("Value"=FALSE) -> ()  [unwired: 2 in, 2 out]
                }
                frame True {
                  n876 = And(x=w2378, y=w2379) -> (x .and. y?=w2377:bool)
                  n877 = case shown="True" w2377 {
                    tunnel: w2382 -> [_ w2394]
                    tunnel: w2381 -> [_ w2393]
                    tunnel: [w2384 w2392] -> w2380
                    tunnel: w2378 -> [w2383 _]
                    frame False {
                      n878 = case shown="True" w2383 {
                        tunnel: [w2385 w2386] -> w2384
                        frame False {
                          n879 = call "Display Message to User6"() -> ("error out"=w2385:errorcluster)  [unwired: 10 in, 1 out]
                        }
                        frame True {
                          n880 = call "Display Message to User8"() -> ("error out"=w2386:errorcluster)  [unwired: 10 in, 1 out]
                        }
                      }
                    }
                    frame True {
                      n881 = control-ref of="Current SN"() -> (w2389:refnum<vi>)
                      n882 = control-ref of="UUT"() -> (w2388:refnum<vi>)
                      n883 = local read "DAQmx Device Name"() -> (w2391:tag)
                      n884 = control-ref of="Next SN"() -> (w2390:refnum<vi>)
                      n885 = call "SetSN (SubVI).vi"("Kinetics Params"=w2394, "UUT"=w2388, "DAQmx Device Name"=w2391, "Current SN"=w2389, "VISA resource name"=w2393, "Next SN"=w2390) -> ("error out"=w2392:errorcluster, "UUT SN Report"=w2387:string)  [unwired: 4 in]
                      n886 = property on="UUT SN Report" class="Str"("Value"=w2387) -> ()  [unwired: 2 in, 2 out]
                    }
                  }
                }
              }
            }
          }
          n887 = Increment(x=w2338) -> (x+1=w2337:i32)
          n888 = for {
            tunnel: w2331 -> [w2403]
            tunnel: w2345 -> [w2402]
            tunnel: w2327 -> [w2401]
            tunnel: string[] ["SN\r\n"] -> [w2400] mode=indexing
            tunnel: w2337 -> [w2397]
            tunnel: [w2395] -> w2343
            i -> [w2398]
            n889 = call "Serial.vi"("error in (no error)"=w2401, "write buffer"=w2400, "VISA resource name"=w2403) -> ("error out"=w2395:errorcluster, "read buffer"=w2399:string)  [unwired: 7 in]
            n890 = Add(x=w2397, y=w2398) -> (x+y=w2396:i32)
            n891 = case shown="0, Default" w2398 {
              tunnel: w2402 -> [w2411 w2418]
              tunnel: w2395 -> [w2410 w2417]
              tunnel: w2399 -> [w2405 w2413]
              tunnel: w2396 -> [w2406 w2412]
              frame 0, Default {
                n892 = property on="Current SN" class="DigNum (strict)"() -> ("Value"=w2404:i32)  [unwired: 2 in, 2 out]
                n893 = Number To Decimal String(number=w2404) -> (decimal integer string=w2409:string)  [unwired: 1 in]
                n894 = Equal?(x=w2405, y=w2409) -> (x = y?=w2408:bool)
                n895 = call "PassOrFail (SubVI).vi"("String Res"=w2405, "index (row)"=w2406, "error in (no error)"=w2410, "Data in"=-3.0, "Pass?Fail"=w2408, "Table in"=w2411) -> ()  [unwired: 5 in, 1 out]
              }
              frame 1 {
                n896 = property on="PN" class="Str"() -> ("Value"=w2416:string)  [unwired: 2 in, 2 out]
                n897 = Equal?(x=w2416, y=w2413) -> (x = y?=w2415:bool)
                n898 = call "PassOrFail (SubVI).vi"("String Res"=w2413, "index (row)"=w2412, "error in (no error)"=w2417, "Data in"=-3.0, "Pass?Fail"=w2415, "Table in"=w2418) -> ()  [unwired: 5 in, 1 out]
              }
            }
          }
          n899 = disable-structure shown="Disabled" {
            frame Disabled {
              n900 = property on="SN From File" class="Str" props=["Value"]() -> ()  [unwired: 2 in, 3 out]
            }
            frame Enabled {
            }
          }
          n901 = property on="Pannel User Message" class="Str"(error in=w2343, "Value"="You can press start to execute(s) test(s)." ("Pannel User Message")) -> (error out=w2324:errorcluster)  [unwired: 1 in, 1 out]
          n902 = property on="Automation" class="Bool (strict)"(error in=w2324) -> ("Value"=w2325:bool)  [unwired: 1 in, 2 out]
          n903 = case shown="True" w2325 {
            frame False {
            }
            frame True {
              w2351 = TRUE ("Value (Signaling)")
              n904 = property on="Report" class="Bool (strict)"("Val(Sgnl)"=w2351, "Value"=w2351) -> ()  [unwired: 2 in, 2 out]
            }
          }
        }
        frame "Visual Inspection" {
          n905 = property on="UUT In" class="Ring (strict)"(error in=w2425) -> ("Value"=w2419:u16)  [unwired: 1 in, 2 out]
          n906 = case shown="4, 5" w2419 {
            tunnel: [string[][] [["J56 to CHASIS", "< 2m", "-", "ohms", "", ""], ["J57 to CHASIS", "< 2m", "-", "ohms", "", ""], ["J58 to CHASIS", "< 2m", "-", "ohms", "", ""], ["J56_A to CHASIS", "> 500k", "-", "ohms", "", ""], ["J56_B to CHASIS", "> 500k", "-", "ohms", "", ""], ["J56_C to CHASIS", "> 500k", "-", "ohms", "", ""], ["J57_A to CHASIS", "> 500k", "-", "ohms", "", ""], ["J57_B to CHASIS", "> 500k", "-", "ohms", "", ""], ["Torque wrench by DIN Standard & ", "-", "-", ".", "", ""], ["manufacturer's instructions for nut Torque.", "-", "-", ".", "", ""], ["Motor Speed ", "9980", "+/-100", "rpm", "", ""], ["Driver Current ", "47", "+/-3", "A", "", ""], ["Leak Test", "", "", "", "", ""]] ("deleted portion") string[][] [["J56 to CHASIS", "< 2m", "-", "ohms", "", ""], ["J57 to CHASIS", "< 2m", "-", "ohms", "", ""], ["J58 to CHASIS", "< 2m", "-", "ohms", "", ""], ["J56_A to CHASIS", "> 500k", "-", "ohms", "", ""], ["J56_B to CHASIS", "> 500k", "-", "ohms", "", ""], ["J56_C to CHASIS", "> 500k", "-", "ohms", "", ""], ["J57_A to CHASIS", "> 500k", "-", "ohms", "", ""], ["J57_B to CHASIS", "> 500k", "-", "ohms", "", ""], ["Torque wrench by DIN Standard & ", "-", "-", ".", "", ""], ["manufacturer's instructions for nut Torque.", "-", "-", ".", "", ""], ["Motor Speed ", "3700", "+/-100", "rpm", "", ""], ["Driver Current ", "27", "+/-3", "A", "", ""], ["Leak Test", "", "", "", "", ""]] ("deleted portion") string[][] [["Motor Speed ", "8000", "+/-100", "rpm", "", ""], ["Driver Current ", "50", "+/-3", "A", "", ""], ["Leak Test", "", "", "", "", ""]] ("deleted portion 2") string[][] [] ("deleted portion 2")] -> w2424
            frame 1 {
            }
            frame 2, 3 {
              # "Namer 30 & Warior"
            }
            frame 4, 5 {
              # "Condenser"
            }
            frame Default {
            }
          }
          n907 = Index Array(array=w2424, index (col)=0 ("disabled index (col)")) -> (element=w2422:string[])  [unwired: 1 in]
          n908 = for {
            tunnel: w2421 -> [w2429]
            tunnel: w2425 -> [w2428]
            tunnel: w2422 -> [w2427] mode=indexing
            tunnel: [w2426] -> w2420
            n909 = call "Reset old test Values (SubVI) Kinetics.vi"("error in"=w2428, "Atr in"=w2429, "Test Paragraph"=w2427) -> ("error out"=w2426:errorcluster)  [unwired: 6 in, 2 out]
          }
          n910 = call "VisualInspectionKineticsNamer60.vi"("error in (no error)"=w2420, "PN"=w2419, "SubTestName"=w2422, "TableRef"=w2421) -> ()  [unwired: 6 in, 2 out]
        }
      }
      "TestinExecution" <- w244
    }
    n911 = flat-sequence {
      tunnel: w228 -> [_]
      frame #0 {
        w238 = T1."Enabled" ("Disabled")
        w239 = FALSE ("Start")
        n912 = local read "DAQmx Device Name"() -> (w237:tag)
        n913 = property on="Start" class="Bool (strict)"("Value"=w239, "DisabledEnum"=w238) -> ()  [unwired: 2 in, 2 out]
        n914 = property on="Report" class="Bool (strict)"("Value"=w239, "DisabledEnum"=w238) -> ()  [unwired: 2 in, 2 out]
        n915 = call "Operation (SubVI).vi"("On/Off"=FALSE, "Operation"=T6."PowerSuply", "DAQmx Device Name"=w237) -> ()  [unwired: 8 in, 1 out]
      }
    }
    n916 = property on="G.Stop" class="Bool (strict)"() -> ("Value"=w225:bool)  [unwired: 2 in, 2 out]
    n917 = Or(x=w225, y=w229) -> (x .or. y?=w226:bool)
  }
  n918 = while {
    shift-right: [w2439] -> _
    shift-left: T4."Initialize" -> [w2457]
    shift-right: [w2454] -> _
    shift-left: _ -> [w2453]
    shift-right: [w2452] -> _
    shift-left: w34 -> [w2450]
    shift-right: [w2451] -> _
    shift-left: refnum<vi> refnum ("Config_CANAT") -> [w2449]
    shift-right: [w2447] -> _
    shift-left: w31 -> [w2448]
    tunnel: "ATR" -> [_]
    tunnel: w25 -> [w2446]
    tunnel: w24 -> [w2445]
    shift-right: [w2443] -> _
    shift-left: w9 -> [w2444]
    tunnel: w6 -> [w2442]
    tunnel: w10 -> [w2441]
    tunnel: w23 -> [_]
    tunnel: w32 -> [w2456]
    tunnel: [w2455] -> _
    tunnel: w16 -> [_]
    tunnel: w14 -> [w2440]
    shift-right: [w2437] -> _
    shift-left: w9 -> [w2438]
    shift-right: [w2435] -> _
    shift-left: w9 -> [w2436]
    tunnel: [w2434] -> w7
    tunnel: w5 -> [_]
    stop <- w2434 stop-if-true
    n919 = case shown="\"Erase ATR Table\", Default" w2457 {
      tunnel: [T4."MainProgram" w2654 w2717 w3278] -> w2439
      tunnel: [FALSE w2642 FALSE FALSE] -> w2434
      tunnel: [w2459 w2647 w2711 w3271] -> w2455
      tunnel: w2456 -> [_ w2612 w2715 _]
      tunnel: [w2470 refnum<visa-resource-name> refnum ("VISA resource name") w2712 w3276] -> w2454
      tunnel: w2453 -> [_ w2666 w2713 _]
      tunnel: [w2517 w2636 w2707 w3296] -> w2452
      tunnel: [w2505 refnum<vi> refnum ("Config_CANAT") w2708 w3286] -> w2451
      tunnel: w2450 -> [w2517 w2668 w2710 w3296]
      tunnel: w2449 -> [_ w2657 w2709 w3286]
      tunnel: w2448 -> [w2516 w2661 w2706 w3295]
      tunnel: [w2516 w2635 w2705 w3295] -> w2447
      tunnel: w2446 -> [_ _ w2704 _]
      tunnel: w2445 -> [_ _ w2703 _]
      tunnel: w2444 -> [w2515 w2659 w2702 w3293]
      tunnel: [w2515 w2659 w2701 w3293] -> w2443
      tunnel: w2442 -> [w2514 _ w2700 _]
      tunnel: w2441 -> [_ _ w2699 _]
      tunnel: w2440 -> [_ _ w2698 _]
      tunnel: w2438 -> [_ _ w2697 _]
      tunnel: [w2512 w2634 w2696 w3288] -> w2437
      tunnel: w2436 -> [_ _ w2695 _]
      tunnel: [w2512 w2634 w2694 w3288] -> w2435
      frame "Erase ATR Table", Default {
        w2463 = u16 1 items=["BLDC 60A"=1, "BLDC 30A"=2, "Warrior 60A"=3, "Condenser Merkava"=4, "Condenser India"=5] ("UUT")
        w2465 = FALSE ("STDBY")
        w2504 = refnum<visa-resource-name> "COMx" ("VISA Kinetics")
        w2512 = 0
        w2458 = T1."Enabled" ("Disabled")
        w2519 = FALSE ("Visible")
        n920 = property on="Serial Com" class="Bool"(error in=errorcluster {"status"=FALSE, "code"=0, "source"=""} ("error out"), "Visible"=FALSE) -> (error out=w2466:errorcluster)  [unwired: 1 in, 1 out]
        n921 = property on="STDBY" class="Bool (strict)"(error in=w2466, "Value"=w2465, "Blinking"=w2465) -> ()  [unwired: 1 in, 2 out]
        n922 = property on="VISA Kinetics" class="VISAName"(error in=w2466, "Visible"=w2519, "Value"=w2504) -> (error out=w2521:errorcluster)  [unwired: 1 in, 1 out]
        n923 = property on="Serial Status" class="Bool (strict)"(error in=w2521, "Value"=w2519) -> (error out=w2510:errorcluster)  [unwired: 1 in, 1 out]
        n924 = property on="Pannel User Message" class="Str"(error in=w2510, "Value"="Select a UUT from list bellow:") -> (error out=w2509:errorcluster)  [unwired: 1 in, 1 out]
        n925 = call "UUT select.vi"("error constant"=w2509, "UUT"=w2463) -> ("error constant 2"=w2491:errorcluster, 2:"UUT Out"=w2469:string, 3:"UUT Out"=w2464:u16)  [unwired: 7 in]
        "UUT" <- w2469
        "UUT In" <- w2464
        n926 = property on="Pannel User Message" class="Str"(error in=w2491, "Value"="Tester initialization in process..." ("Pannel User Message")) -> (error out=w2490:errorcluster)  [unwired: 1 in, 1 out]
        n927 = call "ATRBuild.vi"("error constant"=w2490, "UUT In"=w2464) -> ("error constant 2"=w2508:errorcluster, "TestArray"=→"TestArray":string[], "TestArray Out"=w2507:string[][])  [unwired: 7 in]
        n928 = for {
          tunnel: w2507 -> [w2601] mode=indexing
          tunnel: w2508 -> [w2599]
          tunnel: [w2598] -> w2513
          tunnel: w2507 -> [w2597]
          i -> [w2600]
          n929 = for {
            tunnel: w2601 -> [_] mode=indexing
            tunnel: w2600 -> [w2607]
            tunnel: w2599 -> [w2604]
            tunnel: [w2603] -> w2598
            tunnel: w2597 -> [w2602]
            i -> [w2608]
            n930 = Bundle By Name(cluster=T14 {"Row"=0, "Column"=0} ("Active Cell:Active Cell"), "Row"=w2607, "Column"=w2608) -> (w2606:T14)
            n931 = control-ref of="ATR"() -> (w2605:refnum<vi>)
            n932 = property class="Tbl (strict)"(reference=w2605, error in=w2604, "Active Cell"=w2606, "Cell BG Color"=u32 16777226, "Value"=w2602) -> (error out=w2603:errorcluster)  [unwired: 1 out]
          }
        }
        n933 = call "DataFrom_ini (SubVI).vi"("appended path"=w2514, "UUT"=w2469, "error in (no error)"=w2513) -> ("ProductRev"=→"ProductRev":string, "PN"=w2460:string, "ParamVersion"=→"ParamVersion":string, "UUT SoftwareVer"=w2461:string, "Next SN"=w2483:i32, "FileName"=w2500:string, "error out"=w2475:errorcluster)  [unwired: 10 in]
        "UUT SoftwareVer" <- w2461
        "Next SN" <- w2483
        "FileName" <- w2500
        "PN" <- w2460
        n934 = Number To Decimal String(number=w2483) -> (decimal integer string=w2482:string)  [unwired: 1 in]
        "SN From File" <- w2482
        n935 = control-ref of="ATR"() -> (w2496:refnum<vi>)
        n936 = Build Array(w2461, w2461, w2482) -> (w2481:string[])
        n937 = call "Boards S/N"("error in (no error)"=w2475) -> ("POWER Board S/N"=→"POWER Board S/N":string, "DSP Board S/N"=→"DSP Board S/N":string, "error out"=w2474:errorcluster)  [unwired: 15 in, 1 out]
        n938 = for {
          tunnel: w2474 -> [w2536]
          tunnel: w2496 -> [w2534]
          tunnel: string[] ["RS232 Comm. + Version", "CAN Comm.", "Unit Serial number"] -> [w2533] mode=indexing
          tunnel: [w2532] -> w2498
          tunnel: [w2531] -> w2480 mode=indexing
          tunnel: w2481 -> [w2530] mode=indexing
          n939 = call "Find_Number_LineMARVIN.vi"("Test Paragraph"=w2533, "error in"=w2536, "TableIn"=w2534) -> ("error out"=w2535:errorcluster, "Line number"=w2531:i32)  [unwired: 2 in, 2 out]
          n940 = call "InsertSingleData.vi"("String In"=w2530, "error in (no error)"=w2535, "Col"=2, "Row"=w2531, "Table in"=w2534) -> ("error out"=w2532:errorcluster)  [unwired: 6 in]
        }
        n941 = control-ref of="This VI"() -> (w2494:refnum<vi>)
        n942 = Index Array(array=w2480, index=1) -> (element=w2478:i32)
        n943 = call "COM UUT Board.vi"("error in (no error)"=w2498, "VI reference (current VI)"=w2494, "VISA resource name 2"=w2504) -> ("error out"=w2502:errorcluster, ".not. x?"=w2488:bool, "VISA resource name out"=w2501:refnum<visa-resource-name>)  [unwired: 6 in]
        "Serial Status" <- w2488
        n944 = case shown="True" w2488 {
          tunnel: w2502 -> [w2538 w2572]
          tunnel: w2501 -> [w2539 w2571]
          tunnel: [w2539 w2540] -> w2470
          tunnel: [w2538 w2562] -> w2472
          tunnel: w2500 -> [_ w2561]
          tunnel: w2461 -> [_ w2557]
          tunnel: w2460 -> [_ w2548]
          frame False {
          }
          frame True {
            n945 = local read "DAQmx Device Name"() -> (w2552:tag)
            n946 = control-ref of="Motor Speed RPM Serial"() -> (w2549:refnum<vi>)
            n947 = VISA Flush I/O Buffer(VISA resource name=w2571, error in (no error)=w2572) -> (VISA resource name out=w2540:refnum<visa-resource-name>, error out=w2570:errorcluster)  [unwired: 1 in]
            n948 = control-ref of="Stop Button"() -> (w2551:refnum<vi>)
            n949 = control-ref of="Pannel User Message"() -> (w2550:refnum<vi>)
            n950 = call "SetParameters (SubVI).vi"("Stop"=w2551, "Pannel User Message"=w2550, "DAQmx Device Name"=w2552, "VISA resource name in"=w2540, "PN"=w2548, "Motor Speed RPM Serial"=w2549, "error in (no error)"=w2570, "FileName"=w2561) -> ("CC=1"=w2546:dbl, 6:"CC=2"=w2545:string, 8:"CC=2"=w2544:string, "SetParam?"=w2547:bool, "error out"=w2569:errorcluster)  [unwired: 3 in]
            n951 = case shown="False" w2547 {
              tunnel: w2546 -> [_ w2587]
              tunnel: w2545 -> [_ w2586]
              tunnel: w2544 -> [_ w2585]
              tunnel: [w2582 w2587] -> w2541
              tunnel: [w2578 w2586] -> w2542
              tunnel: [w2577 w2585] -> w2543
              tunnel: w2540 -> [w2579 _]
              frame False {
                n952 = call "Serial.vi"("write buffer"="CC\r\n", "VISA resource name"=w2579) -> ("error out"=w2576:errorcluster, "read buffer"=w2583:string)  [unwired: 8 in]
                n953 = call "Time Delay12"("error in (no error)"=w2576) -> ("error out"=w2575:errorcluster)  [unwired: 10 in]
                n954 = call "Serial.vi"("error in (no error)"=w2575, "write buffer"="AO[1]\r\n", "VISA resource name"=w2579) -> ("error out"=w2574:errorcluster, "read buffer"=w2578:string)  [unwired: 7 in]
                n955 = call "Time Delay17"("error in (no error)"=w2574) -> ("error out"=w2573:errorcluster)  [unwired: 10 in]
                n956 = Fract/Exp String To Number(string=w2583) -> (number=w2582:dbl)  [unwired: 3 in, 1 out]
                n957 = call "Serial.vi"("error in (no error)"=w2573, "write buffer"="RO[1]\r\n", "VISA resource name"=w2579) -> ("read buffer"=w2577:string)  [unwired: 7 in, 1 out]
              }
              frame True {
              }
            }
            "CC" <- w2541
            "AO[1]" <- w2542
            "RO[1]" <- w2543
            n958 = call "Serial.vi"("error in (no error)"=w2569, "write buffer"="SN\r\n", "VISA resource name"=w2540) -> ("error out"=w2566:errorcluster, "read buffer"=w2555:string)  [unwired: 7 in]
            n959 = property on="UUT SN Report" class="Str"("Value"=w2555) -> ()  [unwired: 2 in, 2 out]
            n960 = Decimal String To Number(string=w2555) -> (number=w2553:i32)  [unwired: 2 in, 1 out]
            "Current SN" <- w2553
            n961 = call "Serial.vi"("error in (no error)"=w2566, "write buffer"="VR\r\n", "VISA resource name"=w2540) -> ("error out"=w2556:errorcluster, "read buffer"=w2558:string)  [unwired: 7 in]
            n962 = case shown="1, Default" w2553 {
              tunnel: w2556 -> [w2588 w2596]
              tunnel: w2555 -> [_ w2590]
              tunnel: [w2588 w2589] -> w2554
              frame -1, 0 {
              }
              frame 1, Default {
                n963 = control-ref of="ATR"() -> (w2592:refnum<vi>)
                n964 = call "Find_Number_LineMARVIN.vi"("Test Paragraph"="Unit Serial number", "error in"=w2596, "TableIn"=w2592) -> ("error out"=w2591:errorcluster, "Line number"=w2594:i32)  [unwired: 2 in, 2 out]
                n965 = call "InsertSingleData.vi"("String In"=w2590, "error in (no error)"=w2591, "Col"=2, "Row"=w2594, "Table in"=w2592) -> ("error out"=w2589:errorcluster)  [unwired: 6 in]
              }
            }
            n966 = control-ref of="ATR"() -> (w2563:refnum<vi>)
            n967 = call "Find_Number_LineMARVIN.vi"("Test Paragraph"="RS232 Comm. + Version", "error in"=w2554, "TableIn"=w2563) -> ("Line number"=w2564:i32)  [unwired: 2 in, 3 out]
            n968 = Equal?(x=w2558, y=w2557) -> (x = y?=w2559:bool)
            n969 = call "PassOrFail (SubVI).vi"("String Res"=w2558, "index (row)"=w2564, "Data in"=-3.0, "Pass?Fail"=w2559, "Table in"=w2563) -> ("error out"=w2562:errorcluster)  [unwired: 6 in]
          }
        }
        n970 = case shown="\"Condenser India\", \"Condenser Merkava\"" w2469 {
          tunnel: w2472 -> [w2525 w2528]
          tunnel: [w2525 w2527] -> w2471
          tunnel: w2470 -> [_ w2526]
          frame "False", Default {
          }
          frame "Condenser India", "Condenser Merkava" {
            n971 = call "Serial.vi"("error in (no error)"=w2528, "write buffer"="EP=1\r\nVC=1000\r\n", "VISA resource name"=w2526) -> ("error out"=w2527:errorcluster)  [unwired: 7 in, 1 out]
          }
        }
        n972 = call "KineticsCan.vi"("error in"=w2471) -> ("error out"=w2497:errorcluster, "Version"=w2492:string, "Res_Pass_T"=w2468:bool, "Config_CANAT_out"=w2505:refnum<vi>)  [unwired: 7 in]
        n973 = case shown="\"False\", Default" w2469 {
          tunnel: w2468 -> [w2523 _]
          tunnel: [w2523 TRUE ("Res_Pass_T")] -> w2467
          frame "False", Default {
          }
          frame "Condenser India", "Condenser Merkava" {
          }
        }
        "CAN Status" <- w2467
        n974 = Equal?(x=w2492, y=w2461) -> (x = y?=w2493:bool)
        n975 = call "PassOrFail (SubVI).vi"("String Res"=w2492, "index (row)"=w2478, "error in (no error)"=w2497, "Data in"=-3.0, "Pass?Fail"=w2493, "Table in"=w2496) -> ("error out"=w2487:errorcluster)  [unwired: 5 in]
        n976 = property on="Pannel User Message" class="Str"(error in=w2487, "Value"="You can press start to execute(s) test(s)." ("Pannel User Message")) -> (error out=w2486:errorcluster)  [unwired: 1 in, 1 out]
        n977 = property on="Start" class="Bool (strict)"(error in=w2486, "DisabledEnum"=w2458) -> (error out=w2503:errorcluster)  [unwired: 1 in, 1 out]
        n978 = property on="Report" class="Bool (strict)"(error in=w2503, "DisabledEnum"=w2458) -> (error out=w2459:errorcluster)  [unwired: 1 in, 1 out]
        n979 = property on="Stop Button" class="Bool (strict)"(error in=w2459, "DisabledEnum"=w2458) -> ()  [unwired: 1 in, 2 out]
      }
      frame "Stop" {
        w2611 = FALSE ("STDBY")
        w2634 = 0
        n980 = property on="STDBY" class="Bool (strict)"(error in=w2612, "Value"=w2611, "Blinking"=w2611) -> ()  [unwired: 1 in, 2 out]
        n981 = control-ref of="ATR"() -> (w2633:refnum<vi>)
        n982 = call "PassFailUUT (SubVI).vi"("error in (no error)"=w2612, "Table in"=w2633) -> ("PassFaileUUTresult"=w2626:bool)  [unwired: 7 in, 2 out]
        n983 = property on="Test Failed" class="Bool (strict)"("Value"=w2626) -> ()  [unwired: 2 in, 2 out]
        n984 = flat-sequence {
          tunnel: w2612 -> [w2691]
          tunnel: [w2690] -> w2658
          frame #0 {
            n985 = control-ref of="Pannel User Message"() -> (w2693:refnum<vi>)
            n986 = property class="Str"(reference=w2693, error in=w2691, "Value"="Program Stopped...\r\nPlease turn OFF All Power sinks") -> (error out=w2690:errorcluster)  [unwired: 1 out]
          }
        }
        n987 = Select(t="PASS" ("name or relative path"), s=w2626, f="FAIL" ("name or relative path")) -> (s? t:f=w2625:string)
        n988 = call <vilib>:"Application Directory.vi"() -> ("Application Directory"=w2629:path)
        n989 = Build Path(base path=w2629, name or relative path="data\\TestResult.ini") -> (appended path=w2632:path)
        n990 = call <vilib>:"Open Config Data.vi"("configuration file path"=w2632) -> ("error out"=w2630:errorcluster, "refnum"=w2631:T5)  [unwired: 2 in, 7 out]
        n991 = call-poly <vilib>:"Write Key.vi"("section"="Kinetics", "error in (no error)"=w2630, "value"=w2625, "key"="Result", "refnum"=w2631) -> ("error out"=w2628:errorcluster, "refnum out"=w2627:T5)  [unwired: 4 in, 1 out]
        n992 = call <vilib>:"Close Config Data.vi"("error in (no error)"=w2628, "refnum"=w2627) -> ()  [unwired: 8 in, 2 out]
        n993 = property on="VISA Current" class="VISAName"() -> ("Value"=w2615:refnum<visa-resource-name>)  [unwired: 2 in, 2 out]
        n994 = local read "DAQmx Device Name"() -> (w2619:tag)
        n995 = call "Clear CAN Buffer.vi"("error in (no error)"=w2658, "Cluster in"=w2657) -> ("error out"=w2613:errorcluster)  [unwired: 8 in, 1 out]
        n996 = call "Close CAN Device.vi"("error in (no error)"=w2613, "Cluster in"=w2657) -> ("error out"=w2646:errorcluster)  [unwired: 8 in, 1 out]
        n997 = VISA Close(VISA resource name=w2666, error in (no error)=w2658) -> (error out=w2660:errorcluster)
        n998 = VISA Close(VISA resource name=w2615) -> (error out=w2614:errorcluster)  [unwired: 1 in]
        n999 = property on="Stop Button" class="Bool (strict)"() -> ("Value"=w2638:bool)  [unwired: 2 in, 2 out]
        n1000 = call "Operation (SubVI).vi"("On/Off"=FALSE, "Operation"=T6."Init", "DAQmx Device Name"=w2619) -> ("error out"=w2616:errorcluster)  [unwired: 8 in]
        n1001 = property on="ClosePanel" class="Bool (strict)"() -> ("Value"=w2639:bool)  [unwired: 2 in, 2 out]
        n1002 = Or(x=w2639, y=w2638) -> (x .or. y?=w2637:bool)
        n1003 = Flush Queue(queue=w2661, error in (no error)=w2660) -> (queue out=w2663:refnum<queue>, error out=w2662:errorcluster)  [unwired: 1 out]
        n1004 = Flush Queue(queue=w2668, error in (no error)=w2660) -> (queue out=w2667:refnum<queue>, error out=w2669:errorcluster)  [unwired: 1 out]
        n1005 = case shown="True" w2637 {
          tunnel: w2669 -> [w2671 w2679]
          tunnel: w2667 -> [w2673 w2675]
          tunnel: w2663 -> [w2672 w2674]
          tunnel: w2662 -> [w2670 w2678]
          tunnel: [w2671 w2677] -> w2653
          tunnel: [w2670 w2676] -> w2652
          tunnel: [w2673 w2675] -> w2636
          tunnel: [w2672 w2674] -> w2635
          frame False {
          }
          frame True {
            n1006 = Release Queue(queue=w2674, error in (no error)=w2678) -> (error out=w2676:errorcluster)  [unwired: 1 in, 2 out]
            n1007 = Release Queue(queue=w2675, error in (no error)=w2679) -> (error out=w2677:errorcluster)  [unwired: 1 in, 2 out]
          }
        }
        n1008 = Merge Errors(w2653, w2652, w2646, w2616, w2614) -> (w2651:errorcluster)
        n1009 = property on="Refresh Button" class="Bool (strict)"() -> ("Value"=w2640:bool)  [unwired: 2 in, 2 out]
        n1010 = call <vilib>:"Clear Errors.vi"("error in (no error)"=w2651) -> ("error out"=w2650:errorcluster)  [unwired: 5 in, 1 out]
        n1011 = property on="Stop Button" class="Bool (strict)"() -> ("Value"=w2644:bool)  [unwired: 2 in, 2 out]
        n1012 = property on="ClosePanel" class="Bool (strict)"(error in=w2650) -> (error out=w2648:errorcluster, "Value"=w2649:bool)  [unwired: 1 in, 1 out]
        n1013 = Not(x=w2640) -> (.not. x?=w2641:bool)
        n1014 = Select(t=T4."Initialize", s=w2640, f=T4."Stop") -> (s? t:f=w2654:T4)
        n1015 = Not(x=w2644) -> (.not. x?=w2643:bool)
        n1016 = Compound Arithmetic op=AND(w2649, w2643, w2641) -> (w2645:bool)
        n1017 = case shown="False" w2645 {
          tunnel: w2648 -> [w2682 w2686]
          tunnel: [w2682 w2686] -> w2647
          tunnel: [w2681 w2685] -> w2642
          tunnel: w2640 -> [w2680 _]
          frame False {
            n1018 = case shown="False" w2680 {
              tunnel: [TRUE FALSE] -> w2681
              frame False {
              }
              frame True {
              }
            }
          }
          frame True {
            n1019 = flat-sequence {
              tunnel: [TRUE] -> w2685
              frame #0 {
              }
              frame #1 {
                n1020 = control-ref of="This VI"() -> (w2689:refnum<vi>)
                n1021 = property class="VI"(reference=w2689, "FP.State"=T15."Closed" ("Front Panel Window:State")) -> ()  [unwired: 1 in, 2 out]
              }
            }
          }
        }
      }
      frame "MainProgram" {
        n1022 = event shown="[0] Timeout" {
          selector: w2704 -> [_ _ _ _ _ _ _ _ _ _ _ _ _ _]
          dyn-events: _ -> [_ _ _ _ _ _ _ _ _ _ _ _ _ _]
          timeout: "EventTimeout" -> [_ _ _ _ _ _ _ _ _ _ _ _ _ _]
          tunnel: [T4."MainProgram" T4."MainProgram" T4."MainProgram" T4."MainProgram" T4."MainProgram" T4."MainProgram" T4."Stop" T4."MainProgram" w3123 T4."MainProgram" T4."MainProgram" T4."MainProgram" T4."Stop" T4."MainProgram"] -> w2717
          tunnel: [w2729 w2835 w2902 w2912 w2921 w2932 w2952 w2972 w3073 w3222 w3236 _ w3258 w3259] -> w2711
          tunnel: w2715 -> [w2734 w2835 w2901 w2912 w2923 w2932 w2952 _ w3073 w3211 w3235 w3243 w3258 w3259]
          tunnel: [w2726 w2849 w2903 w2913 w2922 w2933 w2950 w2964 w3128 w3220 w3233 _ w3256 w3263] -> w2712
          tunnel: w2713 -> [w2726 w2849 w2903 w2913 w2922 w2933 w2950 w2964 w3128 w3220 w3233 _ w3256 w3263]
          tunnel: w2710 -> [w2736 w2860 w2897 w2909 w2918 w2929 w2949 w2974 w3148 w3219 w3232 w3247 w3255 w3266]
          tunnel: w2709 -> [w2732 w2859 w2898 w2910 w2919 w2930 w2948 w2968 w3147 w3218 w3231 w3246 w3254 w3262]
          tunnel: [w2733 w2859 w2898 w2910 w2919 w2930 w2948 w2968 w3147 w3218 w3231 w3246 w3254 w3262] -> w2708
          tunnel: [w2735 w2860 w2897 w2909 w2918 w2929 w2949 w2974 w3148 w3219 w3232 w3247 w3255 w3266] -> w2707
          tunnel: w2706 -> [w2720 w2858 w2896 w2908 w2917 w2928 w2947 w2973 w3146 w3217 w3230 w3245 w3253 w3265]
          tunnel: [w2720 w2858 w2896 w2908 w2917 w2928 w2947 w2971 w3146 w3217 w3230 w3245 w3253 w3265] -> w2705
          tunnel: w2703 -> [_ _ _ _ _ _ _ _ w3106 _ _ _ _ _]
          tunnel: w2702 -> [w2731 w2857 w2895 w2907 w2916 w2927 w2945 w2969 w3132 w3216 w3229 w3244 w3252 w3264]
          tunnel: [w2731 w2857 w2895 w2907 w2916 w2927 w2945 w2969 w3131 w3216 w3229 w3244 w3252 w3264] -> w2701
          tunnel: w2700 -> [_ w2855 _ _ _ _ _ _ w3130 _ _ _ _ _]
          tunnel: w2699 -> [_ w2848 _ _ _ _ _ _ _ _ _ _ _ _]
          tunnel: w2698 -> [_ _ _ _ _ _ _ _ _ w3215 _ _ _ _]
          tunnel: w2697 -> [_ w2839 w2894 w2906 w2915 w2926 w2942 w2967 w3107 w3213 w3228 w3241 w3251 w3261]
          tunnel: [_ w2839 w2894 w2906 w2915 w2926 w2942 w2967 w3107 w3213 w3228 w3241 w3251 w3261] -> w2696
          tunnel: w2695 -> [w2728 w2838 w2893 w2905 w2914 w2925 w2941 w2966 w3101 w3212 w3227 w3240 w3250 w3260]
          tunnel: [w2727 w2838 w2893 w2905 w2914 w2925 w2941 w2966 w3101 w3212 w3227 w3240 w3250 w3260] -> w2694
          event Timeout {
            n1023 = event-data() -> ()  [unwired: 1 in, 3 out]
            n1024 = disable-structure shown="Enabled" {
              disable-tunnel: w2736 -> [w2758 w2818]
              disable-tunnel: [w2757 w2818] -> w2735
              disable-tunnel: w2734 -> [w2756 w2817]
              disable-tunnel: [w2755 w2815] -> w2733
              disable-tunnel: w2732 -> [w2754 w2815]
              disable-tunnel: [w2751 w2817] -> w2729
              disable-tunnel: w2728 -> [w2749 w2816]
              disable-tunnel: [w2748 w2816] -> w2727
              frame Disabled {
                n1025 = property class="Clust (strict)"(reference=w2754, error in=w2756) -> (reference out=w2755:refnum<vi>, error out=w2750:errorcluster, "Value"=w2761:T24)
                n1026 = Unbundle By Name(w2761) -> ("DevType"=w2762:T18, "CanIndex"=w2760:T19)
                n1027 = call "VCI_Receive.vi"("CANIndex"=w2760, "DevIndex"=u32 0, "DevType"=w2762) -> ("Recieve"=w2759:T25[])  [unwired: 3 in, 5 out]
                n1028 = Empty Array?(array=w2759) -> (empty?=w2753:bool)
                n1029 = case shown="False" w2753 {
                  tunnel: w2760 -> [w2776 _]
                  tunnel: w2755 -> [w2774 _]
                  tunnel: w2758 -> [w2773 w2806]
                  tunnel: w2750 -> [w2772 w2805]
                  tunnel: w2759 -> [w2777 _]
                  tunnel: [w2767 w2805] -> w2751
                  tunnel: [w2766 w2806] -> w2757
                  tunnel: [TRUE w2800] -> w2752
                  tunnel: w2749 -> [_ w2804]
                  tunnel: [0 w2803] -> w2748
                  frame False {
                    n1030 = call "Demo_MakeDispBuff.vi"("Channel"=w2776, "Type"=enum16{"接收", "发送"}."接收", "OBJs"=w2777) -> ("Buffer"=w2775:T26)
                    n1031 = for {
                      N: 3 -> [_]
                      tunnel: w2775 -> [w2791]
                      tunnel: w2774 -> [w2790]
                      tunnel: w2773 -> [w2781]
                      tunnel: w2772 -> [w2780]
                      tunnel: [w2783] -> w2770 mode=indexing
                      tunnel: [w2781] -> w2769
                      tunnel: [w2780] -> w2768
                      i -> [w2779]
                      n1032 = property class="Clust (strict)"(reference=w2790) -> ("Value"=w2788:T24)  [unwired: 1 in, 2 out]
                      n1033 = Index Array(array=w2791, index=w2779) -> (element=w2784:T27)
                      n1034 = Unbundle By Name(w2784) -> ("Channel"=w2786:T19, "VCI_CAN_OBJ"=w2789:T25)  [unwired: 2 out]
                      n1035 = Unbundle By Name(w2788) -> ("CanIndex"=w2787:T19)
                      n1036 = Equal?(x=w2787, y=w2786) -> (x = y?=w2785:bool)
                      n1037 = case shown="True" w2785 {
                        tunnel: w2789 -> [_ w2799]
                        tunnel: [w2792 w2795] -> w2783
                        tunnel: T16 {"ID"=0, "MSGTYPE"=0, "LEN"=0, "aDATA"=[]} ("Msg") -> [w2792 w2794]
                        frame False {
                        }
                        frame True {
                          n1038 = Unbundle By Name(w2799) -> ("ID"=w2793:u32, "DataLen"=w2798:u8, "Data"=w2796:u8[])
                          n1039 = Bundle By Name(cluster=w2794, "ID"=w2793, "MSGTYPE"=u8 0, "LEN"=w2798, "aDATA"=w2796) -> (w2795:T16)
                        }
                      }
                    }
                    n1040 = Enqueue Element(queue=w2769, element=w2770, error in (no error)=w2768) -> (queue out=w2766:refnum<queue>, error out=w2767:errorcluster)  [unwired: 2 out]
                  }
                  frame True {
                    n1041 = Increment(x=w2804) -> (x+1=w2803:i32)
                    n1042 = Greater Or Equal?(x=w2803, y=7) -> (x >= y?=w2801:bool)
                    n1043 = Not(x=w2801) -> (.not. x?=w2800:bool)
                  }
                }
                n1044 = property on="CAN Status" class="Bool (strict)"("Value"=w2752) -> ()  [unwired: 2 in, 2 out]
              }
              frame Enabled {
                n1045 = property on="VISA Current" class="VISAName"() -> ("Value"=w2809:refnum<visa-resource-name>)  [unwired: 2 in, 2 out]
                n1046 = Not Equal?(x=w2809, y=refnum<visa-resource-name> "COMx") -> (x != y?=w2810:bool)
                n1047 = case shown="True" w2810 {
                  tunnel: w2809 -> [_ w2819]
                  frame False {
                  }
                  frame True {
                    n1048 = call "ReadCurrent.vi"("LoopFromMain"=TRUE, "VISA resource name"=w2819) -> ("CurrentSens"=→"CurrentSens":bool, "CurrentOut"=w2827:string)  [unwired: 7 in, 1 out]
                    "Current" <- w2827
                    n1049 = Fract/Exp String To Number(string=w2827) -> (number=w2825:dbl)  [unwired: 3 in, 1 out]
                    "CurrentOut" <- w2825
                    n1050 = property on="Motor Speed RPM Serial" class="DigNum (strict)"() -> ("Value"=w2824:dbl)  [unwired: 2 in, 2 out]
                    n1051 = Equal To 0?(x=w2825) -> (x = 0?=w2821:bool)
                    n1052 = Greater Or Equal?(x=w2824, y=4000.0) -> (x >= y?=w2822:bool)
                    n1053 = And(x=w2822, y=w2821) -> (x .and. y?=w2820:bool)
                    n1054 = case shown="True" w2820 {
                      tunnel: w2819 -> [_ w2830]
                      frame False {
                      }
                      frame True {
                        n1055 = call "ReadCurrent.vi"("LoopFromMain"=FALSE, "VISA resource name"=w2830) -> ()  [unwired: 7 in, 3 out]
                      }
                    }
                  }
                }
                n1056 = property on="Automation" class="Bool (strict)"() -> ("Value"=w2814:bool)  [unwired: 2 in, 2 out]
                n1057 = property on="Start" class="Bool (strict)"() -> ("Value"=w2812:bool)  [unwired: 2 in, 2 out]
                n1058 = Or(x=w2814, y=w2812) -> (x .or. y?=w2813:bool)
                n1059 = control-ref of="ATR"() -> (w2807:refnum<vi>)
                n1060 = case shown="False" w2813 {
                  frame False {
                    n1061 = property on="Pannel User Message" class="Str"("Value"="You can press start to execute(s) test(s).") -> ()  [unwired: 2 in, 2 out]
                  }
                  frame True {
                  }
                }
                n1062 = call "PassFailUUT (SubVI).vi"("Table in"=w2807) -> ("PassFaileUUTresult"=w2808:bool)  [unwired: 8 in, 2 out]
                n1063 = property on="Test Failed" class="Bool (strict)"("Value"=w2808) -> ()  [unwired: 2 in, 2 out]
              }
            }
            n1064 = property on="ClosePanel" class="Bool (strict)"("Value"=FALSE ("ClosePanel")) -> ()  [unwired: 2 in, 2 out]
            n1065 = Not Equal?(x=w2726, y=refnum<visa-resource-name> "COMx") -> (x != y?=w2724:bool)
            n1066 = property on="Analogtest" class="Bool (strict)"() -> ("Value"=w2722:bool)  [unwired: 2 in, 2 out]
            n1067 = Not(x=w2722) -> (.not. x?=w2721:bool)
            n1068 = Get Queue Status(queue=w2720) -> (# elements in queue=w2719:i32)  [unwired: 2 in, 7 out]
            n1069 = And(x=w2721, y=w2724) -> (x .and. y?=w2723:bool)
            n1070 = case shown="True" w2723 {
              tunnel: w2726 -> [_ w2746]
              frame False {
              }
              frame True {
                n1071 = call "Serial.vi"("Clear Log"=FALSE, "write buffer"="VC\r\n", "VISA resource name"=w2746) -> ("read buffer"=w2740:string)  [unwired: 7 in, 1 out]
                n1072 = Fract/Exp String To Number(string=w2740) -> (number=→"Motor Speed RPM Serial":dbl)  [unwired: 3 in, 1 out]
                n1073 = Empty String/Path?(string/path=w2740) -> (empty?=w2742:bool)
                n1074 = Not(x=w2742) -> (.not. x?=w2741:bool)
                n1075 = disable-structure shown="Disabled" {
                  disable-tunnel: w2741 -> [w2747 _]
                  frame Disabled {
                    n1076 = property on="Serial Status" class="Bool (strict)"("Value"=w2747) -> ()  [unwired: 2 in, 2 out]
                  }
                  frame Enabled {
                  }
                }
              }
            }
            n1077 = case shown="0" w2719 {
              tunnel: [TRUE ("STDBY") FALSE ("STDBY")] -> w2718
              frame 0 {
              }
              frame 1, Default {
              }
            }
            n1078 = property on="STDBY" class="Bool (strict)"("Value"=w2718, "Blinking"=w2718) -> ()  [unwired: 2 in, 2 out]
          }
          event "SetSN": Value Change {
            w2834 = FALSE ("STDBY")
            n1079 = event-data() -> ()  [unwired: 1 in, 6 out]
            n1080 = property on="STDBY" class="Bool (strict)"(error in=w2835, "Value"=w2834, "Blinking"=w2834) -> ()  [unwired: 1 in, 2 out]
            n1081 = property on="Current SN" class="DigNum (strict)"(error in=w2835) -> (error out=w2841:errorcluster, "Value"=w2854:i32)  [unwired: 1 in, 1 out]
            n1082 = Equal To 0?(x=w2854) -> (x = 0?=w2851:bool)
            n1083 = Equal?(x=w2854, y=-1) -> (x = y?=w2852:bool)
            n1084 = Or(x=w2852, y=w2851) -> (x .or. y?=w2850:bool)
            n1085 = property on="UUT" class="Str"() -> ("Value"=w2833:string)  [unwired: 2 in, 2 out]
            n1086 = control-ref of="ATR"() -> (w2842:refnum<vi>)
            n1087 = case shown="\"BLDC 60A\"" w2833 {
              tunnel: [38 38 13 13 45] -> w2832
              frame "BLDC 30A", Default {
              }
              frame "Warrior 60A" {
              }
              frame "Condenser Merkava" {
              }
              frame "Condenser India" {
              }
              frame "BLDC 60A" {
              }
            }
            n1088 = call "PassFailUUT (SubVI).vi"("error in (no error)"=w2841, "Table in"=w2842) -> ("Total Pass"=w2837:i32)  [unwired: 7 in, 2 out]
            n1089 = Equal?(x=w2837, y=w2832) -> (x = y?=w2836:bool)
            n1090 = property on="CAN Status" class="Bool (strict)"() -> ("Value"=w2843:bool)  [unwired: 2 in, 2 out]
            n1091 = property on="Serial Status" class="Bool (strict)"() -> ("Value"=w2847:bool)  [unwired: 2 in, 2 out]
            n1092 = And(x=w2847, y=w2843) -> (x .and. y?=w2844:bool)
            n1093 = case shown="True" w2844 {
              tunnel: w2855 -> [_ w2879]
              tunnel: w2850 -> [_ w2868]
              tunnel: w2849 -> [_ w2878]
              tunnel: w2848 -> [_ w2877]
              tunnel: [errorcluster {"status"=FALSE, "code"=0, "source"=""} ("error out") w2876] -> w2846
              tunnel: w2836 -> [_ w2869]
              frame False {
                n1094 = property on="SetSN" class="Bool (strict)"("Value"=FALSE) -> ()  [unwired: 2 in, 2 out]
                n1095 = call "Display Message to User10"() -> ()  [unwired: 10 in, 2 out]
              }
              frame True {
                n1096 = property on="Test Failed" class="Bool (strict)"() -> ("Value"=w2873:bool)  [unwired: 2 in, 2 out]
                n1097 = property on="Automation" class="Bool (strict)"() -> ("Value"=w2875:bool)  [unwired: 2 in, 2 out]
                n1098 = Not(x=w2873) -> (.not. x?=w2874:bool)
                n1099 = Select(t=w2874, s=w2875, f=w2877) -> (s? t:f=w2871:bool)
                n1100 = Or(x=w2869, y=w2871) -> (x .or. y?=w2870:bool)
                n1101 = And(x=w2868, y=w2870) -> (x .and. y?=w2872:bool)
                n1102 = case shown="True" w2872 {
                  tunnel: w2879 -> [_ w2892]
                  tunnel: w2878 -> [_ w2891]
                  tunnel: [w2881 w2890] -> w2876
                  tunnel: w2868 -> [w2880 _]
                  frame False {
                    n1103 = case shown="False" w2880 {
                      tunnel: [w2883 w2884] -> w2881
                      frame False {
                        n1104 = call "Display Message to User9"() -> ("error out"=w2883:errorcluster)  [unwired: 10 in, 1 out]
                      }
                      frame True {
                        n1105 = call "Display Message to User3"() -> ("error out"=w2884:errorcluster)  [unwired: 10 in, 1 out]
                      }
                    }
                    n1106 = property on="Automation" class="Bool (strict)"(error in=w2881, "Value"=FALSE ("Automation")) -> ()  [unwired: 1 in, 2 out]
                  }
                  frame True {
                    n1107 = control-ref of="Current SN"() -> (w2887:refnum<vi>)
                    n1108 = control-ref of="UUT"() -> (w2886:refnum<vi>)
                    n1109 = local read "DAQmx Device Name"() -> (w2889:tag)
                    n1110 = control-ref of="Next SN"() -> (w2888:refnum<vi>)
                    n1111 = call "SetSN (SubVI).vi"("Kinetics Params"=w2892, "UUT"=w2886, "DAQmx Device Name"=w2889, "Current SN"=w2887, "VISA resource name"=w2891, "Next SN"=w2888) -> ("error out"=w2890:errorcluster, "UUT SN Report"=w2885:string)  [unwired: 4 in]
                    "UUT SN Report" <- w2885
                    n1112 = property on="UUT SN Report" class="Str"("Value"=w2885) -> ()  [unwired: 2 in, 2 out]
                  }
                }
              }
            }
            n1113 = call <vilib>:"Clear Errors.vi"("error in (no error)"=w2846) -> ("error out"=w2840:errorcluster)  [unwired: 5 in, 1 out]
            n1114 = property on="SetSN" class="Bool (strict)"(error in=w2840, "Value"=FALSE ("SetSN")) -> ()  [unwired: 1 in, 2 out]
          }
          event "ATR": Mouse Enter {
            n1115 = event-data() -> ()  [unwired: 1 in, 4 out]
            n1116 = call-poly <vilib>:"Set Cursor.vi"("error in (no error)"=w2901, "icon"=u16 1) -> ("error out"=w2902:errorcluster)  [unwired: 8 in, 1 out]
          }
          event "Stop Button": Value Change {
            n1117 = event-data() -> ()  [unwired: 1 in, 6 out]
            n1118 = property on="Stop Button" class="Bool (strict)"("Value"=FALSE ("Stop Button")) -> ()  [unwired: 2 in, 2 out]
          }
          event "ATR": Mouse Leave {
            n1119 = event-data() -> ()  [unwired: 1 in, 4 out]
            n1120 = call-poly <vilib>:"Set Cursor.vi"("error in (no error)"=w2923, "icon"=u16 0) -> ("error out"=w2921:errorcluster)  [unwired: 8 in, 1 out]
          }
          event "ATR": Mouse Down? {
            n1121 = event-data() -> ("Coords"=w2940:T28)  [unwired: 1 in, 4 out]
            n1122 = invoke on="ATR" class="Tbl (strict)" method="Point To Row Column"("Point"=w2940) -> ("InBounds"=w2936:bool, "CellPosition"=w2935:T14)  [unwired: 5 in, 4 out]
            n1123 = Greater Than 0?(x=w2935) -> (x > 0?=w2939:cluster{"Row":bool, "Column":bool})
            n1124 = Cluster To Array(cluster=w2939) -> (array=w2938:bool[])
            n1125 = Or Array Elements(Boolean array=w2938) -> (logical OR=w2937:bool)
            n1126 = Or(x=w2936, y=w2937) -> (x .or. y?=w2934:bool)
            n1127 = event-data("Discard?"=w2934) -> ()  [unwired: 1 in, 1 out]
          }
          event Panel Close? {
            n1128 = event-data() -> ("VIRef"=w2946:refnum<vi>)  [unwired: 1 in, 3 out]
            n1129 = Close Reference(reference=w2946) -> ()  [unwired: 1 in, 1 out]
            n1130 = disable-structure shown="Disabled" {
              frame Disabled {
                n1131 = property on="Stop Button" class="Bool (strict)"("Val(Sgnl)"=TRUE ("Stop Button"), "Value"=FALSE ("Stop Button")) -> ()  [unwired: 2 in, 2 out]
              }
              frame Enabled {
              }
            }
            n1132 = event-data("Discard?"=TRUE) -> ()  [unwired: 1 in, 1 out]
            "ClosePanel" <- TRUE ("ClosePanel")
          }
          event "Start": Value Change {
            w2958 = FALSE ("STDBY")
            (unwired) FALSE
            w2962 = string[] []  # TestArray
            n1133 = event-data() -> ()  [unwired: 1 in, 2 out]
            n1134 = property on="STDBY" class="Bool (strict)"("Value"=w2958, "Blinking"=w2958) -> (error out=w2959:errorcluster)  [unwired: 2 in, 1 out]
            n1135 = while {
              tunnel: [w3010] -> w2961
              tunnel: [w3009] -> w2957
              shift-right: [w3007] -> _
              shift-left: enum16{"Stop", "Tests", "Bit test", "Start"}."Start" -> [w3008]
              tunnel: w2962 -> [w3006]
              tunnel: w2959 -> [_]
              stop <- w3005 stop-if-true
              n1136 = case shown="\"Tests\"" w3008 {
                tunnel: [w3015 w3020 w3030 w3042] -> w3010
                tunnel: [errorcluster {"status"=FALSE, "code"=0, "source"=""} ("error out") w3019 errorcluster {"status"=FALSE, "code"=0, "source"=""} ("error out") w3040] -> w3009
                tunnel: [w3014 w3026 enum16{"Stop", "Tests", "Bit test", "Start"}."Stop" w3036] -> w3007
                tunnel: w3006 -> [w3015 _ w3030 w3042]
                tunnel: [w3013 w3025 FALSE FALSE] -> w3005
                frame "Stop", Default {
                  n1137 = flat-sequence {
                    tunnel: [enum16{"Stop", "Tests", "Bit test", "Start"}."Stop"] -> w3014
                    tunnel: [TRUE] -> w3013
                    frame #0 {
                    }
                  }
                  n1138 = property on="Start" class="Bool (strict)"("Value"=FALSE ("Start")) -> ()  [unwired: 2 in, 2 out]
                }
                frame "Tests" {
                  w3024 = T1."Disabled and Grayed Out" ("Disabled")
                  n1139 = property on="TestArray" class="Arr (strict)"() -> (error out=w3019:errorcluster, "Value"=w3021:string[])  [unwired: 2 in, 1 out]
                  n1140 = call "Start Test Selection (SubVI).vi"("TestArrayIn"=w3021) -> ("AutoOut"=w3018:bool, "TestArrayOut"=w3020:string[])  [unwired: 9 in]
                  "Automation" <- w3018
                  n1141 = property on="Start" class="Bool (strict)"("DisabledEnum"=w3024) -> ()  [unwired: 2 in, 2 out]
                  n1142 = property on="Report" class="Bool (strict)"("DisabledEnum"=w3024) -> ()  [unwired: 2 in, 2 out]
                  n1143 = control-ref of="ATR"() -> (w3022:refnum<vi>)
                  n1144 = property on="Stop Button" class="Bool (strict)"("Value"=FALSE ("Stop Burn-in")) -> ()  [unwired: 2 in, 2 out]
                  n1145 = case shown="True" w3018 {
                    tunnel: w3022 -> [_ w3027]
                    frame False {
                    }
                    frame True {
                      n1146 = call "ResetTable Result (SubVI).vi"("Table in"=w3027) -> ()  [unwired: 11 in]
                    }
                  }
                  n1147 = flat-sequence {
                    tunnel: [enum16{"Stop", "Tests", "Bit test", "Start"}."Tests"] -> w3026
                    tunnel: [TRUE] -> w3025
                    frame #0 {
                    }
                  }
                }
                frame "Bit test" {
                }
                frame "Start" {
                  n1148 = property on="CAN Status" class="Bool (strict)"() -> (error out=w3039:errorcluster, "Value"=w3038:bool)  [unwired: 2 in, 1 out]
                  n1149 = property on="CurrentSens" class="Bool (strict)"() -> ("Value"=w3034:bool)  [unwired: 2 in, 2 out]
                  n1150 = property on="Serial Status" class="Bool (strict)"(error in=w3039) -> ("Value"=w3037:bool)  [unwired: 1 in, 2 out]
                  n1151 = And(x=w3038, y=w3037) -> (x .and. y?=w3035:bool)
                  n1152 = case shown="True" w3035 {
                    tunnel: [w3044 w3047] -> w3040
                    tunnel: [enum16{"Stop", "Tests", "Bit test", "Start"}."Stop" w3046] -> w3036
                    tunnel: w3034 -> [_ w3045]
                    frame False {
                      n1153 = call "Display Message to User5"() -> ("error out"=w3044:errorcluster)  [unwired: 10 in, 1 out]
                    }
                    frame True {
                      n1154 = case shown="True" w3045 {
                        tunnel: [w3048 w3054] -> w3047
                        tunnel: [enum16{"Stop", "Tests", "Bit test", "Start"}."Stop" enum16{"Stop", "Tests", "Bit test", "Start"}."Tests"] -> w3046
                        frame False {
                          n1155 = call "Display Message to User"() -> ("error out"=w3048:errorcluster)  [unwired: 10 in, 1 out]
                        }
                        frame True {
                          n1156 = control-ref of="Motor Speed RPM Serial"() -> (w3051:refnum<vi>)
                          n1157 = control-ref of="Stop Button"() -> (w3052:refnum<vi>)
                          n1158 = control-ref of="Pannel User Message"() -> (w3053:refnum<vi>)
                          n1159 = call "Write panel message Kinetics (SubVI).vi"(4:"rpm"=w3051, 5:"rpm"=FALSE ("rpm"), "PrintTime"=FALSE, "Stop"=w3052, "Time to wait"=0.0, "Strin"="TESTER BIT TEST OPERATION IN PROCESS\nPlease wait...", "String in"=w3053) -> ("error out"=w3054:errorcluster)  [unwired: 2 in, 2 out]
                        }
                      }
                    }
                  }
                }
              }
            }
            n1160 = Array Size(array=w2961) -> (size(s)=w2960:i32)
            n1161 = case shown="1, Default" w2960 {
              tunnel: w2957 -> [w2998 w3000]
              tunnel: [w2998 w2999] -> w2956
              frame 0 {
              }
              frame 1, Default {
                n1162 = local read "DAQmx Device Name"() -> (w3004:tag)
                n1163 = call "Operation (SubVI).vi"("error in (no error)"=w3000, "On/Off"=TRUE, "Operation"=T6."PowerSuply", "DAQmx Device Name"=w3004) -> ("error out"=w3001:errorcluster)  [unwired: 7 in]
                n1164 = call "Time Delay"("error in (no error)"=w3001) -> ("error out"=w2999:errorcluster)  [unwired: 10 in]
              }
            }
            n1165 = disable-structure shown="Enabled" {
              disable-tunnel: w2956 -> [w2977 w2997]
              disable-tunnel: [w2976 w2997] -> w2955
              frame Disabled {
                n1166 = property on="Automation" class="Bool (strict)"(error in=w2977, "Value"=TRUE ("Automation")) -> (error out=w2978:errorcluster)  [unwired: 1 in, 1 out]
                n1167 = control-ref of="ATR"() -> (w2983:refnum<vi>)
                n1168 = property class="Tbl (strict)"(reference=w2983, error in=w2978) -> (reference out=w2979:refnum<vi>, "Value"=w2980:string[][])  [unwired: 1 out]
                n1169 = Index Array(array=w2980, index (col)=0 ("disabled index (col)")) -> (element=w2981:string[])  [unwired: 1 in]
                n1170 = for {
                  tunnel: w2981 -> [w2989] mode=indexing
                  tunnel: w2979 -> [w2991]
                  tunnel: [w2985] -> w2976
                  i -> [w2992]
                  w2988 = "." ("regular expression")
                  n1171 = Search and Replace String(input string=w2989, search string=w2988, replace string=w2988) -> (number of replacements=w2986:i32, error out=w2985:errorcluster)  [unwired: 5 in, 2 out]
                  n1172 = Not Equal?(x=w2986, y=0) -> (x != y?=w2990:bool)
                  n1173 = case shown="True" w2990 {
                    tunnel: w2992 -> [_ w2996]
                    tunnel: w2991 -> [_ w2994]
                    frame False {
                    }
                    frame True {
                      n1174 = call "InsertSingleData.vi"("String In"="PASS", "Col"=6, "Row"=w2996, "Table in"=w2994) -> ()  [unwired: 7 in, 1 out]
                    }
                  }
                }
              }
              frame Enabled {
              }
            }
            n1175 = Bundle By Name(cluster=T2 {"VISA"="COM1", "TestArray"=[]}, "VISA"=w2964, "TestArray"=w2961) -> (w2965:T2)
            n1176 = Enqueue Element(queue=w2973, element=w2965, error in (no error)=w2955) -> (queue out=w2971:refnum<queue>, error out=w2972:errorcluster)  [unwired: 2 out]
          }
          event "Report": Value Change {
            w3072 = FALSE ("STDBY")
            (unwired) FALSE
            w3059 = "Kinetics" ("section")
            w3109 = T29 1 items=["User Home"=0, "User Desktop"=1, "User Documents"=2, "User Application Data"=3, "User Preferences"=4, "User Temporary"=5, "Public Documents"=6, "Public Application Data"=7, "Public Preferences"=8, "Public Cache"=13, "System Core Libraries"=9, "System Installed Libraries"=10, "Application Files"=11, "Boot Volume Root"=12] ("system directory type")
            w3070 = FALSE ("Report")
            w3067 = "_"
            n1177 = event-data() -> ("CtlRef"=w3127:refnum<vi>)  [unwired: 1 in]
            n1178 = property on="STDBY" class="Bool (strict)"(error in=w3073, "Value"=w3072, "Blinking"=w3072) -> ()  [unwired: 1 in, 2 out]
            n1179 = local read "UUT"() -> (w3078:string)
            n1180 = call <vilib>:"Get System Directory.vi"("create directory if not found? (F)"=TRUE, "system directory type"=w3109) -> ("system directory"=w3108:path)  [unwired: 9 in]
            n1181 = Build Path(base path=w3108, name or relative path="KineticsReports") -> (appended path=w3157:path)
            n1182 = property on="CAN Status" class="Bool (strict)"() -> ("Value"=w3112:bool)  [unwired: 2 in, 2 out]
            n1183 = property on="Serial Status" class="Bool (strict)"() -> (error out=w3076:errorcluster, "Value"=w3113:bool)  [unwired: 2 in, 1 out]
            n1184 = call <vilib>:"Check if File or Folder Exists.vi"("path"=w3157) -> ("error out"=w3155:errorcluster, "file or folder exists?"=w3158:bool, "dup path"=w3156:path)  [unwired: 8 in]
            n1185 = To Upper Case(1:w3078) -> (0:w3079:string)
            n1186 = And(x=w3113, y=w3112) -> (x .and. y?=w3114:bool)
            n1187 = property on="UUT SN Report" class="Str"() -> ("Value"=w3075:string)  [unwired: 2 in, 2 out]
            n1188 = case shown="False" w3158 {
              tunnel: w3155 -> [w3207 w3208]
              tunnel: w3156 -> [w3206 w3209]
              tunnel: [w3205 w3209] -> w3111
              tunnel: [w3204 w3208] -> w3160
              frame False {
                n1189 = Create Folder(path (use dialog)=w3206, error in=w3207) -> (created path=w3205:path, error out=w3204:errorcluster)  [unwired: 1 in, 1 out]
              }
              frame True {
              }
            }
            n1190 = case shown="True" w3114 {
              tunnel: ["" ("read buffer") "" ("read buffer")] -> _
              tunnel: [w3166 w3168] -> w3104
              tunnel: w3128 -> [_ w3171]
              tunnel: [w3167 w3180] -> _
              tunnel: [w3167 w3170] -> _
              tunnel: [w3167 "" ("read buffer")] -> w3121
              frame False {
                w3167 = "N_A" ("read buffer")
                n1191 = property on="PN" class="Str"() -> ("Value"=w3165:string)  [unwired: 2 in, 2 out]
                n1192 = call "Build PN (SubVI).vi"("read buffer"=w3165) -> ("String"=w3166:string)  [unwired: 10 in]
              }
              frame True {
                n1193 = call "Serial.vi"("write buffer"="SN\r\n", "VISA resource name"=w3171) -> ("error out"=w3176:errorcluster, "read buffer"=w3178:string)  [unwired: 8 in]
                n1194 = Decimal String To Number(string=w3178) -> (number=w3177:i32)  [unwired: 2 in, 1 out]
                n1195 = Number To Decimal String(number=w3177, width (-)=i16 4) -> (decimal integer string=w3180:string)
                n1196 = call "Serial.vi"("error in (no error)"=w3176, "write buffer"="VR\r\n", "VISA resource name"=w3171) -> ("error out"=w3172:errorcluster, "read buffer"=w3170:string)  [unwired: 7 in]
                n1197 = call "Serial.vi"("error in (no error)"=w3172, "write buffer"="PN\r\n", "VISA resource name"=w3171) -> ()  [unwired: 7 in, 2 out]
                n1198 = property on="PN" class="Str"() -> ("Value"=w3169:string)  [unwired: 2 in, 2 out]
                n1199 = call "Build PN (SubVI).vi"("read buffer"=w3169) -> ("String"=w3168:string)  [unwired: 10 in]
              }
            }
            n1200 = Get Date/Time String(want seconds? (F)=TRUE) -> (date string=w3159:string)  [unwired: 2 in, 1 out]
            n1201 = call <vilib>:"Open Config Data.vi"("create file if necessary (T)"=FALSE, "configuration file path"=w3130) -> ("refnum"=w3137:T5)  [unwired: 1 in, 8 out]
            n1202 = call-poly <vilib>:"Read Key.vi"("section"=w3078, "key"="version", "refnum"=w3137) -> ("error out"=w3133:errorcluster, "value"=w3135:string, "refnum out"=w3134:T5)  [unwired: 5 in, 1 out]
            n1203 = property on="Logger Path" class="Path"(error in=w3160, "Value"=w3111, "StartPath"=w3111) -> (error out=w3140:errorcluster)  [unwired: 1 in, 1 out]
            n1204 = Search and Replace String(replace all?=TRUE ("replace all? (F)"), input string=w3159, search string="/") -> (result string=w3143:string)  [unwired: 5 in, 3 out]
            n1205 = call-poly <vilib>:"Read Key.vi"("section"=w3059, "error in (no error)"=w3133, "key"="Tester Software Ver", "refnum"=w3134) -> ("error out"=w3064:errorcluster, "value"=w3105:string, "refnum out"=w3066:T5)  [unwired: 4 in, 1 out]
            n1206 = property on="UUT SoftwareVer" class="Str"() -> ("Value"=w3074:string)  [unwired: 2 in, 2 out]
            n1207 = call-poly <vilib>:"Read Key.vi"("section"=w3059, "error in (no error)"=w3064, "key"="Tester Hardware Rev", "refnum"=w3066) -> ("error out"=w3061:errorcluster, "value"=w3060:string, "refnum out"=w3062:T5)  [unwired: 4 in, 1 out]
            n1208 = property on="POWER Board S/N" class="Str"() -> ("Value"=w3084:string)  [unwired: 2 in, 2 out]
            n1209 = Concatenate Strings("ATR" ("string"), w3067, w3075, w3067, w3143, ".docx" ("string")) -> (w3141:string)
            n1210 = call <vilib>:"Close Config Data.vi"("error in (no error)"=w3061, "refnum"=w3062) -> ()  [unwired: 8 in, 2 out]
            n1211 = Build Path(base path=w3111, name or relative path=w3141) -> (appended path=w3142:path)
            n1212 = property on="DSP Board S/N" class="Str"() -> ("Value"=w3083:string)  [unwired: 2 in, 2 out]
            n1213 = property on="ProductRev" class="Str"() -> ("Value"=w3071:string)  [unwired: 2 in, 2 out]
            n1214 = Concatenate Strings("  Rev-" ("string"), w3135) -> (w3129:string)
            n1215 = while {
              tunnel: w3141 -> [w3189]
              tunnel: w3111 -> [w3186]
              shift-right: [w3188] -> w3139
              shift-left: w3142 -> [w3187]
              shift-right: [w3184] -> w3131
              shift-left: w3132 -> [w3185]
              tunnel: w3140 -> [w3190]
              tunnel: [w3191] -> w3110
              stop <- w3183 continue-if-true
              n1216 = call <vilib>:"Check if File or Folder Exists.vi"("error in (no error)"=w3190, "path"=w3187) -> ("error out"=w3191:errorcluster, "file or folder exists?"=w3183:bool)  [unwired: 7 in, 1 out]
              n1217 = case shown="True" w3183 {
                tunnel: w3189 -> [_ w3203]
                tunnel: w3185 -> [_ w3195]
                tunnel: [w3193 w3200] -> w3188
                tunnel: w3187 -> [w3193 _]
                tunnel: w3186 -> [_ w3201]
                tunnel: [1 w3194] -> w3184
                frame False {
                }
                frame True {
                  w3196 = ".docx" ("search string")
                  n1218 = Search and Replace String(input string=w3203, search string=w3196) -> (result string=w3202:string)  [unwired: 6 in, 3 out]
                  n1219 = Number To Decimal String(number=w3195) -> (decimal integer string=w3198:string)  [unwired: 1 in]
                  n1220 = call <vilib>:"Space Constant.vi"() -> ("String"=w3197:string)
                  n1221 = Concatenate Strings(w3202, w3197, w3198, w3196) -> (w3199:string)
                  n1222 = Build Path(base path=w3201, name or relative path=w3199) -> (appended path=w3200:path)
                  n1223 = Increment(x=w3195) -> (x+1=w3194:i32)
                }
              }
            }
            n1224 = property on="ParamVersion" class="Str"() -> ("Value"=w3082:string)  [unwired: 2 in, 2 out]
            n1225 = call "HeaderBis.vi"("UUTHeader"=w3079, "P/N UUT"=w3104, "Tester HW"=w3060, "DSP SN"=w3083, "Driver S/N"=w3075, "Product Rev"=w3071, "VR"=w3074, "POWER SN"=w3084, "Oper."=w3106, "Revision Param"=w3082, "Tester Software Ver"=w3105) -> ("table header"=w3103:string, "Array"=w3102:string[][])  [unwired: 6 in, 1 out]
            n1226 = Open/Create/Replace File(file path (use dialog)=w3139, error in=w3110, operation (0:open)=T17."create") -> (error out=w3150:errorcluster)  [unwired: 3 in, 2 out]
            n1227 = control-ref of="ATR"() -> (w3162:refnum<vi>)
            n1228 = property class="Bool (strict)"(reference=w3127, error in=w3076) -> ("BoolText.Text"=w3126:string)  [unwired: 2 out]
            n1229 = property class="Tbl (strict)"(reference=w3162, error in=w3150) -> ("Value"=w3163:string[][])  [unwired: 2 out]
            n1230 = control-ref of="ATR"() -> (w3095:refnum<vi>)
            n1231 = call "PassFailUUT (SubVI).vi"("Table in"=w3095) -> ("PassFaileUUTresult"=w3088:bool)  [unwired: 8 in, 2 out]
            n1232 = Equal?(x=w3126, y="Report") -> (x = y?=w3120:bool)
            n1233 = property on="Test Failed" class="Bool (strict)"("Value"=w3088) -> ()  [unwired: 2 in, 2 out]
            n1234 = property on="PN" class="Str"() -> ("Value"=w3080:string)  [unwired: 2 in, 2 out]
            n1235 = Select(t=T4."MainProgram", s=w3120, f=T4."MainProgram") -> (s? t:f=w3123:T4)
            n1236 = call "MarvinReport.vi"("HEADER1"=w3103, "ATR Or"=w3162, "Steps   pfull"=w3163, "Footer UUT"=w3121, "pageNum"=3, "InputHeaderArray"=w3102, "FILE NAME"=w3141, "Report Folder"=w3139, "PN"=w3080, "REV"=w3129, "Test-Conductor"=w3106) -> ("error out"=w3116:errorcluster)  [unwired: 3 in, 1 out]
            n1237 = Select(t="PASS" ("name or relative path"), s=w3088, f="FAIL" ("name or relative path")) -> (s? t:f=w3087:string)
            n1238 = call <vilib>:"Clear Errors.vi"("error in (no error)"=w3116) -> ("error out"=w3115:errorcluster)  [unwired: 5 in, 1 out]
            n1239 = call <vilib>:"Application Directory.vi"() -> ("Application Directory"=w3091:path)
            n1240 = Build Path(base path=w3091, name or relative path="data\\TestResult.ini") -> (appended path=w3094:path)
            n1241 = Select(t="Save Report...", s=w3120, f="Program Stopped...\r\nPlease turn OFF All Power sinks") -> (s? t:f=w3118:string)
            n1242 = property on="Report" class="Bool (strict)"(error in=w3115, "Value"=w3070) -> (error out=w3081:errorcluster)  [unwired: 1 in, 1 out]
            n1243 = call <vilib>:"Open Config Data.vi"("configuration file path"=w3094) -> ("error out"=w3092:errorcluster, "refnum"=w3093:T5)  [unwired: 2 in, 7 out]
            n1244 = property on="Stop Button" class="Bool (strict)"(error in=w3081, "Value"=w3070) -> (error out=w3069:errorcluster)  [unwired: 1 in, 1 out]
            n1245 = property on="Pannel User Message" class="Str"("Value"=w3118) -> ()  [unwired: 2 in, 2 out]
            n1246 = call-poly <vilib>:"Write Key.vi"("section"="Kinetics", "error in (no error)"=w3092, "value"=w3087, "key"="Result", "refnum"=w3093) -> ("error out"=w3090:errorcluster, "refnum out"=w3089:T5)  [unwired: 4 in, 1 out]
            n1247 = property on="Automation" class="Bool (strict)"(error in=w3069, "Value"=w3070) -> (error out=w3068:errorcluster)  [unwired: 1 in, 1 out]
            n1248 = call <vilib>:"Close Config Data.vi"("error in (no error)"=w3090, "refnum"=w3089) -> ()  [unwired: 8 in, 2 out]
            n1249 = property on="Pannel User Message" class="Str"(error in=w3068, "Value"="You can press start to execute(s) test(s)." ("Pannel User Message")) -> ()  [unwired: 1 in, 2 out]
          }
          event "Help Button": Value Change {
            w3210 = FALSE ("STDBY")
            n1250 = event-data() -> ()  [unwired: 1 in, 6 out]
            n1251 = vi-ref "Help.vi"() -> (w3224:refnum<vi>)
            n1252 = property on="STDBY" class="Bool (strict)"(error in=w3211, "Value"=w3210, "Blinking"=w3210) -> ()  [unwired: 1 in, 2 out]
            n1253 = invoke class="VI" method="FP.Open"(reference=w3224, error in=w3211, "Activate"=TRUE ("Activate?"), "State"=T15."Standard") -> (error out=w3223:errorcluster)  [unwired: 1 in, 4 out]
            n1254 = call "Help.vi"("error in"=w3223, "TesterSWVersion"=w3215) -> ("error out"=w3222:errorcluster)  [unwired: 6 in]
            n1255 = property on="Help Button" class="Bool (strict)"("Value"=FALSE ("Help Button")) -> ()  [unwired: 2 in, 2 out]
          }
          event "Serial Com": Value Change {
            n1256 = event-data() -> ()  [unwired: 1 in, 6 out]
            n1257 = property on="Serial Com" class="Bool"(error in=w3235, "Visible"=FALSE) -> (error out=w3239:errorcluster)  [unwired: 1 in, 1 out]
            n1258 = property on="VISA Kinetics" class="VISAName"(error in=w3239, "Visible"=TRUE) -> (error out=w3236:errorcluster)  [unwired: 1 in, 1 out]
          }
          event "VISA Kinetics": Value Change {
            n1259 = event-data() -> ()  [unwired: 1 in, 6 out]
            n1260 = property on="Serial Com" class="Bool"(error in=w3243, "Visible"=FALSE) -> ()  [unwired: 1 in, 2 out]
            n1261 = property on="Pannel User Message" class="Str"(error in=w3243, "Value"="Serial connection in process" ("Pannel User Message")) -> ()  [unwired: 1 in, 2 out]
          }
          event "Refresh Button": Value Change {
            n1262 = event-data() -> ()  [unwired: 1 in, 6 out]
          }
          event "Settings": Value Change {
            n1263 = event-data() -> ()  [unwired: 1 in, 6 out]
          }
        }
      }
      frame "Initialize" {
        w3268 = FALSE ("STDBY")
        w3288 = 0
        w3290 = FALSE ("Visible")
        w3292 = FALSE ("Visible")
        w3276 = refnum<visa-resource-name> "COMx" ("VISA resource name")
        w3280 = FALSE ("Serial Status")
        n1264 = property on="EventTimeout" class="DigNum (strict)"(error in=errorcluster {"status"=FALSE, "code"=0, "source"=""} ("error out"), "Value"=100 ("EventTimeout")) -> (error out=w3283:errorcluster)  [unwired: 1 in, 1 out]
        n1265 = property on="ComTestResult" class="Bool (strict)"("Value"=w3292) -> ()  [unwired: 2 in, 2 out]
        n1266 = property on="VenableResult" class="Bool (strict)"("Value"=w3292) -> ()  [unwired: 2 in, 2 out]
        n1267 = property on="VenableDirectionResult" class="Bool (strict)"("Value"=w3292) -> ()  [unwired: 2 in, 2 out]
        n1268 = property on="Serial Com" class="Bool"(error in=w3283, "Visible"=FALSE) -> (error out=w3298:errorcluster)  [unwired: 1 in, 1 out]
        n1269 = property on="VisualInspectionResult" class="Bool (strict)"("Value"=FALSE ("Visible")) -> ()  [unwired: 2 in, 2 out]
        n1270 = property on="VISA Kinetics" class="VISAName"(error in=w3298, "Visible"=FALSE, "Value"=w3276) -> (error out=w3269:errorcluster)  [unwired: 1 in, 1 out]
        n1271 = property on="Analogtest" class="Bool (strict)"("Value"=w3280) -> ()  [unwired: 2 in, 2 out]
        n1272 = property on="STDBY" class="Bool (strict)"(error in=w3269, "Value"=w3268, "Blinking"=w3268) -> ()  [unwired: 1 in, 2 out]
        n1273 = property on="Serial Status" class="Bool (strict)"("Value"=w3280) -> ()  [unwired: 2 in, 2 out]
        n1274 = property on="Refresh Button" class="Bool (strict)"(error in=w3269, "Value"=FALSE ("Refresh Button")) -> (error out=w3285:errorcluster)  [unwired: 1 in, 1 out]
        n1275 = property on="MotorTempResult" class="Bool (strict)"("Value"=w3290) -> ()  [unwired: 2 in, 2 out]
        n1276 = property on="Automation" class="Bool (strict)"("Value"=w3290) -> ()  [unwired: 2 in, 2 out]
        n1277 = call "Find DAQ Devices.vi"("Error In"=w3285) -> ("Error Out"=w3287:errorcluster, "Stop?"=w3279:bool, "DAQmx Device Name"=w3284:tag)  [unwired: 8 in]
        n1278 = case shown="False" w3279 {
          selector: w3279 -> [_ w3318]
          tunnel: w3287 -> [w3310 w3320]
          tunnel: [w3302 w3320] -> w3277
          tunnel: w3284 -> [w3301 _]
          tunnel: [T4."Erase ATR Table" T4."Stop"] -> w3278
          frame False {
            n1279 = call <vilib>:"Clear Errors.vi"("error in (no error)"=w3310) -> ("error out"=w3309:errorcluster)  [unwired: 5 in, 1 out]
            n1280 = Not Equal?(x=w3301, y=tag "") -> (x != y?=w3311:bool)
            n1281 = case shown="True" w3311 {
              tunnel: w3301 -> [_ w3317]
              tunnel: w3309 -> [w3313 w3316]
              tunnel: [w3313 w3315] -> w3308
              frame False {
              }
              frame True {
                n1282 = call "Operation (SubVI).vi"("error in (no error)"=w3316, "Operation"=T6."Init", "DAQmx Device Name"=w3317) -> ("error out"=w3315:errorcluster)  [unwired: 8 in]
              }
            }
            n1283 = call "Operation (SubVI).vi"("error in (no error)"=w3308, "On/Off"=TRUE, "Operation"=T6."0 ohm", "DAQmx Device Name"=w3301) -> ("error out"=w3303:errorcluster)  [unwired: 7 in]
            n1284 = call "Operation (SubVI).vi"("error in (no error)"=w3303, "On/Off"=TRUE, "Operation"=T6."PowerSuply", "DAQmx Device Name"=w3301) -> ("error out"=w3302:errorcluster)  [unwired: 7 in]
            "DAQmx Device Name" <- w3301
          }
          frame True {
            n1285 = Stop(stop? (T)=w3318) -> ()
          }
        }
        n1286 = call "COM Curent Read.vi"("error in (no error)"=w3277, "VISA resource name 2"=w3276) -> ("error out"=w3274:errorcluster, "VISA Current"=w3273:refnum<visa-resource-name>)  [unwired: 7 in, 1 out]
        "VISA Current" <- w3273
        n1287 = call "ReadCurrent.vi"("error in (no error)"=w3274, "LoopFromMain"=TRUE, "VISA resource name"=w3273) -> ("error out"=w3271:errorcluster, "CurrentSens"=w3272:bool, "CurrentOut"=w3270:string)  [unwired: 6 in]
        n1288 = property on="CurrentSens" class="Bool (strict)"("Value"=w3272) -> ()  [unwired: 2 in, 2 out]
        n1289 = property on="Current" class="Str"("Value"=w3270) -> ()  [unwired: 2 in, 2 out]
        "Test Failed" <- w3280
      }
    }
    "G.Stop" <- w2434
  }
  n1290 = call "ATRBuild.vi"() -> ()  [unwired: 9 in, 3 out]
  n1291 = property on="AO[1]" class="Str"("Visible"=w1) -> ()  [unwired: 2 in, 2 out]
  n1292 = property on="AO[0]" class="DigNum (strict)"("Visible"=w1) -> ()  [unwired: 2 in, 2 out]
  n1293 = property on="RO[1]" class="Str"("Visible"=w1) -> ()  [unwired: 2 in, 2 out]
  n1294 = property on="CC" class="DigNum (strict)"("Visible"=w1) -> ()  [unwired: 2 in, 2 out]
  n1295 = disable-structure shown="Disabled" {
    frame Disabled {
      n1296 = case shown="\"BLDC 30A\", Default" {
        selector: _ -> [_ _ _ _ _]
        tunnel: [26 26 26 26 35] -> _
        frame "BLDC 30A", Default {
        }
        frame "Warrior 60A" {
        }
        frame "Condenser Merkava" {
        }
        frame "Condenser India" {
        }
        frame "BLDC 60A" {
        }
      }
    }
    frame Enabled {
    }
  }
  n1297 = disable-structure shown="Disabled" {
    frame Disabled {
      n1298 = control-ref of="Stop Button"() -> ()  [unwired: 1 out]
      n1299 = control-ref of="UUT"() -> ()  [unwired: 1 out]
      n1300 = property on="UUT" class="Str" props=["Value"]() -> ()  [unwired: 2 in, 3 out]
      n1301 = control-ref of="UUT"() -> ()  [unwired: 1 out]
      n1302 = property on="UUT" class="DigNum (strict)" props=["Value"]() -> ()  [unwired: 2 in, 3 out]
      n1303 = control-ref of="Motor Speed RPM Serial"() -> ()  [unwired: 1 out]
      n1304 = call "Find_Number_LineMARVIN.vi"() -> ()  [unwired: 5 in, 4 out]
      n1305 = control-ref of="Pannel User Message"() -> ()  [unwired: 1 out]
      n1306 = call "Write panel message Kinetics (SubVI).vi"() -> ()  [unwired: 9 in, 3 out]
      n1307 = local read "DAQmx Device Name"() -> (w3327:tag)
      n1308 = control-ref of="ATR"() -> ()  [unwired: 1 out]
      n1309 = call "PassOrFail (SubVI).vi"() -> ()  [unwired: 11 in, 1 out]
      n1310 = call "Serial.vi"("write buffer"="EP=1\r\nVC=1000\r\n") -> ()  [unwired: 9 in, 2 out]
      n1311 = call "Operation (SubVI).vi"("DAQmx Device Name"=w3327) -> ()  [unwired: 10 in, 1 out]
      n1312 = property on="UUT" class="Str" props=["Value"]() -> ()  [unwired: 2 in, 3 out]
    }
    frame Enabled {
    }
  }
  n1313 = disable-structure shown="Disabled" {
    frame Disabled {
      w3328 = T1."Disabled and Grayed Out" ("Disabled")
      w3329 = FALSE ("Start")
      n1314 = property on="Current SN" class="DigNum (strict)" props=["Value"]() -> ()  [unwired: 2 in, 3 out]
      n1315 = property on="UUT" class="DigNum (strict)" props=["Value"]() -> ()  [unwired: 2 in, 3 out]
      n1316 = property on="Serial Status" class="Bool (strict)" props=["Value"]() -> ()  [unwired: 2 in, 3 out]
      n1317 = property on="UUT SoftwareVer" class="Str" props=["Value"]() -> ()  [unwired: 2 in, 3 out]
      n1318 = call "Operation (SubVI).vi"() -> ()  [unwired: 11 in, 1 out]
      n1319 = property on="Next SN" class="DigNum (strict)" props=["Value"]() -> ()  [unwired: 3 in, 2 out]
      n1320 = property on="Start" class="Bool (strict)"("Value"=w3329, "DisabledEnum"=w3328) -> ()  [unwired: 2 in, 2 out]
      n1321 = property on="Report" class="Bool (strict)"("Value"=w3329, "DisabledEnum"=w3328) -> ()  [unwired: 2 in, 2 out]
    }
    frame Enabled {
    }
  }
  n1322 = Stop(stop? (T)=w7) -> ()
  "Pannel User Message" <- w23
